vi "multipatch_states_V0.030_dualWCedits.vi"(0 "common cluster":T11, 1 "images":T8, 2 "allMainVIcontrols":refnum<vi>, 3 "which manipulator":T5(ring), 5 "individual controls in":T10, 7 "state in":T3=enum."Setting defaults...", 9 "cam size":i32[](array[numeric]), 11 "error in":errorcluster, 12 "time in":timestamp, 13 "mainVIpath":path) -> (15 "error out":errorcluster)   [LabVIEW 2015]
uses:
  controls/user_message_v6.ctl
  machine_vision/controls/approach_type.ctl
  controls/scope_motion.ctl
  multiBot/patcherBot/AxMultiClampMsg.dll
  whole_cell_protocol/Controls/Data.ctl
  pipette cleaning/pressure box/cleaning_soft/controls/arduino_pressure_setting.ctl
  controls/memtest_def.ctl
  <vilib>/vision/Image Controls.llb/IMAQ Image.ctl
  controls/images_controls.ctl
  controls/multipatch_common_controls_v4.ctl
  controls/multipatch_individual_controls_v5.ctl
  pipette cleaning/pressure box/cleaning_soft/controls/actuator_type.ctl
  pipette cleaning/pressure box/cleaning_soft/controls/actuator_cluster.ctl
  machine_vision/coordinate model vis/transform_properties_actuators.ctl
  machine_vision/controls/transform_cluster_actuator.ctl
  pipette cleaning/pressure box/cleaning_soft/controls/pressure_box_type.ctl
  pipette cleaning/pressure box/cleaning_soft/controls/pressure_box_control.ctl
  controls/NH_method.ctl
panel:
  out "cell number when cleaning fail 2":i32
  in  "protocol 2":enum16{"clean", "sham"}(ring)
  in  "Cleaning step (time [s], value [mBar]) actual 2":dbl[][](array[numeric])=[[3.0, -345.0], [1.0, -345.0], [1.0, 1000.0], [1.0, -345.0], [1.0, 1000.0], [1.0, -345.0], [1.0, 1000.0], [1.0, -345.0], [1.0, 1000.0], [5.0, 1000.0]]
  in  "Wash step (time [s], value [mBar]) actual 2":dbl[][](array[numeric])=[[2.0, -345.0], [10.0, 1000.0]]
  out "ValidationOutputCluster":T1(array[cluster])
  out "ValidationWaveform":waveform(dbl)[](array[waveform])
  out "ValidationPos2":T2(array[ring])
  out "ValidationPos1":T2(array[ring])
  out "ValidationResults":waveform(dbl)[][](array[waveform])
  in  "debug state":T3=enum."Detecting cell..."
  out "exit trigger":bool
  in  "Tab Control":T4(tab)
  out "max steps to take":i32
  in  "long wc protocol?":bool
  in  "GS memtest inputs":T6={"Samples to Read"=2000, "Rate (Hz)"=20000.0, "Amplitude (mV/pA)"=10.0, "Offset (mV/pA)"=0.0, "Frequency (Hz)"=10.0, "duty cycle (%)"=50.0, "phase"=0.0} {"phase" format="%.2p"; "duty cycle (%)" format="%0.2f"}
  in  "cell tracker movement options":T7={"step down by (steps)"=10.0, "descend threshold diam (px)"=30.0, "step XY by (steps)"=10.0} {"descend threshold diam (px)" format="%#_13g"; "step down by (steps)" format="%#_13g"}
  out "rel move vector (steps)":dbl[](array[numeric])
  in  "Wash step (time [s], value [mBar]) actual":dbl[][](array[numeric])=[[2.0, -345.0], [10.0, 1000.0]]
  in  "Cleaning step (time [s], value [mBar]) actual":dbl[][](array[numeric])=[[3.0, -345.0], [1.0, -345.0], [1.0, 1000.0], [1.0, -345.0], [1.0, 1000.0], [1.0, -345.0], [1.0, 1000.0], [1.0, -345.0], [1.0, 1000.0], [5.0, 1000.0]]
  in  "protocol":enum16{"clean", "sham"}(ring)
  out "cell number when cleaning fail":i32
  in  "give a zap?":i32[](array[numeric])=[0, 0, 1, 0, 1, 0, 0, 1, 0, 0, 1, 0, 1, 1]
  in  "Breakin num pulses":i32[](array[numeric])=[1, 1, 1, 1, 1, 1, 1, 1, 1, 1, 1, 1, 1, 1]
  in  "Breakin durations (ms)":i32[](array[numeric])=[0, 50, 50, 100, 100, 100, 200, 200, 200, 400, 500, 700, 1000, 1000]
  out "slow comp (pF)":dbl
  out "fast comp (pF)":dbl
  out "set pressure":dbl
  in  "AO physical channels":tag="Dev1/ao0:1"
  in  "AI Physical Channel":tag="Dev1/ai0:2, Dev1/ai10"
  out "state out":T3=enum."Setting defaults..."
  # "REENTRANT!!"
  # "VERSION CONTROL\n6/23/17\nmultiBot v0.007 is compatible with multipatch_states_v0.007\n- cell tracker working great\n- latest stable version for SINGLE-PATCH image tracking in slices\nmultiBot v0.006_reentrants is compatible with multipatch_states_wrapper_v0.001\nmultiBot v0.005 is compatible with multipatch_states_v0.005\nmultiBot v0.004 is compatible with multipatch_states_v0.004"
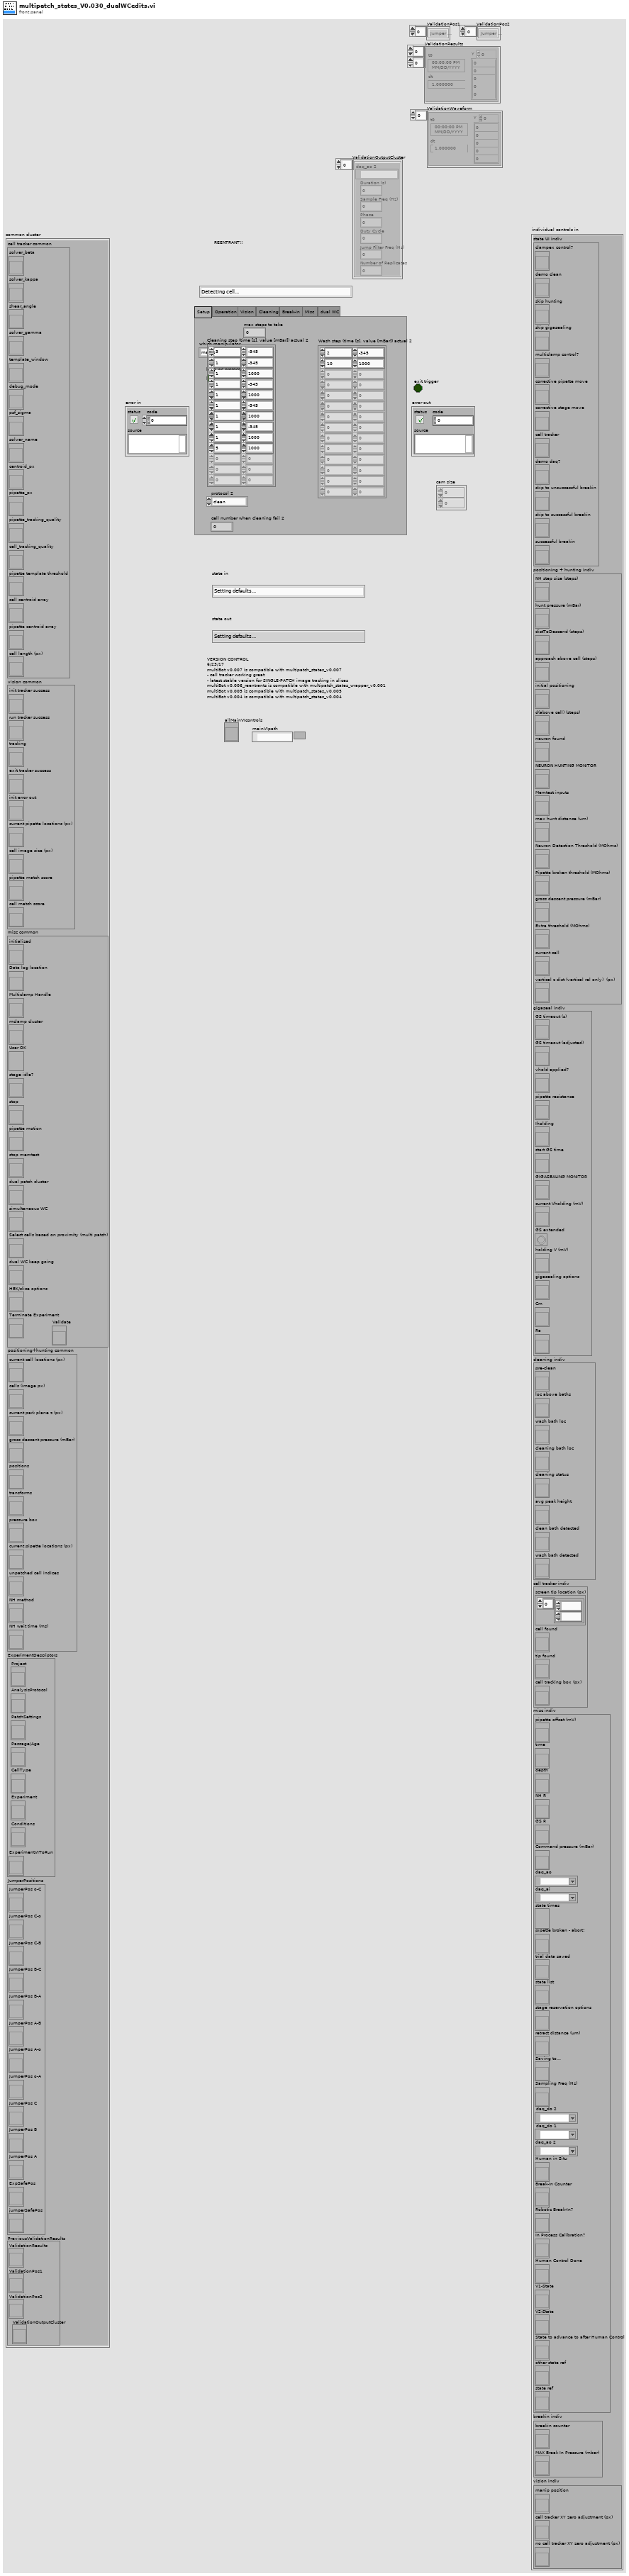
[diagram p1: front panel]
types:
  T1 = cluster{"daq_ao 2":tag, "Duration (s)":dbl, "Sample Freq (Hz)":dbl, "Phase":dbl, "Duty Cycle":dbl, "Jump Filter Freq (Hz)":dbl, "Number of Replicates":i16}[]
  T2 = enum16{"Jumper Safe Position", "Experiment Safe Position", "Jumper Position A", "Jumper Position B", "Jumper Position C", "Jumper Position o-A", "Jumper Position A-o", "Jumper Position A-B", "Jumper Position B-A", "Jumper Position B-C", "Jumper Position C-B", "Jumper Position C-o", "Jumper Position o-C"}[]
  T3 = typedef "user_message_v6.ctl" = enum16{"Initializing...", "Setting defaults...", "Click OK to start patcherBot!", "Starting new attempt...", "Pipette repositioning...", "Initializing cell tracker...", "Gross approach...", "Human Positioning...", "In Process Calibration", "Detecting cell...", "Cell detected...", "Gigaseal Established...", "Breaking in...", "Successful breakin!", "Unsuccessful breakin!", "Whole-cell recording", "Saving autopatching parameters...", "Quitting VI", "Waiting for idle stage...", "Cleaning...", "Retracting pipette...", "DEBUG STATE", "Waiting to break in...", "Waiting for WC", "reclean", "Done with Current Set of Cells"}
  T4 = enum32{"Setup", "Operation", "Vision", "Cleaning", "Break-in", "Misc", "dual WC"}
  T5 = enum16{"manipulator 1", "manipulator 2", "manipulator 3", "manipulator 4"}
  T6 = typedef "memtest_def.ctl" = cluster{"Samples to Read":i32, "Rate (Hz)":dbl, "Amplitude (mV/pA)":dbl, "Offset (mV/pA)":dbl, "Frequency (Hz)":dbl, "duty cycle (%)":dbl, "phase":dbl}
  T7 = cluster{"step down by (steps)":dbl, "descend threshold diam (px)":dbl, "step XY by (steps)":dbl}
  T8 = typedef "images_controls.ctl" = cluster{"slice image":T9, "pipette template":T9, "found pipette":T9, "pipette mask for cell tracker":T9, "cell images ref":refnum<vi>}
  T9 = typedef "IMAQ Image.ctl" = refnum<image>
  T10 = typedef "multipatch_individual_controls_v5.ctl" = cluster{"state UI indiv":cluster{"clampex control?":refnum<vi>, "demo clean":refnum<vi>, "skip hunting":refnum<vi>, "skip gigasealing":refnum<vi>, "multiclamp control?":refnum<vi>, "corrective pipette move":refnum<vi>, "corrective stage move":refnum<vi>, "cell tracker":refnum<vi>, "demo daq?":refnum<vi>, "skip to unsuccessful breakin":refnum<vi>, "skip to successful breakin":refnum<vi>, "successful breakin":refnum<vi>}, "positioning + hunting indiv":cluster{"NH step size (steps)":refnum<vi>, "hunt pressure (mBar)":refnum<vi>, "distToDescend (steps)":refnum<vi>, "approach above cell (steps)":refnum<vi>, "initial positioning":refnum<vi>, "d(above cell) (steps)":refnum<vi>, "neuron found":refnum<vi>, "NEURON HUNTING MONITOR":refnum<vi>, "Memtest inputs":refnum<vi>, "max hunt distance (um)":refnum<vi>, "Neuron Detection Threshold (MOhms)":refnum<vi>, "Pipette broken threshold (MOhms)":refnum<vi>, "gross descent pressure (mBar)":refnum<vi>, "Extra threshold (MOhms)":refnum<vi>, "current cell":refnum<vi>, "vertical z dist (vertical rel only)  (px)":refnum<vi>}, "gigaseal indiv":cluster{"GS timeout (s)":refnum<vi>, "GS timeout (adjusted)":refnum<vi>, "vhold applied?":refnum<vi>, "pipette resistance":refnum<vi>, "Iholding":refnum<vi>, "start GS time":refnum<vi>, "GIGASEALING MONITOR":refnum<vi>, "current Vholding (mV)":refnum<vi>, "GS extended":refnum<vi>, "holding V (mV)":refnum<vi>, "gigasealing options":refnum<vi>, "Cm":refnum<vi>, "Ra ":refnum<vi>}, "cleaning indiv":cluster{"pre-clean":refnum<vi>, "loc above baths":refnum<vi>, "wash bath loc":refnum<vi>, "cleaning bath loc":refnum<vi>, "cleaning status":refnum<vi>, "avg peak height":refnum<vi>, "clean bath detected":refnum<vi>, "wash bath detected":refnum<vi>}, "cell tracker indiv":cluster{"screen tip location (px)":refnum<vi>, "cell found":refnum<vi>, "tip found":refnum<vi>, "cell tracking box (px)":refnum<vi>}, "misc indiv":cluster{"pipette offset (mV)":refnum<vi>, "time":refnum<vi>, "depth":refnum<vi>, "NH R":refnum<vi>, "GS R":refnum<vi>, "Command pressure (mBar)":refnum<vi>, "daq_ao":tag, "daq_ai":tag, "state times":refnum<vi>, "pipette broken - abort!":refnum<vi>, "trial data saved":refnum<vi>, "state list":refnum<vi>, "stage reservation options":refnum<vi>, "retract distance (um)":refnum<vi>, "Saving to...":refnum<vi>, "Sampling Freq (Hz)":refnum<vi>, "daq_do 2":tag, "daq_do 1":tag, "daq_ao 2":tag, "Human in Situ":refnum<vi>, "Break-In Counter":refnum<vi>, "Robotic Break-In?":refnum<vi>, "In Process Calibration?":refnum<vi>, "Human Control Done":refnum<vi>, "V1-State":refnum<vi>, "V2-State":refnum<vi>, "State to advance to after Human Control":refnum<vi>, "other state ref":refnum<vi>, "state ref":refnum<vi>}, "breakin indiv":cluster{"breakin counter":refnum<vi>, "MAX Break In Pressure (mbar)":refnum<vi>}, "vision indiv":cluster{"manip position":refnum<vi>, "cell tracker XY zero adjustment (px)":refnum<vi>, "no cell tracker XY zero adjustment (px)":refnum<vi>}}
  T11 = typedef "multipatch_common_controls_v4.ctl" = cluster{"cell tracker common":cluster{"solver_beta":refnum<vi>, "solver_kappa":refnum<vi>, "shear_angle":refnum<vi>, "solver_gamma":refnum<vi>, "template_window":refnum<vi>, "debug_mode":refnum<vi>, "psf_sigma":refnum<vi>, "solver_name":refnum<vi>, "centroid_px":refnum<vi>, "pipette_px":refnum<vi>, "pipette_tracking_quality":refnum<vi>, "cell_tracking_quality":refnum<vi>, "pipette template threshold":refnum<vi>, "cell centroid array":refnum<vi>, "pipette centroid array":refnum<vi>, "cell length (px)":refnum<vi>}, "vision common":cluster{"init tracker success":refnum<vi>, "run tracker success":refnum<vi>, "tracking":refnum<vi>, "exit tracker success":refnum<vi>, "init error out":refnum<vi>, "current pipette locations (px)":refnum<vi>, "cell image size (px)":refnum<vi>, "pipette match score":refnum<vi>, "cell match score":refnum<vi>}, "misc common":cluster{"initialized":refnum<vi>, "Data log location":refnum<vi>, "Multiclamp Handle":refnum<vi>, "mclamp cluster":refnum<vi>, "User OK":refnum<vi>, "stage idle?":refnum<vi>, "stop":refnum<vi>, "pipette motion":refnum<vi>, "stop memtest":refnum<vi>, "dual patch cluster":refnum<vi>, "simultaneous WC":refnum<vi>, "Select cells based on proximity (multi patch)":refnum<vi>, "dual WC keep going":refnum<vi>, "HEK/slice options":refnum<vi>, "Terminate Experiment":refnum<vi>, "Validate":refnum<vi>}, "positioning+hunting common":cluster{"current cell locations (px)":refnum<vi>, "cells (image px)":refnum<vi>, "current park plane z (px)":refnum<vi>, "gross descent pressure (mBar)":refnum<vi>, "positions":refnum<vi>, "transforms":refnum<vi>, "pressure box":refnum<vi>, "current pipette locations (px)":refnum<vi>, "unpatched cell indices":refnum<vi>, "NH method":refnum<vi>, "NH wait time (ms)":refnum<vi>}, "ExperimentDescriptors":cluster{"Project":refnum<vi>, "AnalysisProtocol":refnum<vi>, "PatchSettings":refnum<vi>, "Passage/Age":refnum<vi>, "CellType":refnum<vi>, "Experiment":refnum<vi>, "Conditions":refnum<vi>, "ExperimentVIToRun":refnum<vi>}, "JumperPositions":cluster{"JumperPos o-C":refnum<vi>, "JumperPos C-o":refnum<vi>, "JumperPos C-B":refnum<vi>, "JumperPos B-C":refnum<vi>, "JumperPos B-A":refnum<vi>, "JumperPos A-B":refnum<vi>, "JumperPos A-o":refnum<vi>, "JumperPos o-A":refnum<vi>, "JumperPos C":refnum<vi>, "JumperPos B":refnum<vi>, "JumperPos A":refnum<vi>, "ExpSafePos":refnum<vi>, "jumperSafePos":refnum<vi>}, "PreviousValidationResults":cluster{"ValidationResults":refnum<vi>, "ValidationPos1":refnum<vi>, "ValidationPos2":refnum<vi>, "ValidationOutputCluster":refnum<vi>}}
  T12 = cluster{"Project":refnum<vi>, "AnalysisProtocol":refnum<vi>, "PatchSettings":refnum<vi>, "Passage/Age":refnum<vi>, "CellType":refnum<vi>, "Experiment":refnum<vi>, "Conditions":refnum<vi>, "ExperimentVIToRun":refnum<vi>}
  T13 = enum8{"Enabled", "Disabled", "Disabled and Grayed Out"}
  T14 = typedef "scope_motion.ctl" = enum16{"superSlow", "fast", "slow", "find slice speed", "slow_dualPatch"}
  T15 = typedef "approach_type.ctl" = enum16{"right to cell", "vertical abs", "approach", "vertical rel", "approach above"}
  T16 = typedef "Data.ctl" = cluster{"daq_ao 1":tag, "daq_ai 1":tag, "experiment day folder":path, "Multiclamp init error":i32, "Multiclamp Handle Out":u32, "sampling rate (Hz)":i32, "trial name":string}
  T17 = enum32{"Invalid", "Standard", "Closed", "Hidden", "Minimized", "Maximized"}
  T18 = enum16{"open", "replace", "create", "open or create", "replace or create", "replace or create with confirmation"}
  T19 = typedef "arduino_pressure_setting.ctl" = enum16{"High Positive Pressure", "Low Positive Pressure", "Atmospheric Pressure", "Low Vacuum", "High Vacuum", "Break In", "Puff"}
  T20 = cluster{"current stage pos (steps)":refnum<vi>, "current manip 1 pos (steps)":refnum<vi>, "current manip 2 pos (steps)":refnum<vi>, "current manip 3 pos (steps)":refnum<vi>, "current manip 4 pos (steps)":refnum<vi>}
  T21 = typedef "transform_cluster_actuator.ctl" = cluster{"s":refnum<vi>, "manip 1":refnum<vi>, "manip 2":refnum<vi>, "manip 3":refnum<vi>, "manip 4":refnum<vi>}
  T22 = typedef "pressure_box_control.ctl" = cluster{"Pressure box COM":refnum<visa-resource-name>, "pressure box type":T23, "High pos pressure (mBar)":dbl, "Low pos pressure (mBar)":dbl, "Vacuum pressure (mBar)":dbl, "calibration":enum16{"PA_vacPump", "PA_venturi", "Neuromatics", "ilyaRig", "mightenRig"}}
  T23 = typedef "pressure_box_type.ctl" = enum16{"Neuromatics", "ProportionAir", "Demo box", "N-ProportionAir"}
  T24 = typedef "transform_properties_actuators.ctl" = cluster{"theta (deg)":dbl, "X sc factor (px/step)":dbl, "Y sc factor (px/step)":dbl, "zero loc (x,y,z)":dbl[], "flip y?":bool, "flip x?":bool, "gamma (deg)":dbl, "flip z?":bool, "Z sc factor (px/step)":dbl, "actuator":T25, "safe space (steps)":i32[]}
  T25 = typedef "actuator_cluster.ctl" = cluster{"Actuator COM":refnum<visa-resource-name>, "Actuator type":T26}
  T26 = typedef "actuator_type.ctl" = enum16{"Scientifica", "Sutter", "Demo", "Off"}
  T27 = cluster{"clampex control?":refnum<vi>, "demo clean":refnum<vi>, "skip hunting":refnum<vi>, "skip gigasealing":refnum<vi>, "multiclamp control?":refnum<vi>, "corrective pipette move":refnum<vi>, "corrective stage move":refnum<vi>, "cell tracker":refnum<vi>, "demo daq?":refnum<vi>, "skip to unsuccessful breakin":refnum<vi>, "skip to successful breakin":refnum<vi>, "successful breakin":refnum<vi>}
  T28 = typedef "Image Type" = u32
  T29 = cluster{u32, string, i32, u32, u32, u32, "arg1":i32}
  T30 = cluster{"width x":dbl, "height y":dbl, "x offset":dbl, "y offset":dbl}
  T31 = cluster{"solver_beta":refnum<vi>, "solver_kappa":refnum<vi>, "shear_angle":refnum<vi>, "solver_gamma":refnum<vi>, "template_window":refnum<vi>, "debug_mode":refnum<vi>, "psf_sigma":refnum<vi>, "solver_name":refnum<vi>, "centroid_px":refnum<vi>, "pipette_px":refnum<vi>, "pipette_tracking_quality":refnum<vi>, "cell_tracking_quality":refnum<vi>, "pipette template threshold":refnum<vi>, "cell centroid array":refnum<vi>, "pipette centroid array":refnum<vi>, "cell length (px)":refnum<vi>}
  T32 = cluster{"init tracker success":refnum<vi>, "run tracker success":refnum<vi>, "tracking":refnum<vi>, "exit tracker success":refnum<vi>, "init error out":refnum<vi>, "current pipette locations (px)":refnum<vi>, "cell image size (px)":refnum<vi>, "pipette match score":refnum<vi>, "cell match score":refnum<vi>}
  T33 = enum16{"unreserve after gross approach", "unreserve after cell found"}
  T34 = typedef "NH_method.ctl" = enum16{"five-step", "three-stepANDfixedCutOff", "three-step"}
  T35 = cluster{"atm wait (indices)":i32, "num samples for slope":i32, "delta suction (mbar)":dbl, "if less than this slope, increase suction":dbl, "else if less than this slope, maintain suction":dbl, "else if less than this slope, decrease suction ":dbl, "max suction (mBar)":dbl}
  T36 = cluster{"GS timeout (s)":refnum<vi>, "GS timeout (adjusted)":refnum<vi>, "vhold applied?":refnum<vi>, "pipette resistance":refnum<vi>, "Iholding":refnum<vi>, "start GS time":refnum<vi>, "GIGASEALING MONITOR":refnum<vi>, "current Vholding (mV)":refnum<vi>, "GS extended":refnum<vi>, "holding V (mV)":refnum<vi>, "gigasealing options":refnum<vi>, "Cm":refnum<vi>, "Ra ":refnum<vi>}
  T37 = enum16{"manipulator 1", "manipulator 2", "manipulator 3", "manipulator 4"}[]
  T38 = typedef "dual_patch_controls.ctl" = cluster{"sampling rate (Hz)":dbl, "total duration (s)":dbl, "stim amplitude (pA)":dbl, "time between stims (s)":dbl, "delta t (s)":dbl, "pulse width (s)":dbl, "# repetitions":dbl, "number of pulses":i32, "before stim (s)":dbl}
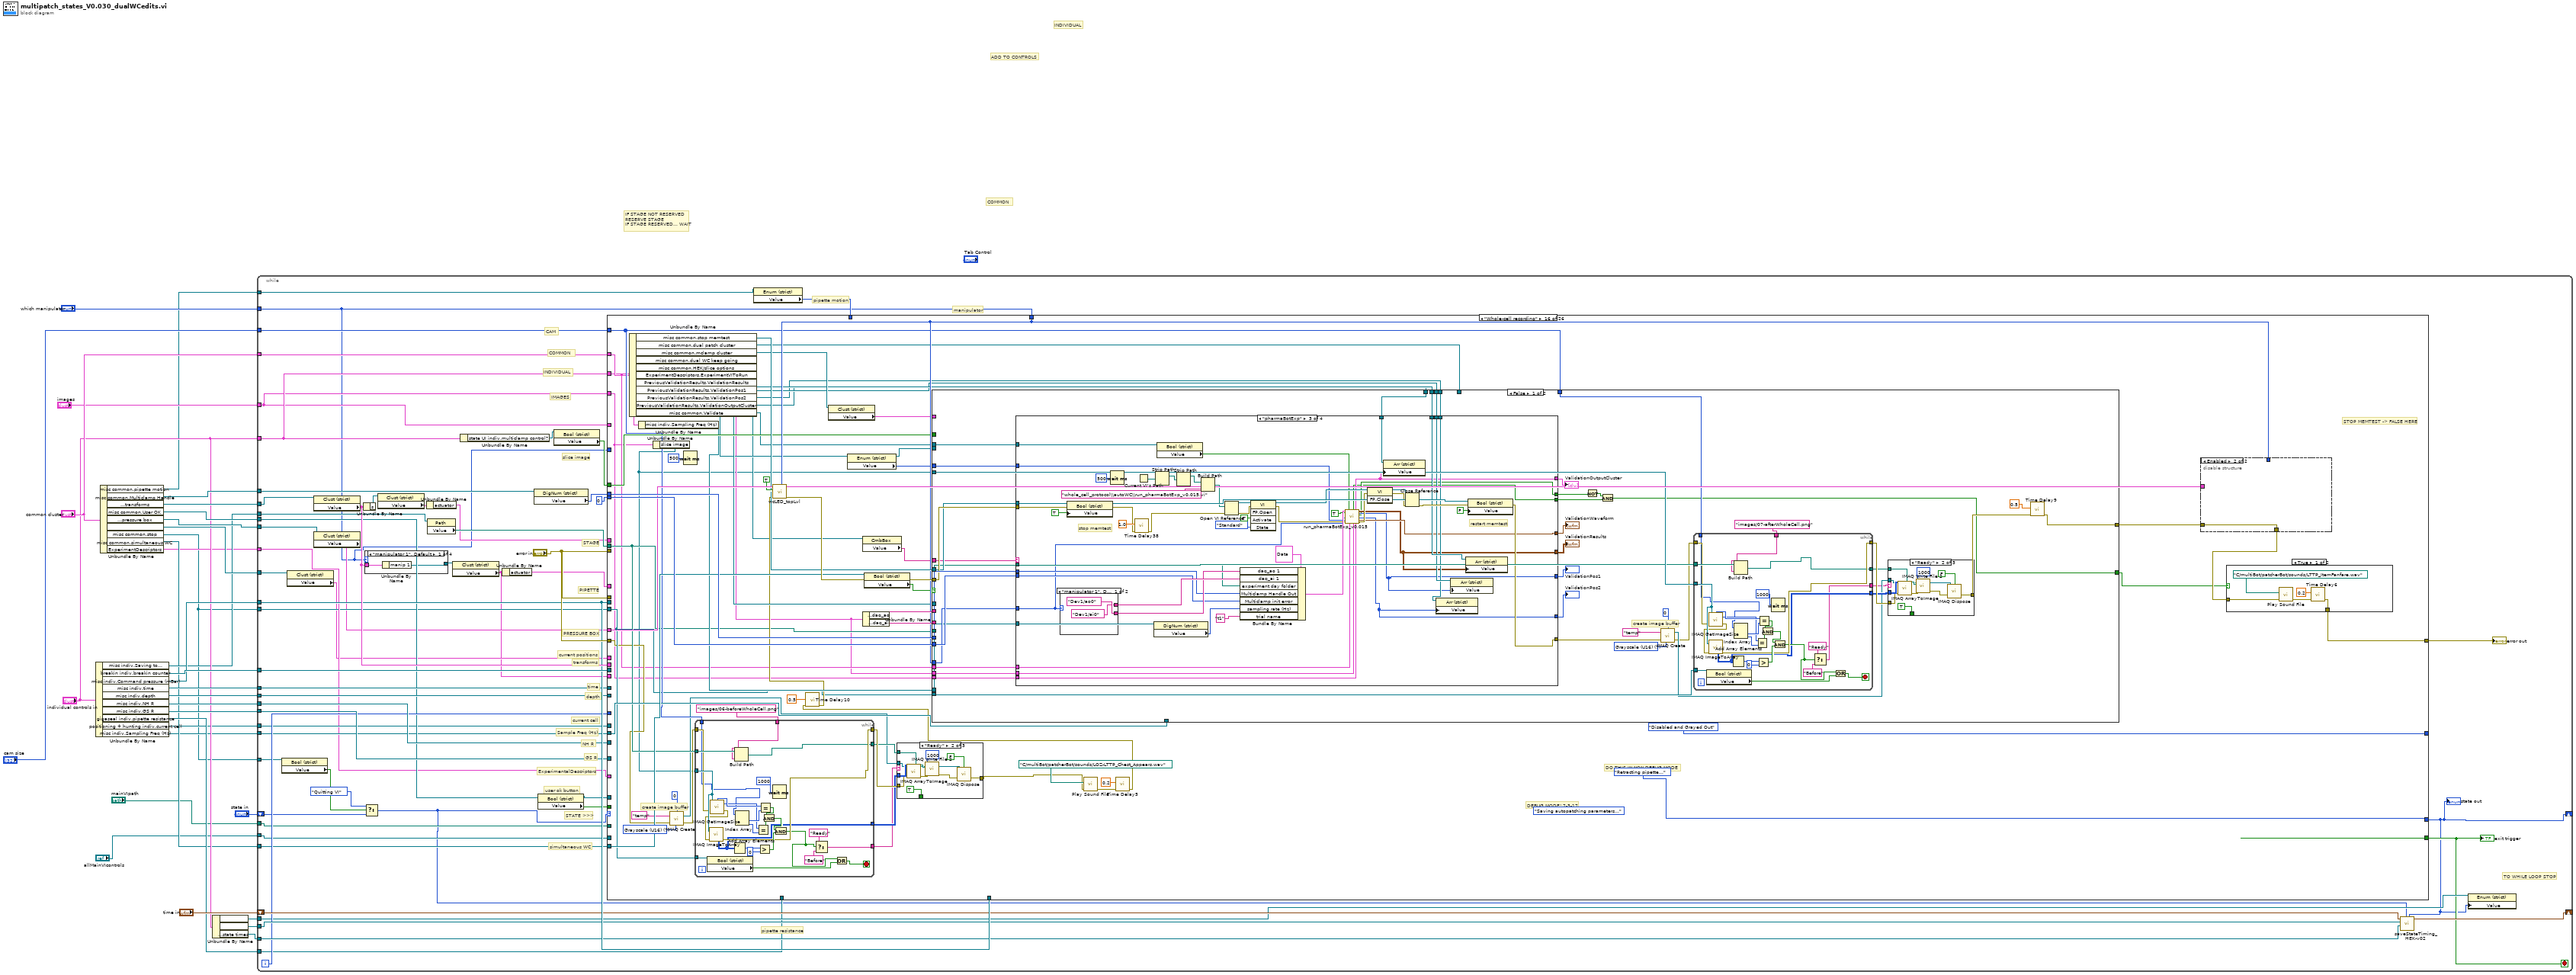
[diagram p0: block diagram]
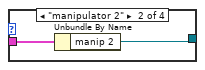
[diagram p2: hidden frame]
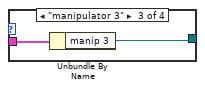
[diagram p3: hidden frame]
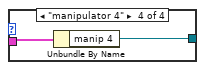
[diagram p4: hidden frame]
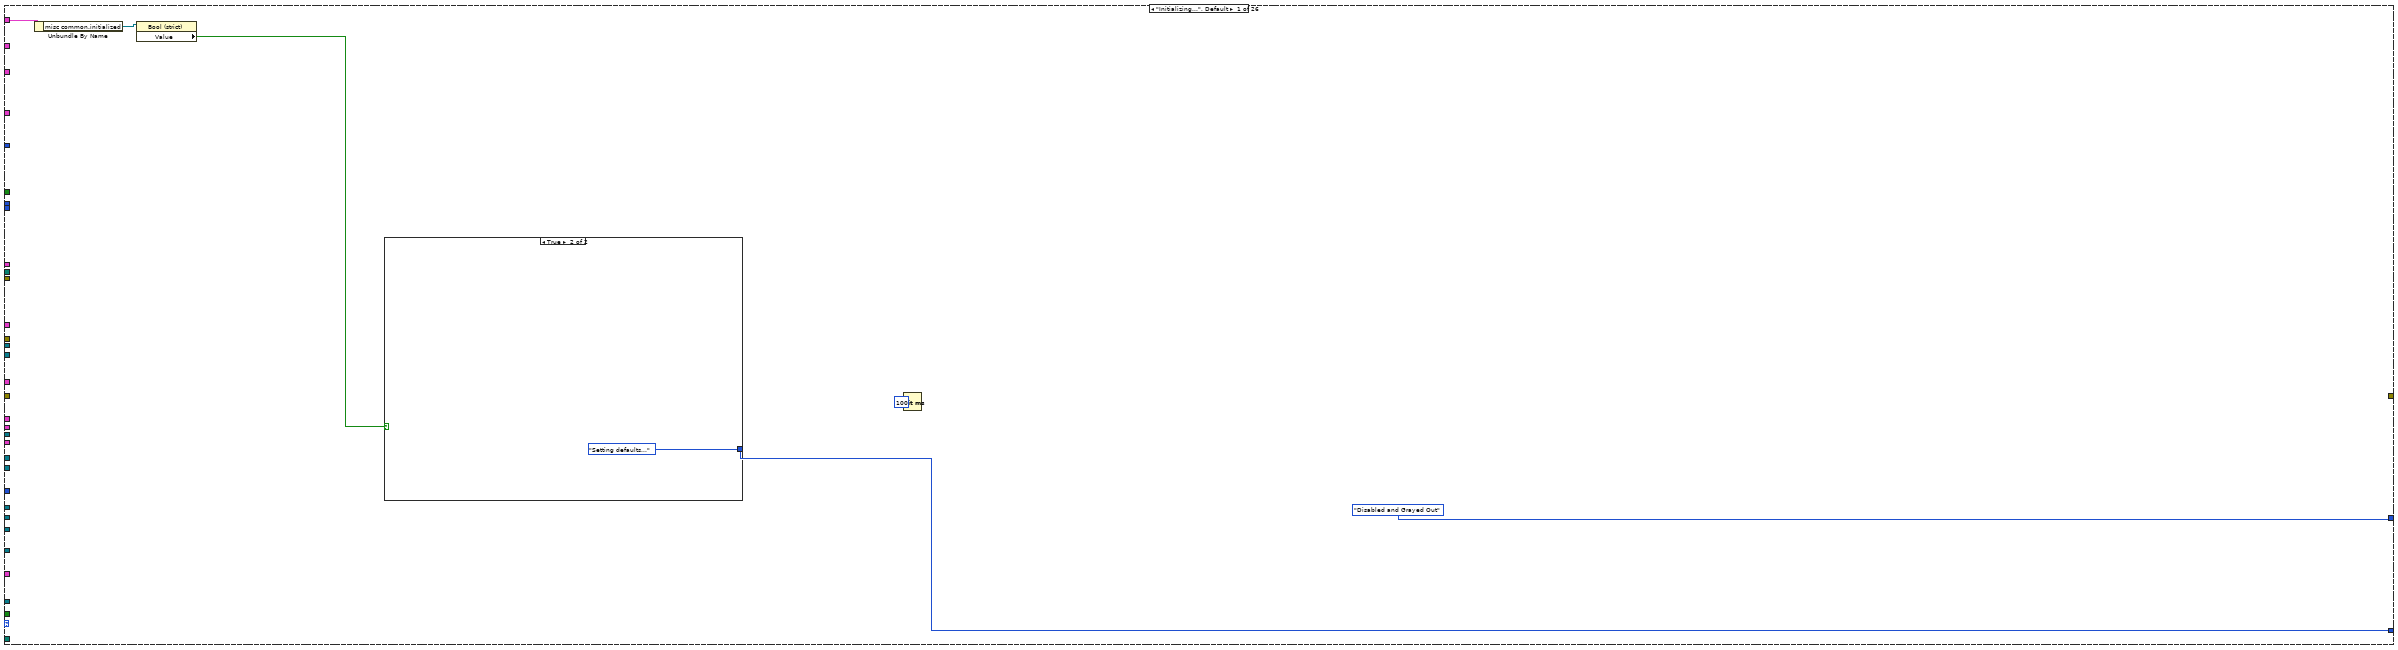
[diagram p5: hidden frame]
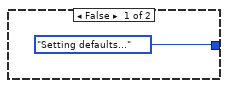
[diagram p6: hidden frame]
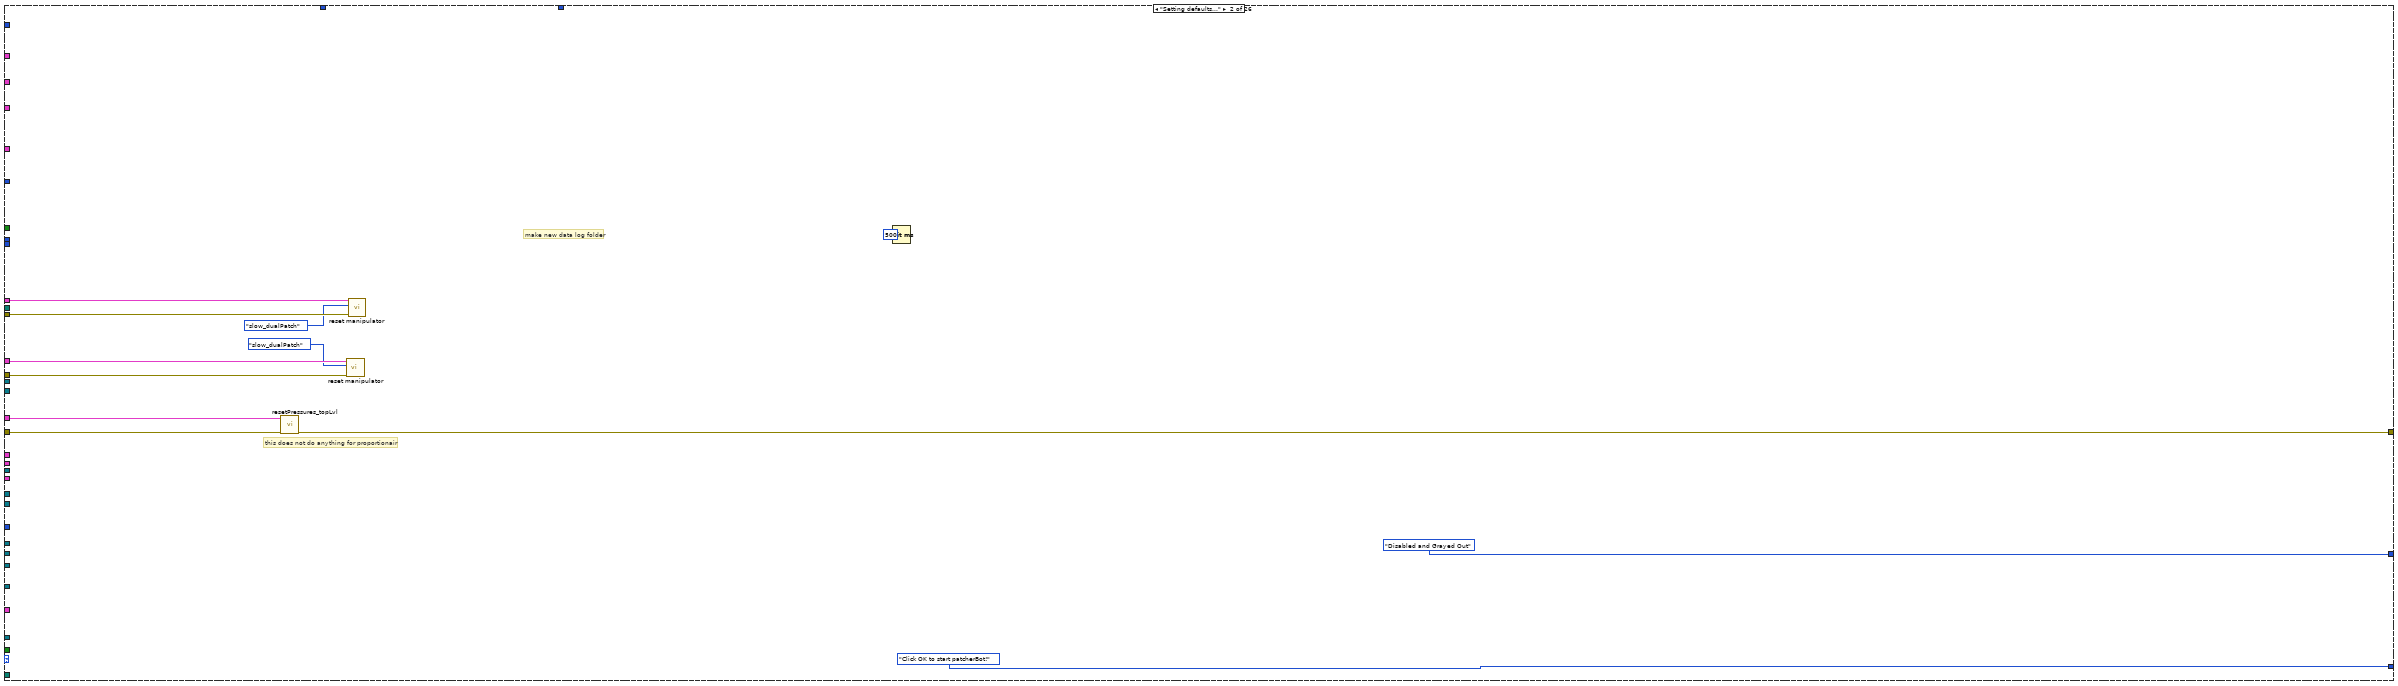
[diagram p7: hidden frame]
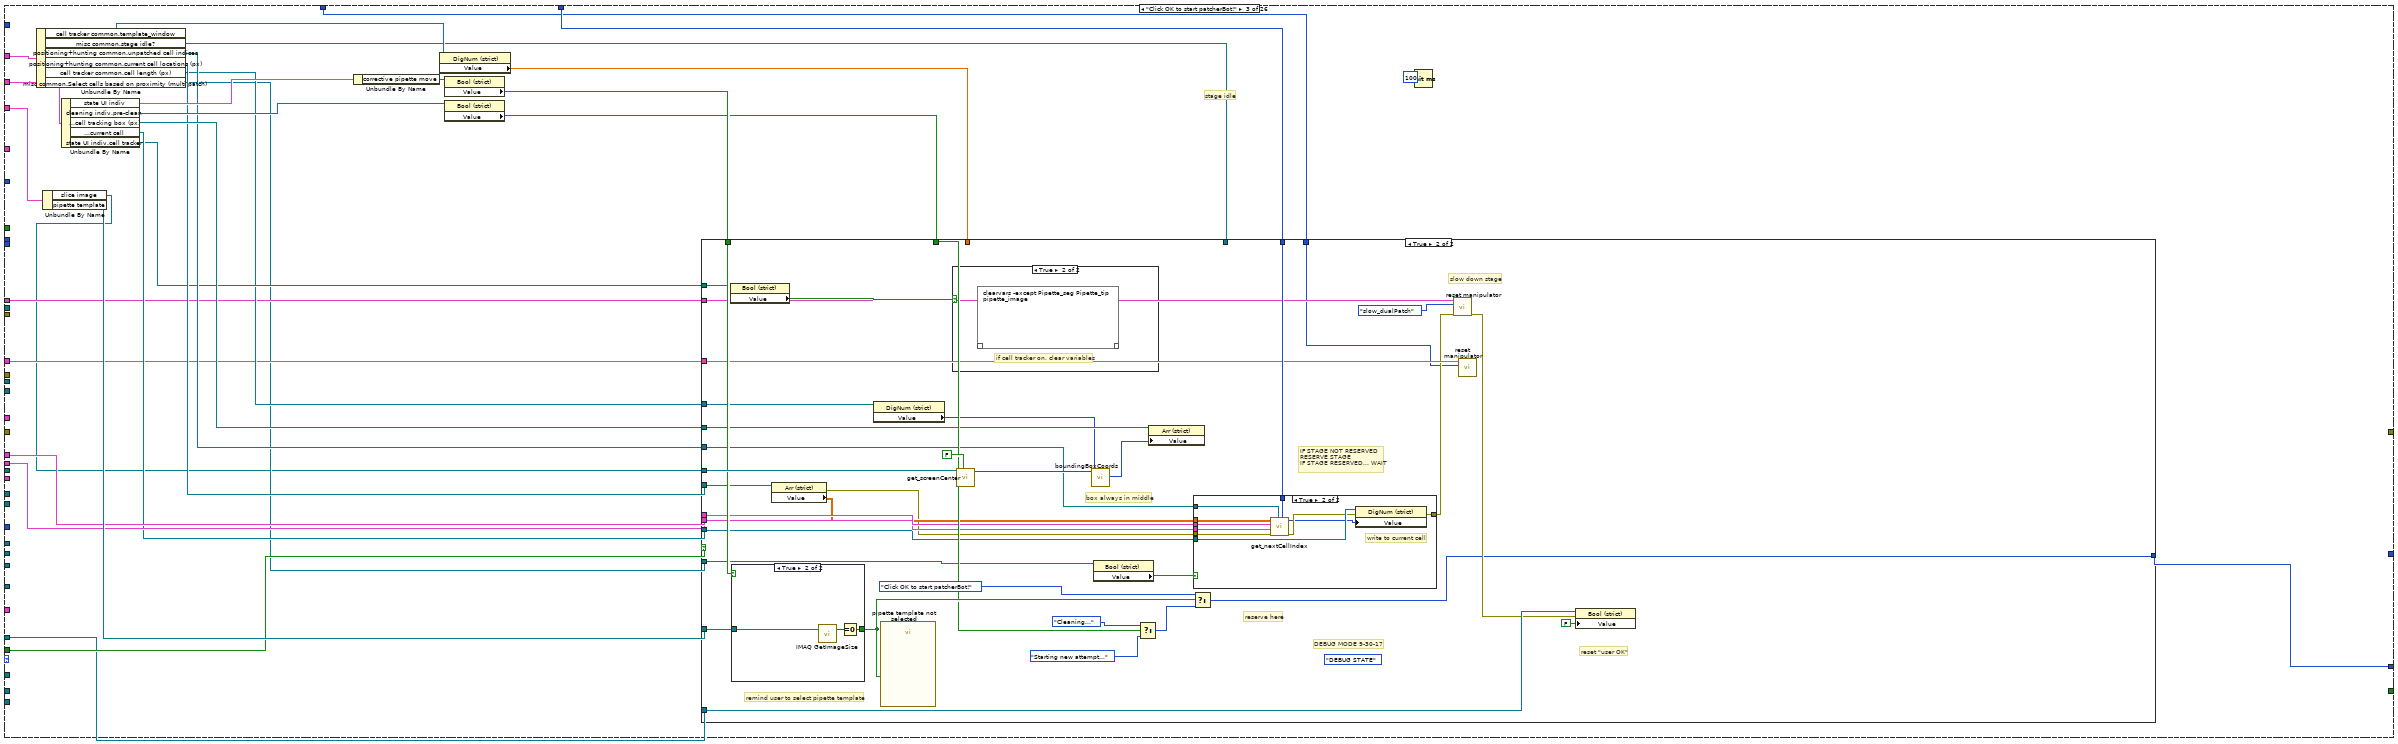
[diagram p8: hidden frame]
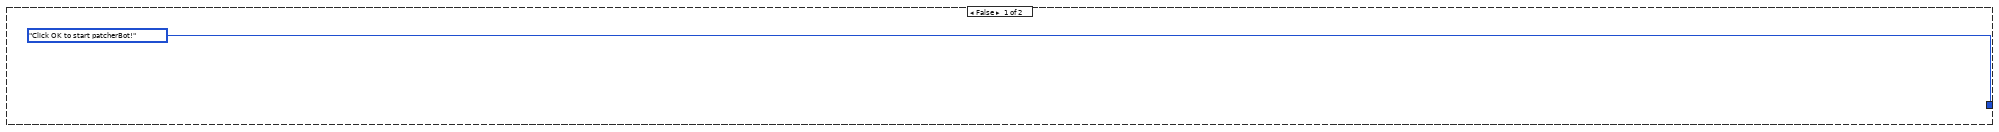
[diagram p9: hidden frame]
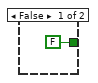
[diagram p12: hidden frame]
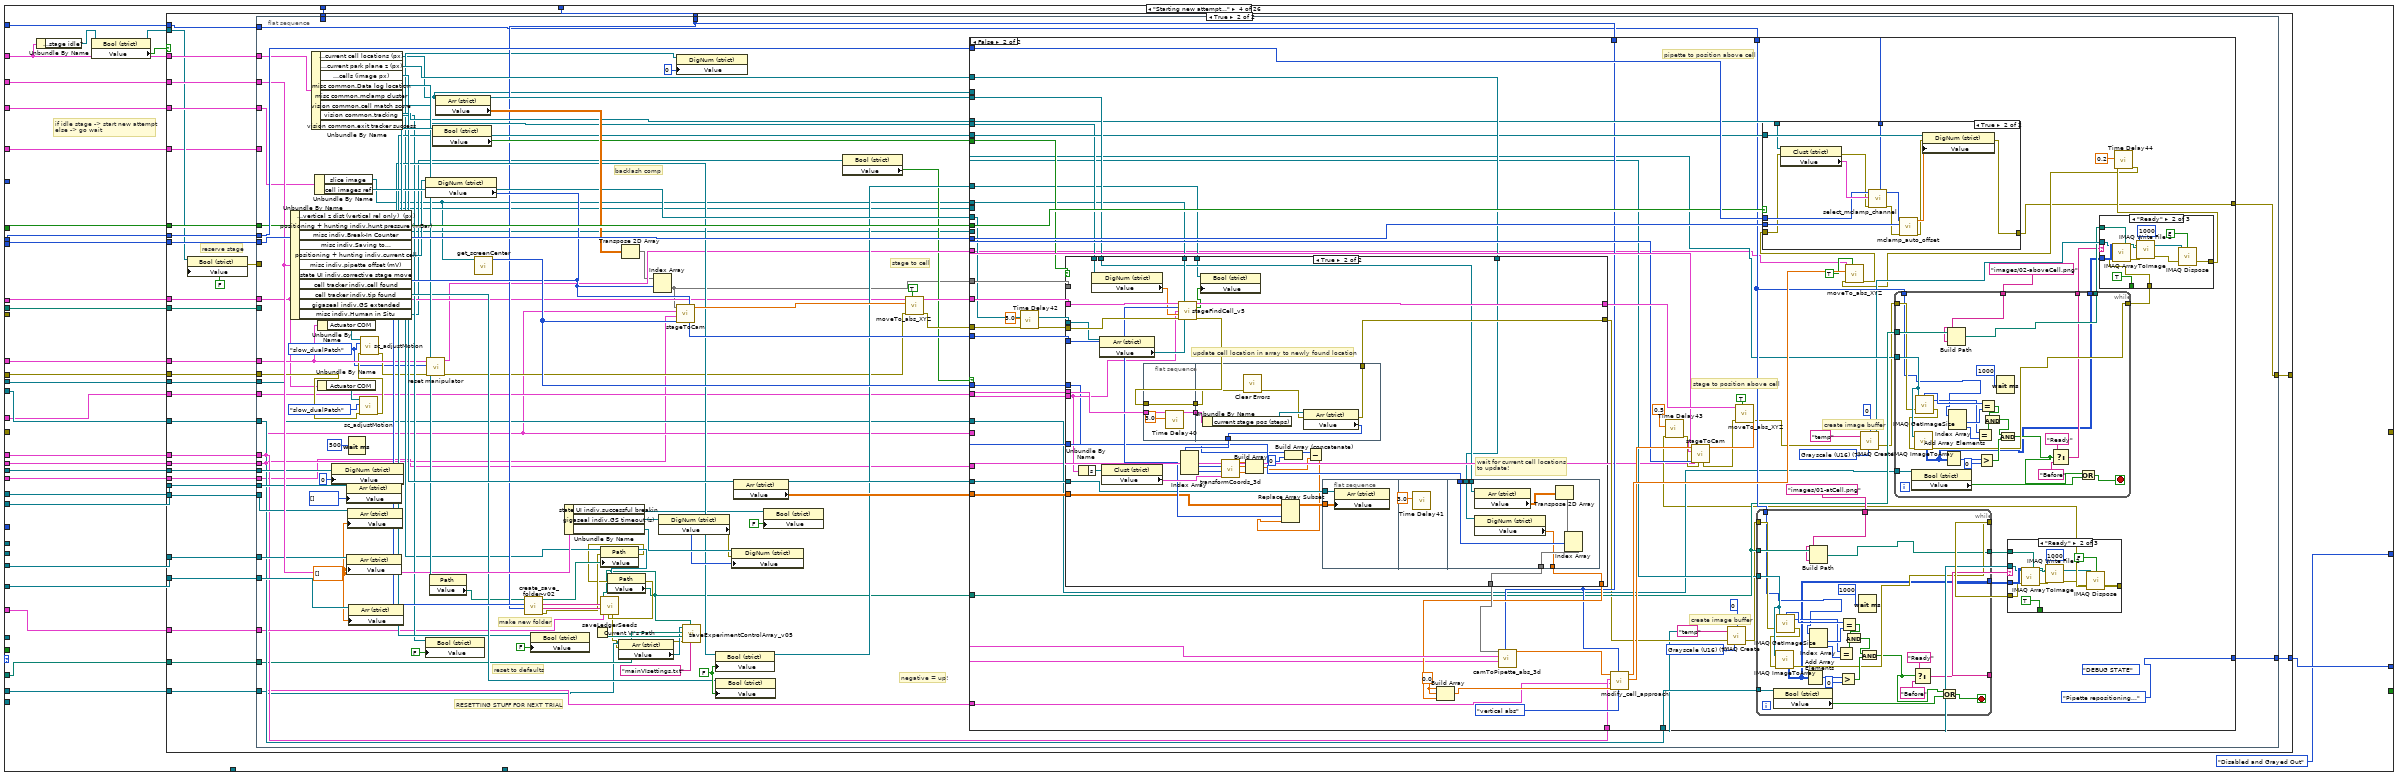
[diagram p13: hidden frame]
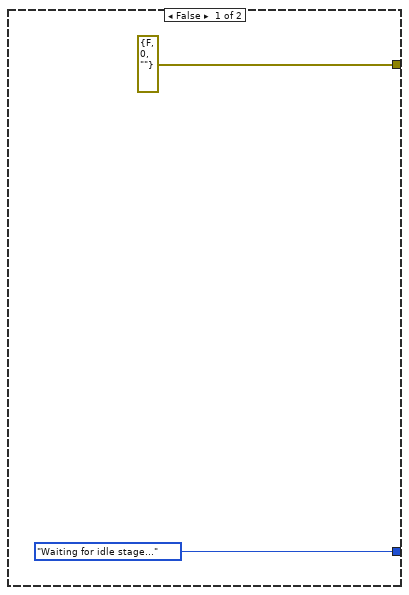
[diagram p14: hidden frame]
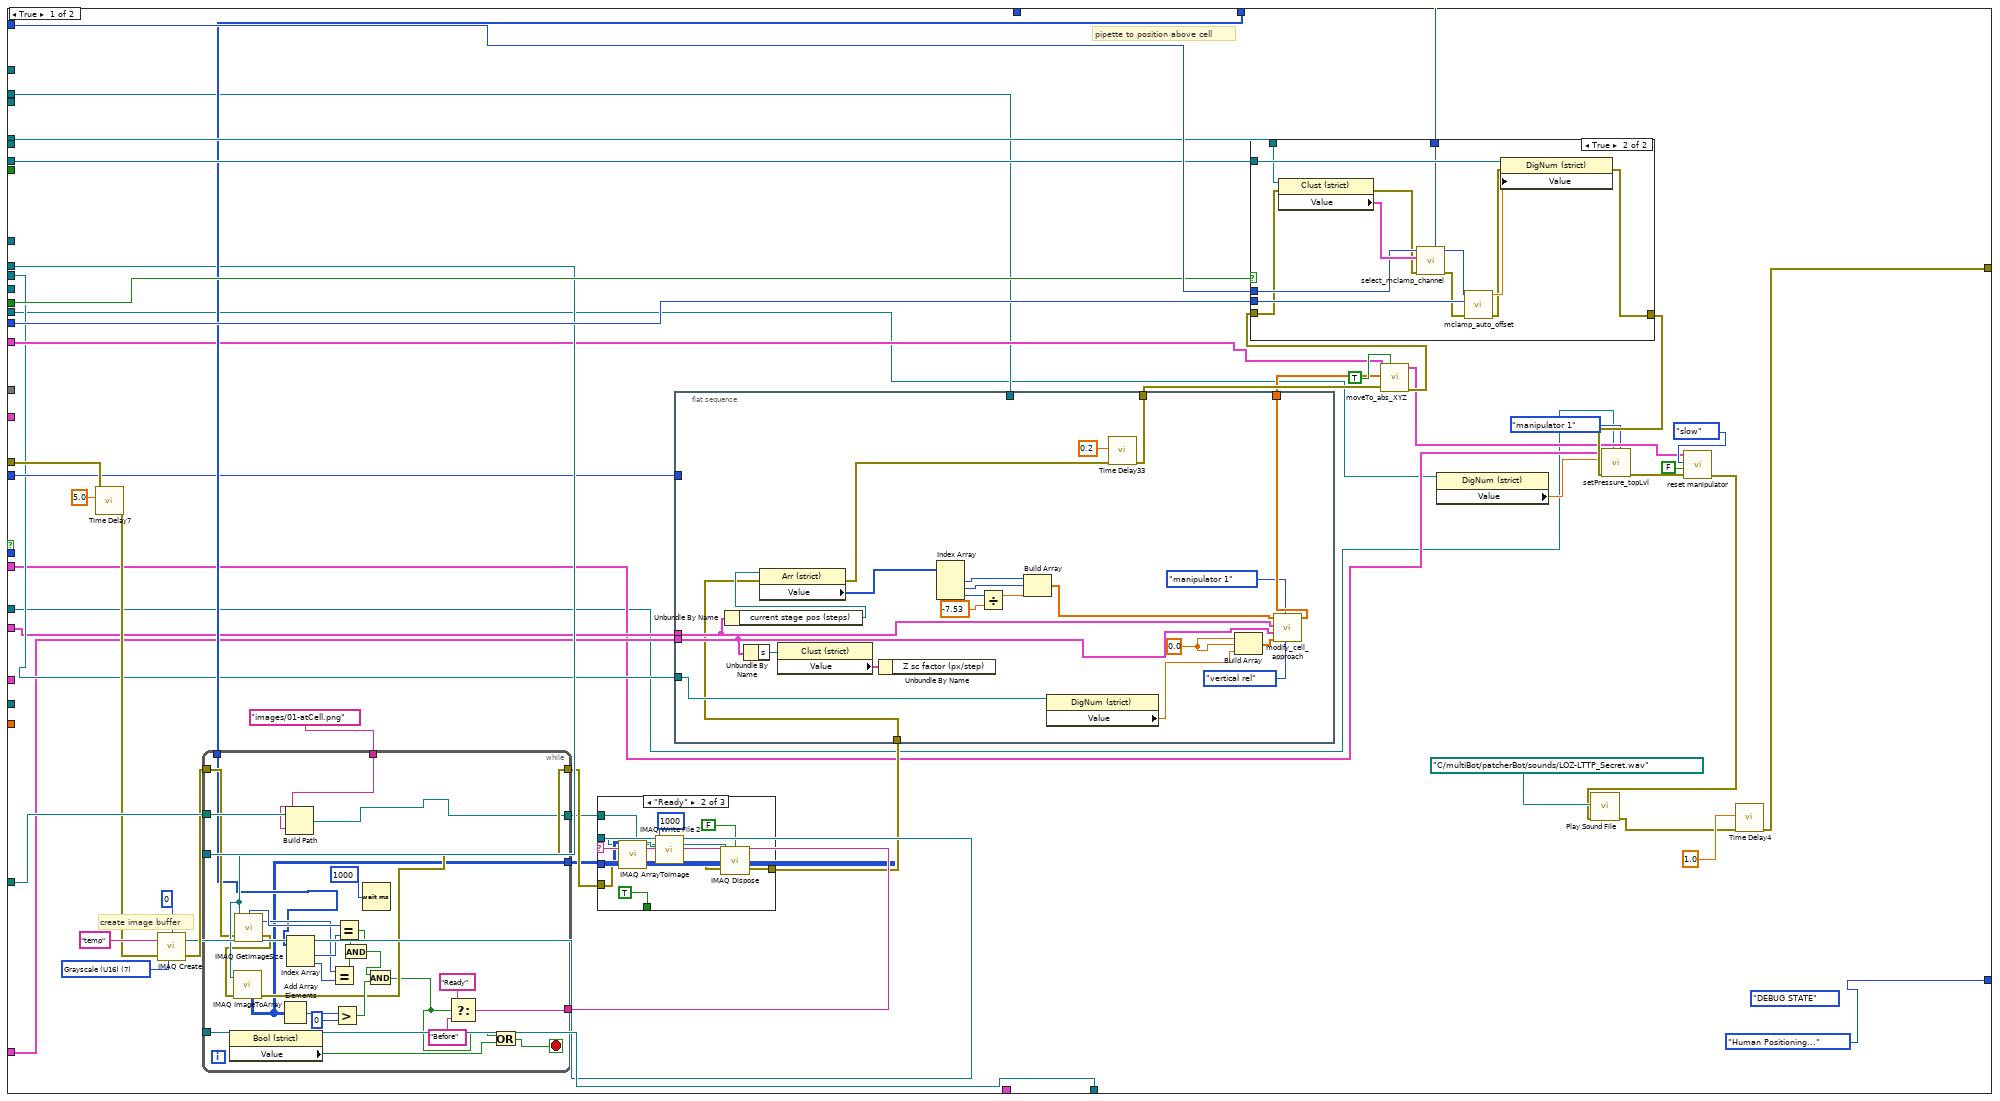
[diagram p15: hidden frame]
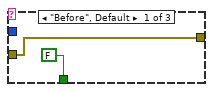
[diagram p16: hidden frame]
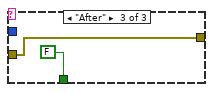
[diagram p17: hidden frame]
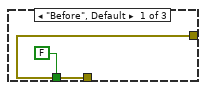
[diagram p19: hidden frame]
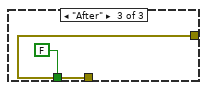
[diagram p20: hidden frame]
diagram:
  # "IF STAGE NOT RESERVED\nRESERVE STAGE\nIF STAGE RESERVED... WAIT"
  # "COMMON"
  # "INDIVIDUAL"
  # "ADD TO CONTROLS"
  n1 = Unbundle By Name("individual controls in") -> ("misc indiv.Saving to..."=w11:refnum<vi>, "breakin indiv.breakin counter"=w25:refnum<vi>, "misc indiv.Command pressure (mBar)"=w21:refnum<vi>, "misc indiv.time"=w19:refnum<vi>, "misc indiv.depth"=w18:refnum<vi>, "misc indiv.NH R"=w17:refnum<vi>, "misc indiv.GS R"=w16:refnum<vi>, "gigaseal indiv.pipette resistance"=w23:refnum<vi>, "positioning + hunting indiv.current cell"=w9:refnum<vi>, "misc indiv.Sampling Freq (Hz)"=w8:refnum<vi>)
  n2 = Unbundle By Name("common cluster") -> ("misc common.pipette motion"=w4:refnum<vi>, "misc common.Multiclamp Handle"=w26:refnum<vi>, "positioning+hunting common.transforms"=w30:refnum<vi>, "misc common.User OK"=w22:refnum<vi>, "positioning+hunting common.pressure box"=w28:refnum<vi>, "positioning+hunting common.positions"=w27:refnum<vi>, "misc common.stop"=w6:refnum<vi>, "misc common.simultaneous WC"=w10:refnum<vi>, "ExperimentDescriptors"=w7:T12)
  n3 = Unbundle By Name("individual controls in") -> ("misc indiv.state ref"=w12:refnum<vi>, "misc indiv.state list"=w14:refnum<vi>, "misc indiv.state times"=w13:refnum<vi>)
  n4 = while {
    tunnel: w30 -> [w88]
    tunnel: "which manipulator" -> [w32]
    tunnel: w28 -> [w84]
    tunnel: w27 -> [w80]
    tunnel: w26 -> [w79]
    tunnel: w25 -> [w75]
    tunnel: "common cluster" -> [w74]
    tunnel: "individual controls in" -> [w73]
    tunnel: w23 -> [w50]
    tunnel: w22 -> [w57]
    tunnel: w21 -> [w71]
    tunnel: "images" -> [w39]
    tunnel: w19 -> [w69]
    tunnel: w18 -> [w68]
    tunnel: w17 -> [w67]
    tunnel: w16 -> [w66]
    tunnel: w11 -> [w65]
    shift-right: [w62] -> _
    shift-left: "time in" -> [w63]
    tunnel: w14 -> [w61]
    tunnel: w13 -> [w60]
    tunnel: w12 -> [w58]
    tunnel: w6 -> [w54]
    tunnel: w4 -> [w52]
    tunnel: w10 -> [w49]
    tunnel: w9 -> [w48]
    tunnel: w8 -> [w47]
    tunnel: w7 -> [w46]
    tunnel: w6 -> [w45]
    tunnel: "cam size" -> [w44]
    tunnel: "mainVIpath" -> [w38]
    tunnel: "allMainVIcontrols" -> [w37]
    shift-right: [w33] -> _
    shift-left: "state in" -> [w36]
    i -> [w59]
    stop <- w43 stop-if-true
    # "CAM"
    # "ExperimentalDescriptors"
    # "Sample Freq (Hz)"
    # "current cell"
    # "simultaneous WC"
    # "pipette resistance"
    # "pipette motion"
    # "user ok button"
    # "TO WHILE LOOP STOP"
    # "IMAGES"
    # "INDIVIDUAL"
    # "COMMON"
    # "manipulator"
    # "slice image"
    # "transforms"
    # "current positions"
    # "STAGE"
    # "PRESSURE BOX"
    # "PIPETTE"
    # "STATE >>>"
    # "GS R"
    # "depth"
    # "time"
    # "NH R"
    n5 = property class="Bool (strict)"(reference=w54) -> ("Value"=w53:bool)  [unwired: 1 in, 2 out]
    n6 = property class="Clust (strict)"(reference=w80) -> ("Value"=w41:T20)  [unwired: 1 in, 2 out]
    n7 = property class="Clust (strict)"(reference=w88) -> ("Value"=w81:T21)  [unwired: 1 in, 2 out]
    n8 = property class="Clust (strict)"(reference=w84) -> ("Value"=w42:T22)  [unwired: 1 in, 2 out]
    n9 = Unbundle By Name(w81) -> ("s"=w72:refnum<vi>)
    n10 = case shown="\"manipulator 1\", Default" w32 {
      tunnel: w81 -> [w91 w93 w95 w97]
      tunnel: [w90 w92 w94 w96] -> w85
      frame "manipulator 1", Default {
        n11 = Unbundle By Name(w91) -> ("manip 1"=w90:refnum<vi>)
      }
      frame "manipulator 2" {
        n12 = Unbundle By Name(w93) -> ("manip 2"=w92:refnum<vi>)
      }
      frame "manipulator 3" {
        n13 = Unbundle By Name(w95) -> ("manip 3"=w94:refnum<vi>)
      }
      frame "manipulator 4" {
        n14 = Unbundle By Name(w97) -> ("manip 4"=w96:refnum<vi>)
      }
    }
    n15 = Select(t=user_message_v6."Quitting VI" ("state in"), s=w53, f=w36) -> (s? t:f=w34:T3)
    n16 = property class="Clust (strict)"(reference=w72) -> ("Value"=w87:T24)  [unwired: 1 in, 2 out]
    n17 = Unbundle By Name(w87) -> ("actuator"=w86:T25)
    n18 = property class="Path"(reference=w65) -> ("Value"=w89:path)  [unwired: 1 in, 2 out]
    n19 = property class="Clust (strict)"(reference=w85) -> ("Value"=w40:T24)  [unwired: 1 in, 2 out]
    n20 = Unbundle By Name(w73) -> ("state UI indiv.multiclamp control?"=w83:refnum<vi>)
    n21 = Unbundle By Name(w40) -> ("actuator"=w70:T25)
    n22 = property class="DigNum (strict)"(reference=w79) -> ("Value"=w78:u32)  [unwired: 1 in, 2 out]
    n23 = property class="Bool (strict)"(reference=w57) -> (reference out=w55:refnum<vi>, "Value"=w56:bool)  [unwired: 1 in, 1 out]
    n24 = property class="Bool (strict)"(reference=w83) -> ("Value"=w82:bool)  [unwired: 1 in, 2 out]
    n25 = property class="Enum (strict)"(reference=w52) -> ("Value"=w51:T14)  [unwired: 1 in, 2 out]
    n26 = case shown="\"Whole-cell recording\"" w34 {
      tunnel: w59 -> [_ _ _ _ _ _ _ w1247 _ w1347 w1660 _ _ _ _ _ _ _ _ _ _ _ _ w3350 _ _]
      tunnel: [w103 user_message_v6."Click OK to start patcherBot!" ("Message to user") w147 w232 user_message_v6."Initializing cell tracker..." ("Message to user") user_message_v6."Gross approach..." ("Message to user") w1112 w1256 w1290 w1308 w1653 w1770 w1938 w1990 user_message_v6."Retracting pipette..." ("Message to user") user_message_v6."Retracting pipette..." ("f") w2556 user_message_v6."Quitting VI" ("Message to user") w2660 w2770 w3010 user_message_v6."Saving autopatching parameters..." ("Message to user") w3318 w3335 w3364 _] -> w33
      tunnel: [T13."Disabled and Grayed Out" ("Disabled") T13."Disabled and Grayed Out" ("Disabled") _ T13."Disabled and Grayed Out" ("Disabled") T13."Disabled and Grayed Out" ("Disabled") _ _ _ _ T13."Disabled and Grayed Out" ("Disabled") w1659 T13."Disabled and Grayed Out" ("Disabled") T13."Disabled and Grayed Out" ("Disabled") T13."Disabled and Grayed Out" ("Disabled") T13."Disabled and Grayed Out" ("Disabled") T13."Disabled and Grayed Out" ("Disabled") T13."Disabled and Grayed Out" ("Disabled") T13."Disabled and Grayed Out" ("Disabled") _ _ _ T13."Disabled and Grayed Out" ("Disabled") _ _ _ _] -> _
      tunnel: w42 -> [_ w112 _ w206 w835 _ w1111 _ _ _ w1655 w1769 w1926 w1989 _ w2066 _ w2652 _ w2773 w3013 w3186 _ _ w3359 _]
      tunnel: "error in" -> [_ w111 _ _ _ _ _ _ _ _ _ w1733 w1891 _ _ w2035 _ w2651 _ _ _ w3185 _ _ _ _]
      tunnel: "error in" -> [_ w113 _ w227 w771 _ _ _ _ w1346 _ _ _ _ _ _ _ w2653 _ w2753 w2995 _ _ _ _ _]
      tunnel: [_ w110 _ _ w777 _ w1061 _ _ w1303 _ w1768 w1919 _ _ w2015 w2499 w2650 _ w2749 w2993 w3221 _ _ _ _] -> w64
      tunnel: w78 -> [_ _ _ w231 _ _ _ _ _ _ w1656 w1766 w1900 _ _ w2070 _ _ _ w2771 w3011 w3220 _ _ _ _]
      tunnel: 0 ("Error out") -> [_ _ _ w230 _ _ _ _ _ _ w1657 w1765 w1934 _ _ w2069 _ _ _ _ _ w3219 _ _ _ _]
      tunnel: w89 -> [_ _ _ w210 w753 _ w1072 _ _ w1307 _ w1743 _ _ _ w2041 w2484 _ _ _ _ w3168 _ _ _ _]
      tunnel: [_ _ _ _ _ _ _ _ _ _ _ _ _ _ _ _ w2508 TRUE _ _ _ _ _ _ _ _] -> w43
      tunnel: w82 -> [_ _ _ w229 _ _ _ _ _ _ w1658 w1767 w1935 _ _ w2055 _ _ _ _ _ w3210 _ _ _ _]
      tunnel: w86 -> [_ w109 w122 w226 w833 _ _ _ _ w1343 _ _ _ _ _ _ _ w2644 _ _ _ _ _ _ _ _]
      tunnel: "error in" -> [_ w108 _ _ _ _ w1068 _ _ w1344 _ _ _ _ _ _ _ w2643 _ _ _ _ _ _ _ _]
      tunnel: w71 -> [_ _ _ _ _ _ _ _ _ _ w1654 _ _ _ _ _ _ _ _ w2772 w3012 _ _ _ _ _]
      tunnel: w70 -> [_ w114 w121 w228 w769 _ w1113 _ _ w1342 _ _ _ _ _ _ _ w2649 _ w2750 w2904 w3194 _ _ _ _]
      tunnel: w71 -> [_ _ _ w205 w834 _ w1109 _ _ _ _ w1763 w1913 _ _ _ _ w2648 _ _ _ w3181 _ _ _ _]
      tunnel: w41 -> [_ _ w131 w225 w827 _ w1117 _ _ w1341 _ _ _ _ _ _ w2523 _ _ _ _ _ _ _ _ _]
      tunnel: w81 -> [_ _ w130 w224 w785 _ w1114 _ _ w1340 _ _ _ _ _ _ w2522 _ _ w2763 w2901 w3202 _ _ _ _]
      tunnel: w32 -> [_ _ w129 w217 w784 _ w1092 _ _ w1310 w1635 w1754 w1912 w1988 _ w2059 w2520 w2645 _ w2762 w3003 w3182 _ _ w3360 _]
      tunnel: w75 -> [_ _ _ w218 _ _ _ _ _ _ _ _ w1923 _ _ _ _ _ _ _ _ _ _ _ _ _]
      tunnel: w74 -> [w100 _ w139 w216 w818 w1021 w1104 w1251 _ w1321 w1634 w1753 w1927 _ _ w2027 w2540 _ w2662 w2766 w3006 w3205 _ _ _ _]
      tunnel: w73 -> [_ _ w145 w212 w781 w1031 w1103 w1255 w1289 w1319 w1652 w1761 w1921 w1992 _ w2026 w2531 _ _ w2745 w2902 w3211 _ w3358 w3367 _]
      tunnel: w39 -> [_ _ w141 w223 w815 w1030 w1060 _ _ w1302 _ w1730 _ _ _ w2013 w2483 _ _ _ _ w3155 _ _ _ _]
      tunnel: w69 -> [_ _ _ w222 _ _ _ w1250 _ w1314 w1648 _ _ _ _ _ w2548 _ _ _ _ _ _ w3348 _ _]
      tunnel: w68 -> [_ _ _ w221 _ _ _ _ _ w1336 _ _ _ _ _ _ w2546 _ _ _ _ _ _ _ _ _]
      tunnel: w67 -> [_ _ _ w220 _ _ _ _ _ w1338 _ _ _ _ _ _ w2544 _ _ _ _ _ _ _ _ _]
      tunnel: w66 -> [_ _ _ w219 _ _ _ w1249 _ w1332 w1646 _ _ _ _ _ w2543 _ _ _ _ _ _ w3343 _ _]
      tunnel: w56 -> [_ _ w126 _ _ _ _ _ _ _ _ _ _ _ _ _ _ _ _ _ _ _ w3320 _ _ _]
      tunnel: w55 -> [_ _ w125 _ _ _ _ _ _ _ _ _ _ _ _ _ _ _ _ _ _ _ w3319 _ _ _]
      tunnel: w51 -> [_ _ w120 w211 _ _ _ _ _ w1317 _ _ _ _ _ _ _ _ _ _ _ w3196 _ _ _ _]
      tunnel: w50 -> [_ _ _ _ _ _ _ _ _ w1316 w1630 _ _ _ _ _ _ _ _ _ _ w3198 _ w3345 _ _]
      tunnel: w49 -> [_ _ _ _ _ _ _ _ _ _ _ w1749 _ w1987 _ w2056 _ _ _ _ _ _ _ _ _ _]
      tunnel: w48 -> [_ _ _ _ _ _ _ _ _ _ _ _ _ _ _ _ _ _ _ w2755 w2898 _ _ _ _ _]
      tunnel: w47 -> [_ _ _ _ _ _ _ _ _ _ _ _ _ _ _ w2048 _ _ _ _ _ _ _ _ _ _]
      tunnel: w46 -> [_ _ _ w209 _ _ _ _ _ _ _ _ _ _ _ _ _ _ _ _ _ _ _ _ _ _]
      tunnel: w45 -> [_ _ _ w207 w752 _ w1070 _ _ w1304 _ w1742 _ _ _ w2040 w2496 _ _ _ _ w3167 _ _ _ _]
      tunnel: w44 -> [_ _ _ w208 w754 _ w1071 _ _ w1305 _ w1744 _ _ _ w2042 w2498 _ _ _ _ w3170 _ _ _ _]
      tunnel: w40 -> [_ _ _ w204 _ _ _ _ _ _ _ _ _ _ _ _ _ _ _ _ _ _ _ _ _ _]
      tunnel: w39 -> [_ _ _ w203 _ _ _ _ _ _ _ _ _ _ _ _ _ _ _ _ _ _ _ _ _ _]
      tunnel: w38 -> [_ _ _ w202 _ _ _ _ _ _ _ _ _ _ _ _ _ _ _ _ _ _ _ _ _ _]
      tunnel: w37 -> [_ _ _ w201 _ _ _ _ _ _ _ _ _ _ _ _ _ _ _ _ _ _ _ _ _ _]
      tunnel: w32 -> [_ _ _ _ _ _ _ _ _ _ _ _ _ _ _ _ _ _ _ _ w2903 _ _ _ _ _]
      frame "Initializing...", Default {
        n27 = Unbundle By Name(w100) -> ("misc common.initialized"=w99:refnum<vi>)
        n28 = property class="Bool (strict)"(reference=w99) -> ("Value"=w98:bool)  [unwired: 1 in, 2 out]
        n29 = case shown="True" w98 {
          tunnel: [user_message_v6."Setting defaults..." ("Message to user") user_message_v6."Setting defaults..." ("Message to user")] -> w103
          frame False {
          }
          frame True {
          }
        }
        n30 = Wait (ms)(milliseconds to wait=u32 100) -> ()  [unwired: 1 out]
      }
      frame "Setting defaults..." {
        # "this does not do anything for proportionair"
        # "make new data log folder"
        n31 = call "resetPressures_topLvl.vi"("error in"=w111, "Pressure box control in"=w112) -> ("error out"=w110:errorcluster)  [unwired: 8 in, 1 out]
        n32 = call "reset manipulator.vi"("error in"=w113, "motion"=scope_motion."slow_dualPatch", "manip in"=w114) -> ()  [unwired: 7 in, 2 out]
        n33 = call "reset manipulator.vi"("error in"=w108, "motion"=scope_motion."slow_dualPatch", "manip in"=w109) -> ()  [unwired: 7 in, 2 out]
        n34 = Wait (ms)(milliseconds to wait=u32 500) -> ()  [unwired: 1 out]
      }
      frame "Click OK to start patcherBot!" {
        # "stage idle"
        n35 = Unbundle By Name(w139) -> ("cell tracker common.template_window"=w138:refnum<vi>, "misc common.stage idle?"=w133:refnum<vi>, "positioning+hunting common.unpatched cell indices"=w132:refnum<vi>, "positioning+hunting common.current cell locations (px)"=w128:refnum<vi>, "cell tracker common.cell length (px)"=w123:refnum<vi>, "misc common.Select cells based on proximity (multi patch)"=w119:refnum<vi>)
        n36 = Unbundle By Name(w141) -> ("slice image"=w118:T9, "pipette template"=w140:T9)
        n37 = Unbundle By Name(w145) -> ("state UI indiv"=w144:T27, "cleaning indiv.pre-clean"=w136:refnum<vi>, "cell tracker indiv.cell tracking box (px)"=w134:refnum<vi>, "positioning + hunting indiv.current cell"=w127:refnum<vi>, "state UI indiv.cell tracker"=w124:refnum<vi>)
        n38 = Unbundle By Name(w144) -> ("corrective pipette move"=w143:refnum<vi>)
        n39 = property class="DigNum (strict)"(reference=w138) -> ("Value"=w137:dbl)  [unwired: 1 in, 2 out]
        n40 = property class="Bool (strict)"(reference=w143) -> ("Value"=w142:bool)  [unwired: 1 in, 2 out]
        n41 = property class="Bool (strict)"(reference=w136) -> ("Value"=w135:bool)  [unwired: 1 in, 2 out]
        n42 = case shown="True" w126 {
          tunnel: [user_message_v6."Click OK to start patcherBot!" ("Message to user") w151] -> w147
          tunnel: w118 -> [_ w179]
          tunnel: w142 -> [_ w176]
          tunnel: w140 -> [_ w175]
          tunnel: w137 -> [_ _]
          tunnel: w135 -> [_ w174]
          tunnel: w134 -> [_ w172]
          tunnel: w133 -> [_ _]
          tunnel: w132 -> [_ w171]
          tunnel: w131 -> [_ w170]
          tunnel: w130 -> [_ w169]
          tunnel: w129 -> [_ w168]
          tunnel: w128 -> [_ w167]
          tunnel: w127 -> [_ w165]
          tunnel: w125 -> [_ w163]
          tunnel: w124 -> [_ w161]
          tunnel: w123 -> [_ w159]
          tunnel: w122 -> [_ w156]
          tunnel: w121 -> [_ w157]
          tunnel: w120 -> [_ w150]
          tunnel: w119 -> [_ w153]
          frame False {
          }
          frame True {
            (unwired) user_message_v6."DEBUG STATE" ("Message to user")
            # "DEBUG MODE 9-30-17"
            # "reserve here"
            # "slow down stage"
            # "reset \"user OK\""
            # "IF STAGE NOT RESERVED\nRESERVE STAGE\nIF STAGE RESERVED... WAIT"
            # "box always in middle"
            # "remind user to select pipette template"
            n43 = property class="Bool (strict)"(reference=w161) -> ("Value"=w160:bool)  [unwired: 1 in, 2 out]
            n44 = case shown="True" w176 {
              tunnel: [FALSE w198] -> w184
              tunnel: w175 -> [_ w197]
              frame False {
              }
              frame True {
                n45 = call "IMAQ GetImageSize"("Image"=w197) -> ("Y Resolution"=w199:i32)  [unwired: 3 in, 2 out]
                n46 = Equal To 0?(x=w199) -> (x = 0?=w198:bool)
              }
            }
            n47 = property class="Arr (strict)"(reference=w167) -> (error out=w164:errorcluster, "Value"=w166:dbl[][])  [unwired: 1 in, 1 out]
            n48 = property class="DigNum (strict)"(reference=w159) -> ("Value"=w158:i32)  [unwired: 1 in, 2 out]
            n49 = call "pipette template not selected"("Enable"=w184) -> ()  [unwired: 9 in, 2 out]
            n50 = case shown="True" w160 {
              frame False {
              }
              frame True {
                # "if cell tracker on, clear variables"
                n51 = script code="clearvars -except Pipette_seg Pipette_tip pipette_image"() -> ()  [unwired: 1 in, 1 out]
              }
            }
            n52 = call "get_screenCenter.vi"("use demo values?"=FALSE, "image"=w179) -> ("screen center (px)"=w177:i32[])  [unwired: 9 in]
            n53 = call "boundingBoxCoords.vi"("side length (px)"=w158, "center (x,y)"=w177) -> ("bounding rectangle"=w173:i32[])  [unwired: 8 in, 1 out]
            n54 = property class="Bool (strict)"(reference=w153) -> ("Value"=w152:bool)  [unwired: 1 in, 2 out]
            n55 = Select(t=user_message_v6."Cleaning..." ("Message to user"), s=w174, f=user_message_v6."Starting new attempt..." ("Message to user")) -> (s? t:f=w180:T3)
            n56 = property class="Arr (strict)"(reference=w172, "Value"=w173) -> ()  [unwired: 1 in, 2 out]
            n57 = case shown="True" w152 {
              tunnel: w171 -> [_ w195]
              tunnel: w170 -> [_ w194]
              tunnel: w169 -> [_ w193]
              tunnel: w168 -> [_ w192]
              tunnel: w166 -> [_ w191]
              tunnel: w165 -> [_ w190]
              tunnel: [w185 w187] -> w155
              tunnel: w164 -> [w185 w186]
              frame False {
              }
              frame True {
                # "write to current cell"
                n58 = call "get_nextCellIndex.vi"("which manipulator"=w192, "unpatched cell indices ref"=w195, "error in"=w186, "transform cluster"=w193, "positions cluster"=w194, "current cell locations (px)"=w191) -> ("error out"=w189:errorcluster, "next manip cell"=w188:i32)  [unwired: 3 in, 1 out]
                n59 = property class="DigNum (strict)"(reference=w190, error in=w189, "Value"=w188) -> (error out=w187:errorcluster)  [unwired: 1 out]
              }
            }
            n60 = Select(t=user_message_v6."Click OK to start patcherBot!" ("Message to user"), s=w184, f=w180) -> (s? t:f=w151:T3)
            n61 = call "reset manipulator.vi"("error in"=w155, "motion"=scope_motion."slow_dualPatch", "manip in"=w156) -> ("error out"=w154:errorcluster)  [unwired: 7 in, 1 out]
            n62 = call "reset manipulator.vi"("motion"=w150, "manip in"=w157) -> ()  [unwired: 8 in, 2 out]
            n63 = property class="Bool (strict)"(reference=w163, error in=w154, "Value"=FALSE) -> ()  [unwired: 2 out]
          }
        }
        n64 = Wait (ms)(milliseconds to wait=u32 100) -> ()  [unwired: 1 out]
      }
      frame "Starting new attempt..." {
        # "if idle stage -> start new attempt\nelse -> go wait"
        n65 = Unbundle By Name(w216) -> ("misc common.stage idle?"=w215:refnum<vi>)
        n66 = property on="Property Node" class="Bool (strict)"(reference=w215) -> (reference out=w213:refnum<vi>, "Value"=w200:bool)  [unwired: 1 in, 1 out]
        n67 = case shown="True" w200 {
          tunnel: [user_message_v6."Waiting for idle stage..." ("Message to user") w267] -> w232
          tunnel: w231 -> [_ w266]
          tunnel: w230 -> [_ w265]
          tunnel: w229 -> [_ w264]
          tunnel: [errorcluster {"status"=FALSE, "code"=0, "source"=""} ("error out") w263] -> _
          tunnel: w228 -> [_ w262]
          tunnel: w227 -> [_ w261]
          tunnel: w226 -> [_ w260]
          tunnel: w225 -> [_ w259]
          tunnel: w224 -> [_ w258]
          tunnel: w223 -> [_ w257]
          tunnel: w212 -> [_ w256]
          tunnel: w222 -> [_ w255]
          tunnel: w221 -> [_ w254]
          tunnel: w220 -> [_ w253]
          tunnel: w219 -> [_ w252]
          tunnel: w218 -> [_ w251]
          tunnel: w217 -> [_ w250]
          tunnel: w216 -> [_ w247]
          tunnel: w213 -> [_ w246]
          tunnel: w211 -> [_ w245]
          tunnel: w210 -> [_ w244]
          tunnel: w209 -> [_ w243]
          tunnel: w208 -> [_ w242]
          tunnel: w207 -> [_ w241]
          tunnel: w206 -> [_ w240]
          tunnel: w205 -> [_ w239]
          tunnel: w204 -> [_ w238]
          tunnel: w203 -> [_ w237]
          tunnel: w202 -> [_ w236]
          tunnel: w201 -> [_ w235]
          frame False {
          }
          frame True {
            # "reserve stage"
            n68 = property on="Property Node" class="Bool (strict)"(reference=w246, "Value"=FALSE) -> (error out=w248:errorcluster)  [unwired: 1 in, 1 out]
            n69 = flat-sequence {
              tunnel: [w318] -> w267
              tunnel: w266 -> [w365]
              tunnel: w265 -> [w364]
              tunnel: w264 -> [w363]
              tunnel: [w292] -> w263
              tunnel: w262 -> [w304]
              tunnel: w261 -> [w300]
              tunnel: w260 -> [w298]
              tunnel: w259 -> [w281]
              tunnel: w258 -> [w280]
              tunnel: w247 -> [w357]
              tunnel: w257 -> [w296]
              tunnel: w256 -> [w345]
              tunnel: w255 -> [w339]
              tunnel: w254 -> [w338]
              tunnel: w253 -> [w337]
              tunnel: w252 -> [w336]
              tunnel: w251 -> [w330]
              tunnel: w250 -> [w323]
              tunnel: w248 -> [_]
              tunnel: w245 -> [_]
              tunnel: w244 -> [_]
              tunnel: w243 -> [w291]
              tunnel: w242 -> [w295]
              tunnel: w241 -> [w294]
              tunnel: w240 -> [w286]
              tunnel: w239 -> [w285]
              tunnel: w238 -> [w279]
              tunnel: w237 -> [_]
              tunnel: w236 -> [w273]
              tunnel: w235 -> [w272]
              frame #0 {
                w297 = scope_motion."slow_dualPatch" ("motion")
                w335 = dbl[] []
                w333 = FALSE ("tip found")
                # "RESETTING STUFF FOR NEXT TRIAL"
                # "reset to defaults"
                # "stage to cell"
                # "backlash comp"
                # "negative = up!"
                # "make new folder"
                n70 = Unbundle By Name(w345) -> ("positioning + hunting indiv.vertical z dist (vertical rel only)  (px)"=w278:refnum<vi>, "positioning + hunting indiv.hunt pressure (mBar)"=w284:refnum<vi>, "misc indiv.Break-In Counter"=w289:refnum<vi>, "misc indiv.Saving to..."=w320:refnum<vi>, "positioning + hunting indiv.current cell"=w324:refnum<vi>, "misc indiv.pipette offset (mV)"=w340:refnum<vi>, "state UI indiv.corrective stage move"=w355:refnum<vi>, "cell tracker indiv.cell found"=w334:refnum<vi>, "cell tracker indiv.tip found"=w332:refnum<vi>, "gigaseal indiv.GS extended"=w327:refnum<vi>, "misc indiv.Human in Situ"=w288:refnum<vi>)
                n71 = Unbundle By Name(w357) -> ("positioning+hunting common.current cell locations (px)"=w277:refnum<vi>, "positioning+hunting common.current park plane z (px)"=w352:refnum<vi>, "positioning+hunting common.cells (image px)"=w350:refnum<vi>, "misc common.Data log location"=w346:refnum<vi>, "misc common.mclamp cluster"=w328:refnum<vi>, "vision common.cell match score"=w325:refnum<vi>, "vision common.tracking"=w322:refnum<vi>)  [unwired: 1 out]
                n72 = Unbundle By Name(w296) -> ("slice image"=w276:T9, "cell images ref"=w351:refnum<vi>)
                n73 = Unbundle By Name(w298) -> ("Actuator COM"=w301:refnum<visa-resource-name>)
                n74 = Unbundle By Name(w304) -> ("Actuator COM"=w305:refnum<visa-resource-name>)
                n75 = property class="DigNum (strict)"(reference=w330, "Value"=0) -> ()  [unwired: 1 in, 2 out]
                n76 = property class="Arr (strict)"(reference=w339, "Value"=i32[] []) -> ()  [unwired: 1 in, 2 out]
                n77 = property class="Arr (strict)"(reference=w337, "Value"=w335) -> ()  [unwired: 1 in, 2 out]
                n78 = property class="Arr (strict)"(reference=w338, "Value"=w335) -> ()  [unwired: 1 in, 2 out]
                n79 = Wait (ms)(milliseconds to wait=u32 500) -> ()  [unwired: 1 out]
                n80 = property class="Arr (strict)"(reference=w336, "Value"=w335) -> ()  [unwired: 1 in, 2 out]
                n81 = call "sc_adjustMotion.vi"("error in (no error)"=w300, "motion"=scope_motion."slow_dualPatch", "VISA handle"=w301) -> ("error out"=w299:errorcluster)  [unwired: 7 in, 1 out]
                n82 = call "sc_adjustMotion.vi"("error in (no error)"=w299, "motion"=w297, "VISA handle"=w305) -> ("error out"=w303:errorcluster)  [unwired: 7 in, 1 out]
                n83 = property class="DigNum (strict)"(reference=w324) -> ("Value"=w347:i32)  [unwired: 1 in, 2 out]
                n84 = property class="Bool (strict)"(reference=w322, "Value"=FALSE) -> ()  [unwired: 1 in, 2 out]
                n85 = call "reset manipulator.vi"("error in"=w303, "motion"=w297, "manip in"=w304) -> ("error out"=w311:errorcluster, "manip out"=w293:T25)  [unwired: 7 in]
                n86 = property class="Path"(reference=w346) -> ("Value"=w313:path)  [unwired: 1 in, 2 out]
                n87 = property class="Bool (strict)"(reference=w355) -> ("Value"=w354:bool)  [unwired: 1 in, 2 out]
                n88 = property class="Arr (strict)"(reference=w277) -> (reference out=w353:refnum<vi>, "Value"=w356:dbl[][])  [unwired: 1 in, 1 out]
                n89 = call "get_screenCenter.vi"("image"=w276) -> ("screen center (px)"=w359:i32[])  [unwired: 10 in]
                n90 = call "create_save_folder-v02.vi"("which manipulator"=w323, "current cell"=w347, "log path"=w313) -> ("error out"=w309:errorcluster, "Recording"=w314:string, "Date"=w315:string, "dup path"=w312:path)  [unwired: 5 in]
                n91 = property class="Bool (strict)"(reference=w327, "Value"=FALSE) -> ()  [unwired: 1 in, 2 out]
                n92 = Unbundle By Name(w345) -> ("state UI indiv.successful breakin"=w316:refnum<vi>, "gigaseal indiv.GS timeout (s)"=w344:refnum<vi>, "gigaseal indiv.GS timeout (adjusted)"=w343:refnum<vi>)
                n93 = Current VI's Path() -> (path=w274:path)
                n94 = property class="Path"(reference=w320, error in=w309, "Value"=w312) -> (reference out=w308:refnum<vi>, error out=w307:errorcluster)
                n95 = property class="Path"(reference=w308, error in=w307) -> (error out=w306:errorcluster, "Value"=w275:path)  [unwired: 1 out]
                n96 = call "saveLedgerSeeds.vi"("error in (no error)"=w306, "ExperimentDescriptors 2"=w291, "Recording"=w314, "Date"=w315, "dataRoot"=w275) -> ("error out"=w270:errorcluster)  [unwired: 6 in]
                n97 = property class="Arr (strict)"(reference=w272, error in=w270) -> (error out=w269:errorcluster, "Value"=w271:refnum<vi>[])  [unwired: 1 out]
                n98 = Transpose 2D Array(2D array=w356) -> (transposed array=w282:dbl[][])
                n99 = Index Array(array=w282, index (row)=w347) -> (element=w283:dbl[])  [unwired: 1 in]
                n100 = property class="DigNum (strict)"(reference=w344) -> (error out=w341:errorcluster, "Value"=w342:i32)  [unwired: 1 in, 1 out]
                n101 = property class="DigNum (strict)"(reference=w289, "Value"=0) -> ()  [unwired: 1 in, 2 out]
                n102 = call "stageToCam.vi"("center location"=w359, "transform cluster + actuator"=w280, "current positions"=w281, "cam location (px)"=w283) -> ("stage location (steps)"=w361:dbl[])  [unwired: 6 in, 1 out]
                n103 = call "saveExperimentControlArray_v05.vi"("saveFileName"="mainVIsettings.txt", "filepath"=w275, "error in"=w269, "subVI"=w274, "mainVI"=w273, "control array in"=w271) -> ()  [unwired: 4 in, 2 out]
                n104 = property class="Bool (strict)"(reference=w334, "Value"=w333) -> (reference out=w319:refnum<vi>)  [unwired: 1 in, 1 out]
                n105 = property class="Bool (strict)"(reference=w332, "Value"=w333) -> ()  [unwired: 1 in, 2 out]
                n106 = property class="DigNum (strict)"(reference=w343, error in=w341, "Value"=w342) -> ()  [unwired: 2 out]
                n107 = property class="Arr (strict)"(reference=w350) -> (reference out=w348:refnum<vi>, "Value"=w349:dbl[][])  [unwired: 1 in, 1 out]
                n108 = property class="Bool (strict)"(reference=w316, "Value"=FALSE) -> ()  [unwired: 1 in, 2 out]
                n109 = property class="Bool (strict)"(reference=w288) -> ("Value"=w287:bool)  [unwired: 1 in, 2 out]
                n110 = call "moveTo_abs_XYZ.vi"("blocking?"=TRUE, "error in"=w311, "XYZ location (steps)"=w361, "Actuator cluster in"=w298) -> ("error out"=w358:errorcluster, "Actuator cluster out"=w360:T25)  [unwired: 6 in]
                n111 = case shown="False" w287 {
                  tunnel: w365 -> [w415 w566]
                  tunnel: w364 -> [w414 w565]
                  tunnel: w363 -> [w413 w564]
                  tunnel: w360 -> [_ w555]
                  tunnel: w281 -> [_ w551]
                  tunnel: w359 -> [_ w550]
                  tunnel: w358 -> [w410 w547]
                  tunnel: w283 -> [_ w544]
                  tunnel: w354 -> [_ w543]
                  tunnel: w353 -> [_ w542]
                  tunnel: w352 -> [_ w541]
                  tunnel: w351 -> [_ w540]
                  tunnel: w349 -> [_ w539]
                  tunnel: w348 -> [_ w538]
                  tunnel: w347 -> [w375 w537]
                  tunnel: w340 -> [w409 w536]
                  tunnel: w328 -> [w408 w535]
                  tunnel: w325 -> [_ w534]
                  tunnel: w323 -> [w407 w533]
                  tunnel: w319 -> [_ w532]
                  tunnel: [user_message_v6."Human Positioning..." ("Message to user") user_message_v6."Pipette repositioning..." ("Message to user")] -> w318
                  tunnel: w295 -> [w404 w524]
                  tunnel: w275 -> [w403 w523]
                  tunnel: w276 -> [w402 w522]
                  tunnel: w294 -> [w401 w521]
                  tunnel: w293 -> [w382 w509]
                  tunnel: [w387 w500] -> w292
                  tunnel: w280 -> [w372 w495]
                  tunnel: w286 -> [w368 _]
                  tunnel: w285 -> [w367 _]
                  tunnel: w284 -> [w366 _]
                  tunnel: w281 -> [w373 _]
                  tunnel: w279 -> [_ _]
                  tunnel: w278 -> [w374 _]
                  tunnel: w277 -> [w370 _]
                  frame True {
                    w398 = T28 7 items=["Grayscale (U8)", "Grayscale (I16)", "Grayscale (SGL)", "Complex (CSG)", "RGB (U32)", "HSL (U32)", "RGB (U64)", "Grayscale (U16)"] ("Image Type")
                    (unwired) user_message_v6."DEBUG STATE" ("Message to user")
                    # "create image buffer"
                    # "pipette to position above cell"
                    n112 = call "Time Delay7"("error in (no error)"=w410, "Delay Time (s)"=5.0) -> ("error out"=w376:errorcluster)  [unwired: 9 in]
                    n113 = call "IMAQ Create"("Border Size"=0, "Image Name"="temp", "Image Type"=w398, "error in (no error)"=w376) -> ("New Image"=w392:T9, "error out"=w397:errorcluster)  [unwired: 1 in]
                    n114 = while {
                      tunnel: w402 -> [w466]
                      tunnel: w403 -> [w480]
                      tunnel: w404 -> [w459]
                      tunnel: [w458] -> w396
                      tunnel: w397 -> [w465]
                      tunnel: "images/01-atCell.png" ("name or relative path") -> [w477]
                      tunnel: w401 -> [w475]
                      tunnel: [w456] -> w395
                      tunnel: [w455] -> w394
                      tunnel: [w454] -> w393
                      stop <- w476 stop-if-true
                      n115 = property class="Bool (strict)"(reference=w475) -> ("Value"=w474:bool)  [unwired: 1 in, 2 out]
                      n116 = call "IMAQ GetImageSize"("Image"=w466, "error in (no error)"=w465) -> ("Y Resolution"=w470:i32, "X Resolution"=w473:i32, "error out"=w464:errorcluster)  [unwired: 2 in]
                      n117 = call "IMAQ ImageToArray"("error in (no error)"=w464, "Image"=w466) -> ("Image Pixels (U16)"=w454:u16[][], "error out"=w458:errorcluster)  [unwired: 2 in, 3 out]
                      n118 = Add Array Elements(numeric array=w454) -> (sum=w463:u16)
                      n119 = Build Path(base path=w480, name or relative path=w477) -> (appended path=w455:path)
                      n120 = Index Array(array=w459) -> (element #1=w472:i32, element #2=w471:i32)  [unwired: 2 in]
                      n121 = Equal?(x=w470, y=w471) -> (x = y?=w468:bool)
                      n122 = Greater?(x=w463, y=u16 0) -> (0:w460:bool)
                      n123 = Equal?(x=w473, y=w472) -> (x = y?=w469:bool)
                      n124 = And(x=w469, y=w468) -> (x .and. y?=w461:bool)
                      n125 = Wait (ms)(milliseconds to wait=u32 1000) -> ()  [unwired: 1 out]
                      n126 = And(x=w461, y=w460) -> (x .and. y?=w457:bool)
                      n127 = Select(t="Ready", s=w457, f="Before") -> (s? t:f=w456:string)
                      n128 = Or(x=w457, y=w474) -> (x .or. y?=w476:bool)
                    }
                    n129 = case shown="\"Ready\"" w395 {
                      tunnel: w394 -> [_ w450 _]
                      tunnel: [FALSE TRUE FALSE] -> _
                      tunnel: w396 -> [w439 w444 w452]
                      tunnel: [w439 w442 w452] -> w369
                      tunnel: w393 -> [_ w447 _]
                      tunnel: w392 -> [_ w441 _]
                      frame "Before", Default {
                      }
                      frame "Ready" {
                        n130 = call "IMAQ ArrayToImage"("Image Pixels (U16)"=w447, "error in (no error)"=w444, "Image"=w441) -> ("error out"=w448:errorcluster, "Image Out"=w445:T9)  [unwired: 7 in]
                        n131 = call-poly "IMAQ Write File 2"("error in (no error)"=w448, "Image Quality"=u32 1000, "File Path"=w450, "Image"=w445) -> ("error out"=w443:errorcluster)  [unwired: 6 in, 1 out]
                        n132 = call "IMAQ Dispose"("All Images? (No)"=FALSE, "Image"=w445, "error in (no error)"=w443) -> ("error out"=w442:errorcluster)  [unwired: 3 in]
                      }
                      frame "After" {
                      }
                    }
                    n133 = flat-sequence {
                      tunnel: [w437] -> w391
                      tunnel: w375 -> [_]
                      tunnel: w374 -> [w436]
                      tunnel: w373 -> [w429]
                      tunnel: w372 -> [w425]
                      tunnel: [w432] -> w371
                      tunnel: w370 -> [_]
                      tunnel: w369 -> [w422]
                      frame #0 {
                        w433 = 0.0 ("element")
                        n134 = Unbundle By Name(w429) -> ("current stage pos (steps)"=w428:refnum<vi>)
                        n135 = Unbundle By Name(w425) -> ("s"=w424:refnum<vi>)
                        n136 = property class="Arr (strict)"(reference=w428, error in=w422) -> (error out=w426:errorcluster, "Value"=w427:i32[])  [unwired: 1 out]
                        n137 = property class="Clust (strict)"(reference=w424) -> ("Value"=w423:T24)  [unwired: 1 in, 2 out]
                        n138 = Unbundle By Name(w423) -> ()  [unwired: 1 out]
                        n139 = Index Array(array=w427) -> (element #1=w421:i32, element #2=w420:i32, element #3=w419:i32)  [unwired: 3 in]
                        n140 = Divide(x=w419, y=-7.53 ("x")) -> (x/y=w418:dbl)
                        n141 = Build Array(w421, w420, w418) -> (w416:dbl[])
                        n142 = property class="DigNum (strict)"(reference=w436) -> ("Value"=w435:dbl)  [unwired: 1 in, 2 out]
                        n143 = call "Time Delay33"("error in (no error)"=w426, "Delay Time (s)"=0.2) -> ("error out"=w437:errorcluster)  [unwired: 9 in]
                        n144 = Build Array(w433, w433, w435) -> (w434:dbl[])
                        n145 = call "modify_cell_approach.vi"("approach type"=approach_type."vertical rel", "which manipulator"=T5."manipulator 1", "abs or rel park location (z only) (px)"=w434, "transform cluster + actuator"=w425, "current positions"=w429, "cell location (steps, pipette coord system)"=w416) -> ("approach cell location (steps, pipette coord system)"=w432:dbl[])  [unwired: 3 in, 2 out]
                      }
                    }
                    n146 = call "moveTo_abs_XYZ.vi"("blocking?"=TRUE, "error in"=w391, "XYZ location (steps)"=w371, "Actuator cluster in"=w382) -> ("error out"=w411:errorcluster, "Actuator cluster out"=w380:T25)  [unwired: 6 in]
                    n147 = case shown="True" w413 {
                      tunnel: w414 -> [_ w494]
                      tunnel: w415 -> [_ w489]
                      tunnel: [w481 w482] -> w386
                      tunnel: w411 -> [w481 w485]
                      tunnel: w409 -> [_ w493]
                      tunnel: w408 -> [_ w491]
                      tunnel: w407 -> [_ w486]
                      frame False {
                      }
                      frame True {
                        n148 = property class="Clust (strict)"(reference=w491, error in=w485) -> (error out=w484:errorcluster, "Value"=w490:T29)  [unwired: 1 out]
                        n149 = call "select_mclamp_channel.vi"("which manipulator"=w486, "error in (no error)"=w484, "mclamp cluster"=w490, "Multiclamp Handle In"=w489) -> ("error out"=w487:errorcluster, "Multiclamp Handle out"=w488:u32)  [unwired: 5 in, 1 out]
                        n150 = call "mclamp_auto_offset.vi"("error in (no error)"=w487, "Error in"=w494, "Multiclamp Handle Out"=w488) -> ("error out"=w483:errorcluster, "pipette offset (mV)"=w492:dbl)  [unwired: 7 in]
                        n151 = property class="DigNum (strict)"(reference=w493, error in=w483, "Value"=w492) -> (error out=w482:errorcluster)  [unwired: 1 out]
                      }
                    }
                    n152 = property class="DigNum (strict)"(reference=w366) -> ("Value"=w378:dbl)  [unwired: 1 in, 2 out]
                    n153 = call "setPressure_topLvl.vi"("which manipulator"=T5."manipulator 1", "Slide Refnum"=w367, "error in"=w386, "set pressure (mBar)"=w378, "Pressure box control in"=w368) -> ("error out"=w385:errorcluster)  [unwired: 5 in, 1 out]
                    n154 = call "reset manipulator.vi"("error in"=w385, "approach? (T = on)"=FALSE, "motion"=scope_motion."slow", "manip in"=w380) -> ("error out"=w384:errorcluster)  [unwired: 6 in, 1 out]
                    n155 = call <vilib>:"Play Sound File.vi"("error in (no error)"=w384, "path"=path "C:/multiBot/patcherBot/sounds/LOZ-LTTP_Secret.wav") -> ("error out"=w388:errorcluster)  [unwired: 8 in, 1 out]
                    n156 = call "Time Delay4"("error in (no error)"=w388, "Delay Time (s)"=1.0) -> ("error out"=w387:errorcluster)  [unwired: 9 in]
                  }
                  frame False {
                    w506 = T28 7 items=["Grayscale (U8)", "Grayscale (I16)", "Grayscale (SGL)", "Complex (CSG)", "RGB (U32)", "HSL (U32)", "RGB (U64)", "Grayscale (U16)"] ("Image Type")
                    w518 = T28 7 items=["Grayscale (U8)", "Grayscale (I16)", "Grayscale (SGL)", "Complex (CSG)", "RGB (U32)", "HSL (U32)", "RGB (U64)", "Grayscale (U16)"] ("Image Type")
                    w557 = 0.0
                    (unwired) user_message_v6."DEBUG STATE" ("Message to user")
                    # "create image buffer"
                    # "create image buffer"
                    # "pipette to position above cell"
                    # "stage to position above cell"
                    n157 = call "Time Delay42"("error in (no error)"=w547, "Delay Time (s)"=5.0) -> ("error out"=w546:errorcluster)  [unwired: 9 in]
                    n158 = case shown="True" w543 {
                      tunnel: [w653 w702] -> w517
                      tunnel: w551 -> [w672 w705]
                      tunnel: w495 -> [w671 w683]
                      tunnel: w546 -> [w661 w716]
                      tunnel: w555 -> [w670 w715]
                      tunnel: [w669 w714] -> w554
                      tunnel: w537 -> [w664 w697]
                      tunnel: w522 -> [_ w713]
                      tunnel: w550 -> [w668 w678]
                      tunnel: [w663 w696] -> w549
                      tunnel: [w652 w695] -> w548
                      tunnel: w544 -> [_ _]
                      tunnel: w542 -> [w658 w692]
                      tunnel: w541 -> [w651 w690]
                      tunnel: w540 -> [_ w685]
                      tunnel: w539 -> [_ w694]
                      tunnel: w538 -> [_ w693]
                      tunnel: w537 -> [_ w691]
                      tunnel: w532 -> [_ w688]
                      tunnel: w534 -> [_ w687]
                      frame False {
                        # "backlash comp"
                        n159 = property class="Arr (strict)"(reference=w658, error in=w661) -> (reference out=w655:refnum<vi>, error out=w660:errorcluster, "Value"=w659:dbl[][])
                        n160 = Transpose 2D Array(2D array=w659) -> (transposed array=w667:dbl[][])
                        n161 = Index Array(array=w667, index (row)=w664) -> (element=w666:dbl[])  [unwired: 1 in]
                        n162 = Subtract(x=w666, y=dbl[] [0.0, 0.0, 0.0]) -> (x-y=w673:dbl[])
                        n163 = call "stageToCam.vi"("center location"=w668, "transform cluster + actuator"=w671, "current positions"=w672, "cam location (px)"=w673) -> ("stage location (steps)"=w674:dbl[])  [unwired: 6 in, 1 out]
                        n164 = call "moveTo_abs_XYZ.vi"("blocking?"=TRUE, "error in"=w660, "XYZ location (steps)"=w674, "Actuator cluster in"=w670) -> ("error out"=w662:errorcluster, "Actuator cluster out"=w669:T25)  [unwired: 6 in]
                        n165 = call "Time Delay39"("error in (no error)"=w662, "Delay Time (s)"=2.0) -> ("error out"=w657:errorcluster)  [unwired: 9 in]
                        n166 = property class="Arr (strict)"(reference=w655, error in=w657) -> (error out=w654:errorcluster, "Value"=w656:dbl[][])  [unwired: 1 out]
                        n167 = Transpose 2D Array(2D array=w656) -> (transposed array=w665:dbl[][])
                        n168 = Index Array(array=w665, index (row)=w664) -> (element=w663:dbl[])  [unwired: 1 in]
                        n169 = property class="DigNum (strict)"(reference=w651, error in=w654) -> (error out=w653:errorcluster, "Value"=w652:dbl)  [unwired: 1 out]
                      }
                      frame True {
                        # "wait for current cell locations\nto update!"
                        # "update cell location in array to newly found location"
                        n170 = Unbundle By Name(w683) -> ("s"=w704:refnum<vi>)
                        n171 = property class="DigNum (strict)"(reference=w687) -> ("Value"=w686:sgl)  [unwired: 1 in, 2 out]
                        n172 = property class="Arr (strict)"(reference=w685) -> ("Value"=w684:T9[])  [unwired: 1 in, 2 out]
                        n173 = property class="Clust (strict)"(reference=w704) -> ("Value"=w703:T24)  [unwired: 1 in, 2 out]
                        n174 = flat-sequence {
                          tunnel: w699 -> [w728]
                          tunnel: w705 -> [w729]
                          tunnel: [w729] -> w701
                          tunnel: [w728] -> w700
                          tunnel: [w734] -> w706
                          tunnel: [w732] -> w702
                          tunnel: w701 -> [w733]
                          tunnel: w700 -> [w731]
                          frame #0 {
                            n175 = call "Time Delay40"("Delay Time (s)"=3.0) -> ()  [unwired: 10 in, 1 out]
                          }
                          frame #1 {
                            n176 = Unbundle By Name(w733) -> ("current stage pos (steps)"=w735:refnum<vi>)
                            n177 = call <vilib>:"Clear Errors.vi"("error in (no error)"=w731) -> ("error out"=w730:errorcluster)  [unwired: 5 in, 1 out]
                            n178 = property class="Arr (strict)"(reference=w735, error in=w730) -> (error out=w732:errorcluster, "Value"=w734:i32[])  [unwired: 1 out]
                          }
                        }
                        n179 = call "stageFindCell_v5.vi"("stage in"=w715, "slice image"=w713, "cell index"=w697, "transform cluster + actuator"=w683, "cell match score"=w686, "error in"=w716, "cell images"=w684) -> ("stageout"=w714:T25, "cell found"=w689:bool, "error out"=w699:errorcluster)  [unwired: 3 in, 3 out]
                        n180 = Index Array(array=w706) -> (element #1=w712:i32, element #2=w711:i32, element #3=w708:i32)  [unwired: 3 in]
                        n181 = property class="Bool (strict)"(reference=w688, "Value"=w689) -> ()  [unwired: 1 in, 2 out]
                        n182 = call "transformCoords_3d.vi"("transform properties"=w703, "z"=w708, "y"=w711, "x"=w712) -> ("z out"=w707:dbl, "y out"=w709:dbl, "x out"=w710:dbl)  [unwired: 5 in]
                        n183 = Build Array(w710, w709, w707) -> (w680:dbl[])
                        n184 = Build Array (concatenate)(w678, 0) -> (w681:i32[])
                        n185 = Subtract(x=w681, y=w680) -> (x-y=w679:dbl[])
                        n186 = Replace Array Subset(array=w694, new element=w679, index (col)=w697) -> (w698:dbl[][])  [unwired: 1 in]
                        n187 = flat-sequence {
                          tunnel: w698 -> [w718]
                          tunnel: w693 -> [w717]
                          tunnel: [w725] -> w696
                          tunnel: [w720] -> w695
                          tunnel: w692 -> [w724]
                          tunnel: w691 -> [w722]
                          tunnel: w690 -> [w721]
                          frame #0 {
                            n188 = property class="Arr (strict)"(reference=w717, "Value"=w718) -> ()  [unwired: 1 in, 2 out]
                          }
                          frame #1 {
                            n189 = call "Time Delay41"("Delay Time (s)"=3.0) -> ()  [unwired: 10 in, 1 out]
                          }
                          frame #2 {
                            n190 = property class="DigNum (strict)"(reference=w721) -> ("Value"=w720:dbl)  [unwired: 1 in, 2 out]
                            n191 = property class="Arr (strict)"(reference=w724) -> ("Value"=w723:dbl[][])  [unwired: 1 in, 2 out]
                            n192 = Transpose 2D Array(2D array=w723) -> (transposed array=w726:dbl[][])
                            n193 = Index Array(array=w726, index (row)=w722) -> (element=w725:dbl[])  [unwired: 1 in]
                          }
                        }
                      }
                    }
                    n194 = Build Array(w557, w557, w548) -> (w556:dbl[])
                    n195 = call "camToPipette_abs_3d.vi"("which manipulator"=w533, "transform cluster + actuator"=w495, "current positions"=w551, "abs pixel location"=w549) -> ("pipette location (steps)"=w562:dbl[])  [unwired: 7 in]
                    n196 = call "modify_cell_approach.vi"("approach type"=approach_type."vertical abs", "which manipulator"=w533, "abs or rel park location (z only) (px)"=w556, "transform cluster + actuator"=w495, "current positions"=w551, "cell location (steps, pipette coord system)"=w562) -> ("approach cell location (px)"=w553:dbl[], "approach cell location (steps, pipette coord system)"=w561:dbl[])  [unwired: 3 in, 1 out]
                    n197 = call "IMAQ Create"("Border Size"=0, "Image Name"="temp", "Image Type"=w518, "error in (no error)"=w517) -> ("New Image"=w510:T9, "error out"=w516:errorcluster)  [unwired: 1 in]
                    n198 = while {
                      tunnel: w522 -> [w636]
                      tunnel: w523 -> [w650]
                      tunnel: w524 -> [w629]
                      tunnel: [w628] -> w515
                      tunnel: w516 -> [w635]
                      tunnel: "images/01-atCell.png" ("name or relative path") -> [w647]
                      tunnel: w521 -> [w645]
                      tunnel: [w626] -> w513
                      tunnel: [w625] -> w512
                      tunnel: [w624] -> w511
                      stop <- w646 stop-if-true
                      n199 = property class="Bool (strict)"(reference=w645) -> ("Value"=w644:bool)  [unwired: 1 in, 2 out]
                      n200 = call "IMAQ GetImageSize"("Image"=w636, "error in (no error)"=w635) -> ("Y Resolution"=w640:i32, "X Resolution"=w643:i32, "error out"=w634:errorcluster)  [unwired: 2 in]
                      n201 = call "IMAQ ImageToArray"("error in (no error)"=w634, "Image"=w636) -> ("Image Pixels (U16)"=w624:u16[][], "error out"=w628:errorcluster)  [unwired: 2 in, 3 out]
                      n202 = Add Array Elements(numeric array=w624) -> (sum=w633:u16)
                      n203 = Build Path(base path=w650, name or relative path=w647) -> (appended path=w625:path)
                      n204 = Index Array(array=w629) -> (element #1=w642:i32, element #2=w641:i32)  [unwired: 2 in]
                      n205 = Equal?(x=w640, y=w641) -> (x = y?=w638:bool)
                      n206 = Greater?(x=w633, y=u16 0) -> (0:w630:bool)
                      n207 = Equal?(x=w643, y=w642) -> (x = y?=w639:bool)
                      n208 = And(x=w639, y=w638) -> (x .and. y?=w631:bool)
                      n209 = Wait (ms)(milliseconds to wait=u32 1000) -> ()  [unwired: 1 out]
                      n210 = And(x=w631, y=w630) -> (x .and. y?=w627:bool)
                      n211 = Select(t="Ready", s=w627, f="Before") -> (s? t:f=w626:string)
                      n212 = Or(x=w627, y=w644) -> (x .or. y?=w646:bool)
                    }
                    n213 = case shown="\"Ready\"" w513 {
                      tunnel: w512 -> [_ w593 _]
                      tunnel: [FALSE TRUE FALSE] -> _
                      tunnel: w515 -> [w582 w587 w595]
                      tunnel: [w582 w585 w595] -> w514
                      tunnel: w511 -> [_ w590 _]
                      tunnel: w510 -> [_ w584 _]
                      frame "Before", Default {
                      }
                      frame "Ready" {
                        n214 = call "IMAQ ArrayToImage"("Image Pixels (U16)"=w590, "error in (no error)"=w587, "Image"=w584) -> ("error out"=w591:errorcluster, "Image Out"=w588:T9)  [unwired: 7 in]
                        n215 = call-poly "IMAQ Write File 2"("error in (no error)"=w591, "Image Quality"=u32 1000, "File Path"=w593, "Image"=w588) -> ("error out"=w586:errorcluster)  [unwired: 6 in, 1 out]
                        n216 = call "IMAQ Dispose"("All Images? (No)"=FALSE, "Image"=w588, "error in (no error)"=w586) -> ("error out"=w585:errorcluster)  [unwired: 3 in]
                      }
                      frame "After" {
                      }
                    }
                    n217 = call "Time Delay43"("error in (no error)"=w514, "Delay Time (s)"=0.5) -> ("error out"=w528:errorcluster)  [unwired: 9 in]
                    n218 = call "stageToCam.vi"("error in (no error)"=w528, "center location"=w550, "transform cluster + actuator"=w495, "current positions"=w551, "cam location (px)"=w553) -> ("stage location (steps)"=w552:dbl[], "error out"=w527:errorcluster)  [unwired: 5 in]
                    n219 = call "moveTo_abs_XYZ.vi"("blocking?"=TRUE, "error in"=w527, "XYZ location (steps)"=w552, "Actuator cluster in"=w554) -> ("error out"=w497:errorcluster)  [unwired: 6 in, 1 out]
                    n220 = call "IMAQ Create"("Border Size"=0, "Image Name"="temp", "Image Type"=w506, "error in (no error)"=w497) -> ("New Image"=w505:T9, "error out"=w496:errorcluster)  [unwired: 1 in]
                    n221 = while {
                      tunnel: w522 -> [w610]
                      tunnel: w523 -> [w623]
                      tunnel: w524 -> [w603]
                      tunnel: [w602] -> w499
                      tunnel: w496 -> [w609]
                      tunnel: "images/02-aboveCell.png" ("name or relative path") -> [w621]
                      tunnel: w521 -> [w619]
                      tunnel: [w601] -> w504
                      tunnel: [w600] -> w503
                      tunnel: [w597] -> w498
                      stop <- w620 stop-if-true
                      n222 = property class="Bool (strict)"(reference=w619) -> ("Value"=w618:bool)  [unwired: 1 in, 2 out]
                      n223 = call "IMAQ GetImageSize"("Image"=w610, "error in (no error)"=w609) -> ("Y Resolution"=w614:i32, "X Resolution"=w617:i32, "error out"=w608:errorcluster)  [unwired: 2 in]
                      n224 = call "IMAQ ImageToArray"("error in (no error)"=w608, "Image"=w610) -> ("Image Pixels (U16)"=w597:u16[][], "error out"=w602:errorcluster)  [unwired: 2 in, 3 out]
                      n225 = Add Array Elements(numeric array=w597) -> (sum=w607:u16)
                      n226 = Build Path(base path=w623, name or relative path=w621) -> (appended path=w601:path)
                      n227 = Index Array(array=w603) -> (element #1=w616:i32, element #2=w615:i32)  [unwired: 2 in]
                      n228 = Equal?(x=w614, y=w615) -> (x = y?=w612:bool)
                      n229 = Greater?(x=w607, y=u16 0) -> (0:w604:bool)
                      n230 = Equal?(x=w617, y=w616) -> (x = y?=w613:bool)
                      n231 = And(x=w613, y=w612) -> (x .and. y?=w605:bool)
                      n232 = Wait (ms)(milliseconds to wait=u32 1000) -> ()  [unwired: 1 out]
                      n233 = And(x=w605, y=w604) -> (x .and. y?=w599:bool)
                      n234 = Select(t="Ready", s=w599, f="Before") -> (s? t:f=w600:string)
                      n235 = Or(x=w599, y=w618) -> (x .or. y?=w620:bool)
                    }
                    n236 = case shown="\"Ready\"" w503 {
                      tunnel: w504 -> [_ w578 _]
                      tunnel: [FALSE TRUE FALSE] -> _
                      tunnel: w499 -> [w567 w571 w580]
                      tunnel: [w567 w569 w580] -> w502
                      tunnel: w498 -> [_ w575 _]
                      tunnel: w505 -> [_ w574 _]
                      frame "Before", Default {
                      }
                      frame "Ready" {
                        n237 = call "IMAQ ArrayToImage"("Image Pixels (U16)"=w575, "error in (no error)"=w571, "Image"=w574) -> ("error out"=w576:errorcluster, "Image Out"=w572:T9)  [unwired: 7 in]
                        n238 = call-poly "IMAQ Write File 2"("error in (no error)"=w576, "Image Quality"=u32 1000, "File Path"=w578, "Image"=w572) -> ("error out"=w570:errorcluster)  [unwired: 6 in, 1 out]
                        n239 = call "IMAQ Dispose"("All Images? (No)"=FALSE, "Image"=w572, "error in (no error)"=w570) -> ("error out"=w569:errorcluster)  [unwired: 3 in]
                      }
                      frame "After" {
                      }
                    }
                    n240 = call "Time Delay44"("error in (no error)"=w502, "Delay Time (s)"=0.2) -> ("error out"=w501:errorcluster)  [unwired: 9 in]
                    n241 = call "moveTo_abs_XYZ.vi"("blocking?"=TRUE, "error in"=w501, "XYZ location (steps)"=w561, "Actuator cluster in"=w509) -> ("error out"=w559:errorcluster)  [unwired: 6 in, 1 out]
                    n242 = case shown="True" w564 {
                      tunnel: w565 -> [_ w749]
                      tunnel: w566 -> [_ w744]
                      tunnel: [w736 w737] -> w500
                      tunnel: w559 -> [w736 w740]
                      tunnel: w536 -> [_ w748]
                      tunnel: w535 -> [_ w746]
                      tunnel: w533 -> [_ w741]
                      frame False {
                      }
                      frame True {
                        n243 = property class="Clust (strict)"(reference=w746, error in=w740) -> (error out=w739:errorcluster, "Value"=w745:T29)  [unwired: 1 out]
                        n244 = call "select_mclamp_channel.vi"("which manipulator"=w741, "error in (no error)"=w739, "mclamp cluster"=w745, "Multiclamp Handle In"=w744) -> ("error out"=w742:errorcluster, "Multiclamp Handle out"=w743:u32)  [unwired: 5 in, 1 out]
                        n245 = call "mclamp_auto_offset.vi"("error in (no error)"=w742, "Error in"=w749, "Multiclamp Handle Out"=w743) -> ("error out"=w738:errorcluster, "pipette offset (mV)"=w747:dbl)  [unwired: 7 in]
                        n246 = property class="DigNum (strict)"(reference=w748, error in=w738, "Value"=w747) -> (error out=w737:errorcluster)  [unwired: 1 out]
                      }
                    }
                  }
                }
              }
            }
          }
        }
      }
      frame "Pipette repositioning..." {
        w763 = T28 7 items=["Grayscale (U8)", "Grayscale (I16)", "Grayscale (SGL)", "Complex (CSG)", "RGB (U32)", "HSL (U32)", "RGB (U64)", "Grayscale (U16)"] ("Image Type")
        w823 = 0.0
        # "create image buffer"
        # "if vertical rel -> use vertical z dist\notherwise -> use park plane"
        # "add secondary autofocus here?"
        # "adjust manip coord system"
        # "CALCULATE PIPETTE POSITION (PX)\nAFTER MOVEMENT"
        # "CALCULATE PIPETTE POSITION (PX)\nBEFORE MOVEMENT"
        # "pipette to RE-ADJUSTED approach position"
        # "stage to cell"
        # "position pipette at center of screen"
        n247 = Unbundle By Name(w781) -> ("positioning + hunting indiv.vertical z dist (vertical rel only)  (px)"=w797:refnum<vi>, "positioning + hunting indiv.current cell"=w798:refnum<vi>, "state UI indiv.corrective pipette move"=w817:refnum<vi>, "positioning + hunting indiv.initial positioning"=w809:refnum<vi>, "positioning + hunting indiv.distToDescend (steps)"=w808:refnum<vi>, "positioning + hunting indiv.approach above cell (steps)"=w807:refnum<vi>, "cell tracker indiv.tip found"=w790:refnum<vi>, "cell tracker indiv.screen tip location (px)"=w805:refnum<vi>, "vision indiv.manip position"=w803:refnum<vi>, "positioning + hunting indiv.gross descent pressure (mBar)"=w799:refnum<vi>, "state UI indiv.cell tracker"=w787:refnum<vi>)
        n248 = Unbundle By Name(w815) -> ("pipette template"=w776:T9, "found pipette"=w814:T9, "slice image"=w750:T9)
        n249 = Unbundle By Name(w769) -> ("Actuator COM"=w772:refnum<visa-resource-name>)
        n250 = Unbundle By Name(w818) -> ("positioning+hunting common.current cell locations (px)"=w813:refnum<vi>, "positioning+hunting common.current park plane z (px)"=w810:refnum<vi>, "positioning+hunting common.current pipette locations (px)"=w804:refnum<vi>, "vision common.pipette match score"=w801:refnum<vi>)
        n251 = Wait (ms)(milliseconds to wait=u32 500) -> ()  [unwired: 1 out]
        n252 = call "sc_adjustMotion.vi"("error in (no error)"=w771, "motion"=scope_motion."slow_dualPatch", "VISA handle"=w772) -> ("error out"=w770:errorcluster)  [unwired: 7 in, 1 out]
        n253 = call "get_screenCenter.vi"("image"=w750) -> ("screen center (px)"=w826:i32[])  [unwired: 10 in]
        n254 = property class="Bool (strict)"(reference=w817) -> ("Value"=w816:bool)  [unwired: 1 in, 2 out]
        n255 = property on="Property Node" class="Arr (strict)"(reference=w804, error in=w770) -> (reference out=w802:refnum<vi>, error out=w832:errorcluster, "Value"=w831:dbl[][])
        n256 = Index Array(array=w831, index (row)=w784) -> (element=w824:dbl[])  [unwired: 1 in]
        n257 = case shown="True" w816 {
          tunnel: w826 -> [_ w955]
          tunnel: w769 -> [w939 w953]
          tunnel: w832 -> [w940 w952]
          tunnel: [w940 w951] -> w775
          tunnel: [w939 w950] -> _
          tunnel: w785 -> [_ w949]
          tunnel: w784 -> [_ w948]
          tunnel: w750 -> [_ w947]
          tunnel: w776 -> [_ w946]
          tunnel: w814 -> [_ w945]
          tunnel: w805 -> [_ w944]
          tunnel: w803 -> [_ w943]
          tunnel: w801 -> [_ w942]
          tunnel: [FALSE ("tip found?") w941] -> w791
          frame False {
          }
          frame True {
            n258 = for {
              N: 1 -> [_]
              tunnel: w955 -> [w960]
              tunnel: [w979] -> w950
              tunnel: [w980] -> w951
              tunnel: w953 -> [w975]
              tunnel: w952 -> [w974]
              tunnel: w949 -> [w959]
              tunnel: w948 -> [w962]
              tunnel: w947 -> [w973]
              tunnel: w946 -> [w972]
              tunnel: w945 -> [w961]
              tunnel: w944 -> [w957]
              tunnel: w943 -> [w971]
              tunnel: w942 -> [w969]
              tunnel: [w963] -> w941
              i -> [w964]
              n259 = property class="DigNum (strict)"(reference=w969) -> ("Value"=w967:sgl)  [unwired: 1 in, 2 out]
              n260 = property class="Clust (strict)"(reference=w971) -> ("Value"=w970:T30)  [unwired: 1 in, 2 out]
              n261 = call "Time Delay8"("error in (no error)"=w974, "Delay Time (s)"=1.0) -> ("error out"=w977:errorcluster)  [unwired: 9 in]
              n262 = Multiply(x=w964, y=100) -> (x*y=w966:i32)
              n263 = Add(x=w966, y=w967) -> (x+y=w965:sgl)
              n264 = call "find_pipetteTip_v5.vi"("manip position"=w970, "slice view"=w973, "error in"=w977, "pipette match score"=w965, "pipette template"=w972, "pipette in"=w975) -> ("error out"=w981:errorcluster, "tip found?"=w963:bool, "screen tip location (px)"=w956:i32[], "pipette out"=w976:T25, "found"=w958:T9)  [unwired: 1 out]
              n265 = case shown="True" w963 {
                tunnel: w981 -> [w983 w998]
                tunnel: [w983 w997] -> w980
                tunnel: [w982 w996] -> w979
                tunnel: w976 -> [w982 w995]
                tunnel: w962 -> [_ w992]
                tunnel: w961 -> [_ w990]
                tunnel: w956 -> [_ w989]
                tunnel: w960 -> [_ w988]
                tunnel: w959 -> [_ w987]
                tunnel: w958 -> [_ w986]
                tunnel: w957 -> [_ w985]
                tunnel: w956 -> [_ w984]
                frame False {
                }
                frame True {
                  n266 = property class="Arr (strict)"(reference=w985, "Value"=w984) -> ()  [unwired: 1 in, 2 out]
                  n267 = Subtract(x=w988, y=w989) -> (x-y=w993:i32[])
                  n268 = call "camToPipette_rel_3d.vi"("which manipulator"=w992, "transform cluster + actuator"=w987, "rel cam (px)"=w993) -> ("rel pipette (steps)"=w991:dbl[])  [unwired: 8 in]
                  n269 = To Long Integer(number=w991) -> (32bit integer=w999:i32[])
                  n270 = call "moveTo_rel_XY.vi"("blocking?"=TRUE, "error in"=w998, "XYZ location (steps)"=w999, "Actuator cluster in"=w995) -> ("error out"=w997:errorcluster, "Actuator cluster out"=w996:T25)  [unwired: 6 in]
                  n271 = call "IMAQ Copy"("Image Dst"=w990, "Image Src"=w986) -> ()  [unwired: 4 in, 2 out]
                }
              }
            }
          }
        }
        n272 = property class="DigNum (strict)"(reference=w807) -> ("Value"=w806:i32)  [unwired: 1 in, 2 out]
        n273 = property class="Bool (strict)"(reference=w790, "Value"=w791) -> ()  [unwired: 1 in, 2 out]
        n274 = property class="Enum (strict)"(reference=w809) -> ("Value"=w751:T15)  [unwired: 1 in, 2 out]
        n275 = property class="DigNum (strict)"(reference=w799) -> ("Value"=w800:dbl)  [unwired: 1 in, 2 out]
        n276 = call <vilib>:"Clear Errors.vi"("error in (no error)"=w775, "specific error code to clear (0: all)"=0) -> ("error out"=w768:errorcluster)  [unwired: 4 in, 1 out]
        n277 = call "setPressure_topLvl.vi"("which manipulator"=w784, "Slide Refnum"=w834, "error in"=w768, "set pressure (mBar)"=w800, "Pressure box control in"=w835) -> ("error out"=w755:errorcluster)  [unwired: 5 in, 1 out]
        n278 = call "IMAQ Create"("Border Size"=0, "Image Name"="temp", "Image Type"=w763, "error in (no error)"=w755) -> ("New Image"=w757:T9, "error out"=w758:errorcluster)  [unwired: 1 in]
        n279 = while {
          tunnel: w750 -> [w865]
          tunnel: w753 -> [w879]
          tunnel: w754 -> [w858]
          tunnel: [w857] -> w762
          tunnel: w758 -> [w864]
          tunnel: "images/03-beforeDecent.png" ("name or relative path") -> [w876]
          tunnel: w752 -> [w874]
          tunnel: [w856] -> w761
          tunnel: [w855] -> w760
          tunnel: [w853] -> w759
          stop <- w875 stop-if-true
          n280 = property class="Bool (strict)"(reference=w874) -> ("Value"=w873:bool)  [unwired: 1 in, 2 out]
          n281 = call "IMAQ GetImageSize"("Image"=w865, "error in (no error)"=w864) -> ("Y Resolution"=w869:i32, "X Resolution"=w872:i32, "error out"=w863:errorcluster)  [unwired: 2 in]
          n282 = call "IMAQ ImageToArray"("error in (no error)"=w863, "Image"=w865) -> ("Image Pixels (U16)"=w853:u16[][], "error out"=w857:errorcluster)  [unwired: 2 in, 3 out]
          n283 = Add Array Elements(numeric array=w853) -> (sum=w862:u16)
          n284 = Build Path(base path=w879, name or relative path=w876) -> (appended path=w856:path)
          n285 = Index Array(array=w858) -> (element #1=w871:i32, element #2=w870:i32)  [unwired: 2 in]
          n286 = Equal?(x=w869, y=w870) -> (x = y?=w867:bool)
          n287 = Greater?(x=w862, y=u16 0) -> (0:w859:bool)
          n288 = Equal?(x=w872, y=w871) -> (x = y?=w868:bool)
          n289 = And(x=w868, y=w867) -> (x .and. y?=w860:bool)
          n290 = Wait (ms)(milliseconds to wait=u32 1000) -> ()  [unwired: 1 out]
          n291 = And(x=w860, y=w859) -> (x .and. y?=w854:bool)
          n292 = Select(t="Ready", s=w854, f="Before") -> (s? t:f=w855:string)
          n293 = Or(x=w854, y=w873) -> (x .or. y?=w875:bool)
        }
        n294 = property class="Digital (strict)"(reference=w810) -> ("Value"=w793:dbl)  [unwired: 1 in, 2 out]
        n295 = property class="Digital (strict)"(reference=w797) -> ("Value"=w794:dbl)  [unwired: 1 in, 2 out]
        n296 = property class="DigNum (strict)"(reference=w798) -> ("Value"=w811:i32)  [unwired: 1 in, 2 out]
        n297 = property class="Arr (strict)"(reference=w813) -> ("Value"=w812:dbl[][])  [unwired: 1 in, 2 out]
        n298 = case shown="\"Ready\"" w760 {
          tunnel: w761 -> [_ w849 _]
          tunnel: [FALSE TRUE FALSE] -> _
          tunnel: w762 -> [w838 w842 w851]
          tunnel: [w838 w840 w851] -> w756
          tunnel: w759 -> [_ w846 _]
          tunnel: w757 -> [_ w845 _]
          frame "Before", Default {
          }
          frame "Ready" {
            n299 = call "IMAQ ArrayToImage"("Image Pixels (U16)"=w846, "error in (no error)"=w842, "Image"=w845) -> ("error out"=w847:errorcluster, "Image Out"=w843:T9)  [unwired: 7 in]
            n300 = call-poly "IMAQ Write File 2"("error in (no error)"=w847, "Image Quality"=u32 1000, "File Path"=w849, "Image"=w843) -> ("error out"=w841:errorcluster)  [unwired: 6 in, 1 out]
            n301 = call "IMAQ Dispose"("All Images? (No)"=FALSE, "Image"=w843, "error in (no error)"=w841) -> ("error out"=w840:errorcluster)  [unwired: 3 in]
          }
          frame "After" {
          }
        }
        n302 = property on="Property Node" class="Arr (strict)"(reference=w802, error in=w756) -> (error out=w828:errorcluster, "Value"=w830:dbl[][])  [unwired: 1 out]
        n303 = Equal?(x=w751, y=approach_type."vertical rel" ("Value")) -> (x = y?=w795:bool)
        n304 = Select(t=w794, s=w795, f=w793) -> (s? t:f=w792:dbl)
        n305 = Index Array(array=w830, index (row)=w784) -> (element=w825:dbl[])  [unwired: 1 in]
        n306 = Subtract(x=w825, y=w824) -> (x-y=w829:dbl[])
        n307 = Transpose 2D Array(2D array=w812) -> (transposed array=w821:dbl[][])
        n308 = Build Array(w823, w823, w792) -> (w822:dbl[])
        n309 = Index Array(array=w821, index (row)=w811) -> (element=w820:dbl[])  [unwired: 1 in]
        n310 = call "adjust_manip_coordSystem.vi"("which manipulator"=w784, "error in"=w828, "transform cluster + actuator"=w785, "pipette position difference (px)"=w829) -> ("error out"=w819:errorcluster)  [unwired: 7 in]
        n311 = flat-sequence {
          tunnel: w833 -> [w918]
          tunnel: w769 -> [w931]
          tunnel: w751 -> [w930]
          tunnel: w827 -> [w914]
          tunnel: w819 -> [w908]
          tunnel: w826 -> [w919]
          tunnel: [w923] -> _
          tunnel: [w927] -> _
          tunnel: w785 -> [w915]
          tunnel: w822 -> [w926]
          tunnel: w784 -> [w925]
          tunnel: w820 -> [w920]
          tunnel: w806 -> [w924]
          tunnel: w808 -> [w917]
          tunnel: [w915] -> w789
          tunnel: [w915] -> w783
          tunnel: [w914] -> w782
          tunnel: [w910] -> w778
          frame #0 {
            # "stage to cell position"
            # "pipette to top of slice position"
            n312 = call "camToPipette_abs_3d.vi"("which manipulator"=w925, "transform cluster + actuator"=w915, "current positions"=w914, "abs pixel location"=w920) -> ("pipette location (steps)"=w929:dbl[])  [unwired: 7 in]
            n313 = call "modify_cell_approach.vi"("approach above cell (steps)"=w924, "approach type"=w930, "which manipulator"=w925, "abs or rel park location (z only) (px)"=w926, "transform cluster + actuator"=w915, "current positions"=w914, "cell location (steps, pipette coord system)"=w929) -> ("distToDescend (steps)"=w913:i32, "approach cell location (steps, pipette coord system)"=w916:dbl[])  [unwired: 2 in, 1 out]
            n314 = disable-structure shown="Enabled" {
              disable-tunnel: w913 -> [w935 w937]
              disable-tunnel: [w932 w937] -> w912
              frame Disabled {
                n315 = Divide(x=w935, y=75.3) -> (x/y=w934:dbl)
                n316 = Round To Nearest(number=w934) -> (nearest integer value=w933:dbl)
                n317 = To Long Integer(number=w933) -> (32bit integer=w932:i32)
              }
              frame Enabled {
              }
            }
            n318 = call "Time Delay28"("error in (no error)"=w908, "Delay Time (s)"=1.0) -> ("error out"=w907:errorcluster)  [unwired: 9 in]
            n319 = call "stageToCam.vi"("center location"=w919, "transform cluster + actuator"=w915, "current positions"=w914, "cam location (px)"=w920) -> ("stage location (steps)"=w921:dbl[])  [unwired: 6 in, 1 out]
            n320 = property class="DigNum (strict)"(reference=w917, "Value"=w912) -> ()  [unwired: 1 in, 2 out]
            n321 = call "moveTo_abs_XYZ.vi"("blocking?"=TRUE, "error in"=w907, "XYZ location (steps)"=w921, "Actuator cluster in"=w918) -> ("error out"=w911:errorcluster, "Actuator cluster out"=w923:T25)  [unwired: 6 in]
            n322 = call "moveTo_abs_XYZ.vi"("blocking?"=TRUE, "error in"=w911, "XYZ location (steps)"=w916, "Actuator cluster in"=w931) -> ("error out"=w910:errorcluster, "Actuator cluster out"=w927:T25)  [unwired: 6 in]
          }
        }
        n323 = Unbundle By Name(w781) -> ("vision indiv.cell tracker XY zero adjustment (px)"=w779:refnum<vi>, "vision indiv.no cell tracker XY zero adjustment (px)"=w780:refnum<vi>)
        n324 = case shown="\"manipulator 1\", Default" w784 {
          tunnel: w789 -> [w900 w902 w904 w906]
          tunnel: [w899 w901 w903 w905] -> w788
          frame "manipulator 1", Default {
            n325 = Unbundle By Name(w900) -> ("manip 1"=w899:refnum<vi>)
          }
          frame "manipulator 2" {
            n326 = Unbundle By Name(w902) -> ("manip 2"=w901:refnum<vi>)
          }
          frame "manipulator 3" {
            n327 = Unbundle By Name(w904) -> ("manip 3"=w903:refnum<vi>)
          }
          frame "manipulator 4" {
            n328 = Unbundle By Name(w906) -> ("manip 4"=w905:refnum<vi>)
          }
        }
        n329 = property class="Bool (strict)"(reference=w787) -> ("Value"=w786:bool)  [unwired: 1 in, 2 out]
        n330 = case shown="False" w786 {
          tunnel: w788 -> [_ w898]
          tunnel: w784 -> [w888 _]
          tunnel: w783 -> [w885 _]
          tunnel: w782 -> [w886 _]
          tunnel: w780 -> [w884 _]
          tunnel: w779 -> [_ w892]
          tunnel: w778 -> [w882 w890]
          tunnel: [w881 w890] -> w777
          frame False {
            # "fudge factor for when not using cell tracker"
            n331 = property class="Arr (strict)"(reference=w884) -> ("Value"=w883:dbl[])  [unwired: 1 in, 2 out]
            n332 = Wait (ms)(milliseconds to wait=u32 500) -> ()  [unwired: 1 out]
            n333 = call "camToPipette_rel_3d.vi"("which manipulator"=w888, "transform cluster + actuator"=w885, "rel cam (px)"=w883) -> ("rel pipette (steps)"=w889:dbl[])  [unwired: 8 in]
            n334 = call "move manipulator rel.vi"("blocking?"=TRUE, "which manipulator"=w888, "error in (no error)"=w882, "transform cluster + actuator"=w885, "positions"=w886, "location (steps)"=w889) -> ("error out"=w881:errorcluster)  [unwired: 5 in]
          }
          frame True {
            # "fudge factor for cell tracker"
            n335 = property class="Clust (strict)"(reference=w898) -> (reference out=w893:refnum<vi>, "Value"=w897:T24)  [unwired: 1 in, 1 out]
            n336 = property class="Arr (strict)"(reference=w892) -> ("Value"=w891:dbl[])  [unwired: 1 in, 2 out]
            n337 = Unbundle By Name(w897) -> ("zero loc (x,y,z)"=w895:dbl[])
            n338 = Add(x=w895, y=w891) -> (x+y=w896:dbl[])
            n339 = Bundle By Name(cluster=w897, "zero loc (x,y,z)"=w896) -> (w894:T24)
            n340 = property class="Clust (strict)"(reference=w893, "Value"=w894) -> ()  [unwired: 1 in, 2 out]
          }
        }
      }
      frame "Initializing cell tracker..." {
        n341 = Unbundle By Name(w1021) -> ("cell tracker common"=w1020:T31)
        n342 = Unbundle By Name(w1021) -> ("vision common"=w1026:T32)
        n343 = Unbundle By Name(w1030) -> ("slice image"=w1000:T9, "pipette mask for cell tracker"=w1029:T9)
        n344 = Unbundle By Name(w1031) -> ("state UI indiv.cell tracker"=w1028:refnum<vi>, "cell tracker indiv.cell tracking box (px)"=w1004:refnum<vi>)
        n345 = Unbundle By Name(w1020) -> ("solver_beta"=w1019:refnum<vi>, "solver_kappa"=w1018:refnum<vi>, "shear_angle"=w1017:refnum<vi>, "solver_gamma"=w1016:refnum<vi>, "template_window"=w1015:refnum<vi>, "debug_mode"=w1014:refnum<vi>, "psf_sigma"=w1013:refnum<vi>, "solver_name"=w1012:refnum<vi>, "pipette template threshold"=w1003:refnum<vi>)
        n346 = Unbundle By Name(w1026) -> ("init tracker success"=w1025:refnum<vi>, "exit tracker success"=w1024:refnum<vi>, "tracking"=w1023:refnum<vi>, "init error out"=w1022:refnum<vi>)  [unwired: 1 out]
        n347 = property class="Bool (strict)"(reference=w1028) -> ("Value"=w1027:bool)  [unwired: 1 in, 2 out]
        n348 = property class="DigNum (strict)"(reference=w1013) -> ("Value"=w1010:dbl)  [unwired: 1 in, 2 out]
        n349 = property class="DigNum (strict)"(reference=w1003) -> ("Value"=w1002:dbl)  [unwired: 1 in, 2 out]
        n350 = property class="DigNum (strict)"(reference=w1015) -> ("Value"=w1011:dbl)  [unwired: 1 in, 2 out]
        n351 = property class="DigNum (strict)"(reference=w1016) -> ("Value"=w1008:dbl)  [unwired: 1 in, 2 out]
        n352 = property class="DigNum (strict)"(reference=w1017) -> ("Value"=w1001:dbl)  [unwired: 1 in, 2 out]
        n353 = property class="DigNum (strict)"(reference=w1018) -> ("Value"=w1007:dbl)  [unwired: 1 in, 2 out]
        n354 = property class="Bool (strict)"(reference=w1014) -> ("Value"=w1006:bool)  [unwired: 1 in, 2 out]
        n355 = property class="DigNum (strict)"(reference=w1019) -> ("Value"=w1009:dbl)  [unwired: 1 in, 2 out]
        n356 = property class="Str"(reference=w1012) -> ("Value"=w1005:string)  [unwired: 1 in, 2 out]
        n357 = case shown="True" w1027 {
          tunnel: w1029 -> [_ _]
          tunnel: w1000 -> [_ w1051]
          tunnel: w1024 -> [_ w1050]
          tunnel: w1025 -> [_ w1047]
          tunnel: w1023 -> [_ w1046]
          tunnel: w1022 -> [_ w1045]
          tunnel: w1011 -> [_ w1043]
          tunnel: w1001 -> [_ w1042]
          tunnel: w1010 -> [_ w1041]
          tunnel: w1009 -> [_ w1040]
          tunnel: w1008 -> [_ w1039]
          tunnel: w1007 -> [_ w1038]
          tunnel: w1006 -> [_ w1037]
          tunnel: w1005 -> [_ w1036]
          tunnel: w1004 -> [_ w1034]
          tunnel: w1002 -> [_ w1033]
          frame False {
          }
          frame True {
            n358 = property class="Bool (strict)"(reference=w1050, "Value"=FALSE) -> ()  [unwired: 1 in, 2 out]
            n359 = call "IMAQ ImageToArray"("Image"=w1051) -> ("Image Pixels (U8)"=w1056:u8[][])  [unwired: 3 in, 4 out]
            n360 = Build Array(w1043, w1042, w1041, w1040, w1039, w1038, w1033) -> (w1055:dbl[])
            n361 = property class="Arr (strict)"(reference=w1034) -> ("Value"=w1035:i32[])  [unwired: 1 in, 2 out]
            n362 = Add(x=w1055, y=0.0) -> (x+y=w1053:dbl[])
            n363 = Boolean To (0,1)(Boolean=w1037) -> (0, 1=w1052:i16)
            n364 = script code="% initialize tracking code\n\ntemplate_window = solver_params(1);\nshear_angle = solver_params(2);\npsf_sigma = solver_params(3);\nsolver_beta = solver_params(4);\nsolver_gamma = solver_params(5);\nsolver_kappa = solver_params(6);\npipette_template_threshold = solver_params(7);\n\ninit_cellTracker_flag = 0;\ninit_cellTracker;"("template_loc"=w1035, "LV_image"=w1056, "solver_params"=w1053, "solver_name"=w1036, "DEBUG_MODE"=w1052) -> ("??"=w1044:errorcluster, "init_cellTracker_flag"=w1058:dbl)  [unwired: 1 in]
            n365 = Not Equal To 0?(x=w1058) -> (x != 0?=w1048:bool)
            n366 = property on="Property Node" class="Bool (strict)"(reference=w1046, error in=w1044, "Value"=TRUE ("tracking")) -> ()  [unwired: 2 out]
            n367 = property class="Clust (strict)"(reference=w1045, "Value"=w1044) -> ()  [unwired: 1 in, 2 out]
            n368 = property class="Bool (strict)"(reference=w1047, "Value"=w1048) -> ()  [unwired: 1 in, 2 out]
          }
        }
      }
      frame "Gross approach..." {
        # "human positioning"
        # "picture before pipette descent"
        # "move pipette to above cell"
        # "set neuron hunt step"
        # "scaling factor conversions"
        # "set pipette speed to slow\napproach on"
        # "move stage to cell"
        n369 = Unbundle By Name(w1104) -> ("positioning+hunting common.current cell locations (px)"=w1101:refnum<vi>, "misc common.stage idle?"=w1088:refnum<vi>)
        n370 = Unbundle By Name(w1103) -> ("positioning + hunting indiv.current cell"=w1085:refnum<vi>, "positioning + hunting indiv.initial positioning"=w1102:refnum<vi>, "positioning + hunting indiv.distToDescend (steps)"=w1098:refnum<vi>, "positioning + hunting indiv.NH step size (steps)"=w1096:refnum<vi>, "positioning + hunting indiv.d(above cell) (steps)"=w1094:refnum<vi>, "misc indiv.stage reservation options"=w1091:refnum<vi>, "positioning + hunting indiv.hunt pressure (mBar)"=w1087:refnum<vi>, "misc indiv.Human in Situ"=w1067:refnum<vi>)
        n371 = Wait (ms)(milliseconds to wait=u32 500) -> ()  [unwired: 1 out]
        n372 = Unbundle By Name(w1060) -> ("slice image"=w1059:T9)
        n373 = disable-structure shown="Enabled" {
          disable-tunnel: w1072 -> [w1134 _]
          disable-tunnel: w1071 -> [w1133 _]
          disable-tunnel: w1059 -> [w1132 _]
          disable-tunnel: w1070 -> [w1131 _]
          disable-tunnel: [w1126 w1178] -> w1069
          disable-tunnel: w1068 -> [w1122 w1178]
          frame Disabled {
            w1128 = T28 7 items=["Grayscale (U8)", "Grayscale (I16)", "Grayscale (SGL)", "Complex (CSG)", "RGB (U32)", "HSL (U32)", "RGB (U64)", "Grayscale (U16)"] ("Image Type")
            # "create image buffer"
            n374 = call "IMAQ Create"("Border Size"=0, "Image Name"="temp", "Image Type"=w1128, "error in (no error)"=w1122) -> ("New Image"=w1120:T9, "error out"=w1121:errorcluster)  [unwired: 1 in]
            n375 = while {
              tunnel: w1132 -> [w1163]
              tunnel: w1134 -> [w1177]
              tunnel: w1133 -> [w1156]
              tunnel: [w1155] -> w1127
              tunnel: w1121 -> [w1162]
              tunnel: "images/03-beforeDecent.png" ("name or relative path") -> [w1174]
              tunnel: w1131 -> [w1172]
              tunnel: [w1154] -> w1125
              tunnel: [w1153] -> w1124
              tunnel: [w1151] -> w1123
              stop <- w1173 stop-if-true
              n376 = property class="Bool (strict)"(reference=w1172) -> ("Value"=w1171:bool)  [unwired: 1 in, 2 out]
              n377 = call "IMAQ GetImageSize"("Image"=w1163, "error in (no error)"=w1162) -> ("Y Resolution"=w1167:i32, "X Resolution"=w1170:i32, "error out"=w1161:errorcluster)  [unwired: 2 in]
              n378 = call "IMAQ ImageToArray"("error in (no error)"=w1161, "Image"=w1163) -> ("Image Pixels (U16)"=w1151:u16[][], "error out"=w1155:errorcluster)  [unwired: 2 in, 3 out]
              n379 = Add Array Elements(numeric array=w1151) -> (sum=w1160:u16)
              n380 = Build Path(base path=w1177, name or relative path=w1174) -> (appended path=w1154:path)
              n381 = Index Array(array=w1156) -> (element #1=w1169:i32, element #2=w1168:i32)  [unwired: 2 in]
              n382 = Equal?(x=w1167, y=w1168) -> (x = y?=w1165:bool)
              n383 = Greater?(x=w1160, y=u16 0) -> (0:w1157:bool)
              n384 = Equal?(x=w1170, y=w1169) -> (x = y?=w1166:bool)
              n385 = And(x=w1166, y=w1165) -> (x .and. y?=w1158:bool)
              n386 = Wait (ms)(milliseconds to wait=u32 1000) -> ()  [unwired: 1 out]
              n387 = And(x=w1158, y=w1157) -> (x .and. y?=w1152:bool)
              n388 = Select(t="Ready", s=w1152, f="Before") -> (s? t:f=w1153:string)
              n389 = Or(x=w1152, y=w1171) -> (x .or. y?=w1173:bool)
            }
            n390 = case shown="\"Ready\"" w1124 {
              tunnel: w1125 -> [_ w1147 _]
              tunnel: [FALSE TRUE FALSE] -> _
              tunnel: w1127 -> [w1136 w1140 w1149]
              tunnel: [w1136 w1138 w1149] -> w1126
              tunnel: w1123 -> [_ w1144 _]
              tunnel: w1120 -> [_ w1143 _]
              frame "Before", Default {
              }
              frame "Ready" {
                n391 = call "IMAQ ArrayToImage"("Image Pixels (U16)"=w1144, "error in (no error)"=w1140, "Image"=w1143) -> ("error out"=w1145:errorcluster, "Image Out"=w1141:T9)  [unwired: 7 in]
                n392 = call-poly "IMAQ Write File 2"("error in (no error)"=w1145, "Image Quality"=u32 1000, "File Path"=w1147, "Image"=w1141) -> ("error out"=w1139:errorcluster)  [unwired: 6 in, 1 out]
                n393 = call "IMAQ Dispose"("All Images? (No)"=FALSE, "Image"=w1141, "error in (no error)"=w1139) -> ("error out"=w1138:errorcluster)  [unwired: 3 in]
              }
              frame "After" {
              }
            }
          }
          frame Enabled {
          }
        }
        n394 = call "Time Delay31"("error in (no error)"=w1069, "Delay Time (s)"=1.0) -> ("error out"=w1074:errorcluster)  [unwired: 9 in]
        n395 = property class="DigNum (strict)"(reference=w1087) -> ("Value"=w1086:dbl)  [unwired: 1 in, 2 out]
        n396 = property class="DigNum (strict)"(reference=w1098) -> ("Value"=w1097:i32)  [unwired: 1 in, 2 out]
        n397 = property class="DigNum (strict)"(reference=w1085) -> ("Value"=w1099:i32)  [unwired: 1 in, 2 out]
        n398 = property class="Enum (strict)"(reference=w1102) -> ("Value"=w1078:T15)  [unwired: 1 in, 2 out]
        n399 = property class="Arr (strict)"(reference=w1101) -> ("Value"=w1100:dbl[][])  [unwired: 1 in, 2 out]
        n400 = property class="DigNum (strict)"(reference=w1094) -> ("Value"=w1093:i32)  [unwired: 1 in, 2 out]
        n401 = Transpose 2D Array(2D array=w1100) -> (transposed array=w1106:dbl[][])
        n402 = Index Array(array=w1106, index (row)=w1099) -> (element=w1105:dbl[])  [unwired: 1 in]
        n403 = case shown="\"vertical abs\", Default" w1078 {
          tunnel: w1093 -> [w1193 w1203 w1215 _ w1235]
          tunnel: w1117 -> [w1190 _ w1217 _ _]
          tunnel: w1114 -> [w1195 _ w1216 _ _]
          tunnel: w1105 -> [_ _ _ _ _]
          tunnel: w1074 -> [_ w1207 w1211 w1232 w1236]
          tunnel: [w1191 w1206 w1218 w1232 w1238] -> w1116
          tunnel: [w1189 w1205 w1212 w1231 w1239] -> w1083
          tunnel: w1092 -> [w1192 _ w1214 _ _]
          tunnel: w1097 -> [w1194 w1199 w1213 _ w1234]
          tunnel: w1113 -> [w1189 w1201 w1212 w1231 w1237]
          frame "vertical abs", Default {
            w1198 = 0
            # "move to relative distance above cell"
            n404 = Subtract(x=w1194, y=w1193) -> (x-y=w1188:i32)
            n405 = Build Array(w1198, w1198, w1188) -> (w1197:i32[])
            n406 = call "move manipulator rel.vi"("blocking?"=TRUE, "which manipulator"=w1192, "transform cluster + actuator"=w1195, "positions"=w1190, "location (steps)"=w1197) -> ("error out"=w1191:errorcluster)  [unwired: 6 in]
          }
          frame "approach" {
            # "pipette to x um away from cell"
            n407 = Subtract(x=w1199, y=w1203) -> (x-y=w1202:i32)
            n408 = call "set step.vi"("error in"=w1207, "step distance (steps)"=w1202, "actuator in"=w1201) -> ("error out"=w1209:errorcluster, "actuator out"=w1208:T25)  [unwired: 7 in]
            n409 = call "take step.vi"("approach?"=TRUE, "motion"=scope_motion."slow" ("gross approach speed"), "blocking?"=TRUE, "error in"=w1209, "actuator in"=w1208) -> ("error out"=w1206:errorcluster, "actuator out"=w1205:T25)  [unwired: 5 in]
          }
          frame "vertical rel" {
            # "should not need to go anywhere.  \npipette should be ready to start hunting already"
            n410 = disable-structure shown="Disabled" {
              disable-tunnel: [w1225 w1230] -> w1218
              disable-tunnel: w1217 -> [w1224 _]
              disable-tunnel: w1216 -> [w1223 _]
              disable-tunnel: w1215 -> [w1222 _]
              disable-tunnel: w1214 -> [w1221 _]
              disable-tunnel: w1213 -> [w1220 _]
              disable-tunnel: w1211 -> [w1219 w1230]
              frame Disabled {
                w1228 = 0
                n411 = Subtract(x=w1220, y=w1222) -> (x-y=w1229:i32)
                n412 = Build Array(w1228, w1228, w1229) -> (w1227:i32[])
                n413 = call "move manipulator rel.vi"("blocking?"=TRUE, "which manipulator"=w1221, "error in (no error)"=w1219, "transform cluster + actuator"=w1223, "positions"=w1224, "location (steps)"=w1227) -> ("error out"=w1225:errorcluster)  [unwired: 5 in]
              }
              frame Enabled {
              }
            }
          }
          frame "right to cell" {
          }
          frame "approach above" {
            n414 = Subtract(x=w1234, y=w1235) -> (x-y=w1233:i32)
            n415 = call "set step.vi"("error in"=w1236, "step distance (steps)"=w1233, "actuator in"=w1237) -> ("error out"=w1243:errorcluster, "actuator out"=w1242:T25)  [unwired: 7 in]
            n416 = call "take step.vi"("approach?"=TRUE, "motion"=scope_motion."slow" ("gross approach speed"), "blocking?"=TRUE, "error in"=w1243, "actuator in"=w1242) -> ("error out"=w1238:errorcluster, "actuator out"=w1239:T25)  [unwired: 5 in]
          }
        }
        n417 = property class="DigNum (strict)"(reference=w1096) -> ("Value"=w1095:i32)  [unwired: 1 in, 2 out]
        n418 = call "Time Delay11"("error in (no error)"=w1116, "Delay Time (s)"=1.0) -> ("error out"=w1110:errorcluster)  [unwired: 9 in]
        n419 = call "setPressure_topLvl.vi"("which manipulator"=w1092, "Slide Refnum"=w1109, "error in"=w1110, "set pressure (mBar)"=w1086, "Pressure box control in"=w1111) -> ("error out"=w1107:errorcluster)  [unwired: 5 in, 1 out]
        n420 = Equal?(x=w1078, y=approach_type."approach" ("initial positioning type")) -> (x = y?=w1077:bool)
        n421 = call "Time Delay12"("error in (no error)"=w1107, "Delay Time (s)"=1.0) -> ("error out"=w1081:errorcluster)  [unwired: 9 in]
        n422 = call "reset manipulator.vi"("error in"=w1081, "approach? (T = on)"=w1077, "motion"=scope_motion."slow", "manip in"=w1083) -> ("error out"=w1080:errorcluster, "manip out"=w1082:T25)  [unwired: 6 in]
        n423 = disable-structure shown="Disabled" {
          disable-tunnel: w1059 -> [w1184 _]
          disable-tunnel: [w1183 w1185] -> w1084
          disable-tunnel: w1072 -> [w1181 _]
          disable-tunnel: w1080 -> [w1179 w1185]
          frame Disabled {
            # "picture after pipette descent"
            n424 = Build Path(base path=w1181, name or relative path="after.tiff") -> (appended path=w1180:path)
            n425 = call-poly "IMAQ Write File 2"("error in (no error)"=w1179, "File Path"=w1180, "Image"=w1184) -> ("error out"=w1183:errorcluster)  [unwired: 7 in, 1 out]
          }
          frame Enabled {
          }
        }
        n426 = call "set step.vi"("error in"=w1084, "step distance (steps)"=w1095, "actuator in"=w1082) -> ("error out"=w1090:errorcluster)  [unwired: 7 in, 1 out]
        n427 = property class="Enum (strict)"(reference=w1091, error in=w1090) -> (error out=w1065:errorcluster, "Value"=w1089:T33)  [unwired: 1 out]
        n428 = case shown="\"unreserve after gross approach\", Default" w1089 {
          tunnel: w1088 -> [w1187 _]
          frame "unreserve after gross approach", Default {
            n429 = property class="Bool (strict)"(reference=w1187, "Value"=TRUE) -> ()  [unwired: 1 in, 2 out]
          }
          frame "unreserve after cell found" {
          }
        }
        n430 = property class="Bool (strict)"(reference=w1067) -> ("Value"=w1066:bool)  [unwired: 1 in, 2 out]
        n431 = case shown="False" w1066 {
          tunnel: [user_message_v6."Detecting cell..." ("Message to user") user_message_v6."Human Positioning..." ("Message to user")] -> w1112
          frame False {
          }
          frame True {
          }
        }
        n432 = call <vilib>:"Play Sound File.vi"("error in (no error)"=w1065, "path"=path "C:/multiBot/patcherBot/sounds/LOZ-LTTP_Secret.wav") -> ("error out"=w1062:errorcluster)  [unwired: 8 in, 1 out]
        n433 = call "Time Delay36"("error in (no error)"=w1062, "Delay Time (s)"=1.0) -> ("error out"=w1061:errorcluster)  [unwired: 9 in]
      }
      frame "Human Positioning..." {
        n434 = Unbundle By Name(w1255) -> ("misc indiv.stage reservation options"=w1246:refnum<vi>, "gigaseal indiv.start GS time"=w1248:refnum<vi>, "misc indiv.Human Control Done"=w1254:refnum<vi>, "misc indiv.State to advance to after Human Control"=w1253:refnum<vi>)
        n435 = Unbundle By Name(w1251) -> ("misc common.stage idle?"=w1245:refnum<vi>)  [unwired: 1 out]
        n436 = flat-sequence {
          tunnel: [w1258] -> w1252
          tunnel: w1254 -> [w1257]
          tunnel: [w1267] -> w1256
          tunnel: w1252 -> [_]
          tunnel: w1253 -> [w1274]
          tunnel: w1245 -> [w1272]
          tunnel: w1250 -> [w1269]
          tunnel: w1249 -> [w1268]
          tunnel: w1248 -> [w1266]
          tunnel: w1247 -> [w1265]
          tunnel: w1246 -> [w1264]
          frame #0 {
            n437 = while {
              tunnel: w1257 -> [w1261]
              tunnel: [w1259] -> w1258
              stop <- w1260 stop-if-true
              n438 = property class="Bool (strict)"(reference=w1261) -> (error out=w1259:errorcluster, "Value"=w1260:bool)  [unwired: 1 in, 1 out]
              n439 = Wait (ms)(milliseconds to wait=u32 200) -> ()  [unwired: 1 out]
            }
          }
          frame #1 {
            n440 = property class="Enum (strict)"(reference=w1274) -> ("Value"=w1267:T3)  [unwired: 1 in, 2 out]
            n441 = property class="Bool (strict)"(reference=w1272, "Value"=TRUE) -> (reference out=w1263:refnum<vi>)  [unwired: 1 in, 1 out]
            n442 = property class="Arr (strict)"(reference=w1268, "Value"=dbl[] [] ("Scalar")) -> ()  [unwired: 1 in, 2 out]
            n443 = property class="Arr (strict)"(reference=w1269, "Value"=i32[] []) -> ()  [unwired: 1 in, 2 out]
            n444 = case shown="\"Cell detected...\"" w1267 {
              tunnel: w1265 -> [_ w1280]
              tunnel: [w1275 user_message_v6."Cell detected..." ("f")] -> _
              tunnel: w1266 -> [_ w1281]
              tunnel: w1264 -> [_ w1279]
              tunnel: w1263 -> [_ w1278]
              tunnel: w1267 -> [w1275 _]
              frame "Initializing...", Default {
              }
              frame "Cell detected..." {
                (unwired) user_message_v6."DEBUG STATE" ("f")
                # "DEBUG MODE!"
                # "neuron found"
                n445 = property on="Property Node" class="Enum (strict)"(reference=w1279) -> ("Value"=w1277:T33)  [unwired: 1 in, 2 out]
                n446 = case shown="\"unreserve after cell found\"" w1277 {
                  tunnel: w1278 -> [_ w1283]
                  frame "unreserve after gross approach", Default {
                  }
                  frame "unreserve after cell found" {
                    n447 = property on="Property Node" class="Bool (strict)"(reference=w1283, "Value"=TRUE) -> ()  [unwired: 1 in, 2 out]
                  }
                }
                n448 = property on="Property Node" class="DigNum (strict)"(reference=w1281, "Val(Sgnl)"=w1280) -> ()  [unwired: 1 in, 2 out]
              }
            }
          }
        }
      }
      frame "In Process Calibration" {
        n449 = Unbundle By Name(w1289) -> ("misc indiv.State to advance to after Human Control"=w1288:refnum<vi>, "misc indiv.In Process Calibration?"=w1286:refnum<vi>)  [unwired: 1 out]
        n450 = call <vilib>:"Play Sound File.vi"("path"=path "C:/multiBot/patcherBot/sounds/LOZ-LA_Secret1.wav") -> ("error out"=w1285:errorcluster)  [unwired: 9 in, 1 out]
        n451 = flat-sequence {
          tunnel: [w1293] -> w1287
          tunnel: w1286 -> [w1292]
          tunnel: w1285 -> [w1291]
          tunnel: [user_message_v6."Starting new attempt..." ("Value")] -> w1290
          tunnel: w1287 -> [_]
          tunnel: w1288 -> [_]
          frame #0 {
            n452 = while {
              tunnel: w1292 -> [w1297]
              tunnel: [w1296] -> w1293
              tunnel: w1291 -> [w1294]
              stop <- w1295 continue-if-true
              n453 = property class="Bool (strict)"(reference=w1297, error in=w1294) -> (error out=w1296:errorcluster, "Value"=w1295:bool)  [unwired: 1 out]
              n454 = Wait (ms)(milliseconds to wait=u32 200) -> ()  [unwired: 1 out]
            }
          }
          frame #1 {
          }
        }
      }
      frame "Detecting cell..." {
        n455 = Unbundle By Name(w1321) -> ("cell tracker common.pipette_tracking_quality"=w1327:refnum<vi>, "cell tracker common.cell_tracking_quality"=w1326:refnum<vi>, "misc common.stage idle?"=w1320:refnum<vi>, "positioning+hunting common.NH method"=w1318:refnum<vi>, "positioning+hunting common.NH wait time (ms)"=w1312:refnum<vi>)
        n456 = property class="Arr (strict)"(reference=w1338) -> (reference out=w1300:refnum<vi>, "Value"=w1337:dbl[])  [unwired: 1 in, 1 out]
        n457 = property class="Arr (strict)"(reference=w1332, "Value"=dbl[] []) -> ()  [unwired: 1 in, 2 out]
        n458 = property class="Arr (strict)"(reference=w1336) -> (reference out=w1325:refnum<vi>, "Value"=w1339:dbl[])  [unwired: 1 in, 1 out]
        n459 = Unbundle By Name(w1319) -> ("state UI indiv.skip hunting"=w1335:refnum<vi>, "positioning + hunting indiv.NH step size (steps)"=w1333:refnum<vi>, "positioning + hunting indiv.NEURON HUNTING MONITOR"=w1330:refnum<vi>, "misc indiv.pipette broken - abort!"=w1329:refnum<vi>, "gigaseal indiv.start GS time"=w1328:refnum<vi>, "misc indiv.stage reservation options"=w1322:refnum<vi>)  [unwired: 1 out]
        n460 = Unbundle By Name(w1302) -> ("slice image"=w1301:T9)
        n461 = property class="Arr (strict)"(reference=w1314, "Value"=i32[] []) -> ()  [unwired: 1 in, 2 out]
        n462 = Wait (ms)(milliseconds to wait=u32 500) -> ()  [unwired: 1 out]
        n463 = property class="Bool (strict)"(reference=w1335) -> ("Value"=w1334:bool)  [unwired: 1 in, 2 out]
        n464 = property class="DigNum (strict)"(reference=w1316) -> ("Value"=w1315:dbl)  [unwired: 1 in, 2 out]
        n465 = case shown="False" w1334 {
          tunnel: w1315 -> [w1439 _]
          tunnel: w1337 -> [w1438 w1622]
          tunnel: w1339 -> [w1437 w1623]
          tunnel: [w1436 w1623] -> w1324
          tunnel: [w1435 w1622] -> w1323
          tunnel: w1342 -> [w1424 w1618]
          tunnel: w1347 -> [w1434 _]
          tunnel: w1346 -> [w1433 w1617]
          tunnel: [w1432 w1618] -> _
          tunnel: [w1431 w1617] -> w1306
          tunnel: [w1430 user_message_v6."Cell detected..." ("f")] -> w1308
          tunnel: w1344 -> [w1429 w1619]
          tunnel: w1343 -> [w1428 w1620]
          tunnel: [w1427 w1620] -> _
          tunnel: [w1426 w1619] -> _
          tunnel: w1310 -> [w1423 _]
          tunnel: w1341 -> [w1422 _]
          tunnel: w1340 -> [w1421 _]
          tunnel: w1333 -> [w1420 _]
          tunnel: w1319 -> [w1419 _]
          tunnel: w1321 -> [w1418 _]
          tunnel: w1330 -> [w1417 _]
          tunnel: w1329 -> [w1416 _]
          tunnel: w1328 -> [w1415 _]
          tunnel: w1327 -> [w1414 _]
          tunnel: w1326 -> [w1413 _]
          tunnel: w1322 -> [w1412 w1615]
          tunnel: w1320 -> [w1411 w1614]
          tunnel: w1319 -> [w1410 _]
          tunnel: w1318 -> [w1409 _]
          tunnel: w1317 -> [w1408 _]
          tunnel: w1310 -> [w1407 _]
          frame False {
            n466 = flat-sequence {
              tunnel: w1439 -> [w1487]
              tunnel: w1438 -> [w1486]
              tunnel: w1437 -> [w1474]
              tunnel: [w1485] -> w1446
              tunnel: [w1484] -> w1445
              tunnel: w1434 -> [w1483]
              tunnel: [w1482] -> w1444
              tunnel: w1433 -> [w1482]
              tunnel: [w1480] -> w1443
              tunnel: [w1481] -> w1442
              tunnel: w1429 -> [w1473]
              tunnel: w1428 -> [w1472]
              tunnel: [w1473] -> w1441
              tunnel: [w1472] -> w1440
              tunnel: [w1470] -> w1425
              tunnel: w1424 -> [w1470]
              tunnel: w1420 -> [w1466]
              tunnel: w1417 -> [w1464]
              tunnel: w1416 -> [w1462]
              tunnel: w1415 -> [w1447]
              tunnel: w1412 -> [w1460]
              tunnel: w1411 -> [w1459]
              tunnel: w1410 -> [w1458]
              tunnel: w1409 -> [w1449]
              tunnel: [w1517] -> w1435
              tunnel: [w1530] -> w1436
              tunnel: w1446 -> [w1530]
              tunnel: w1445 -> [w1517]
              tunnel: w1444 -> [w1528]
              tunnel: [w1527] -> w1432
              tunnel: [w1526] -> w1431
              tunnel: w1443 -> [w1516]
              tunnel: w1442 -> [w1529]
              tunnel: [w1529] -> w1430
              tunnel: w1441 -> [w1525]
              tunnel: w1440 -> [w1524]
              tunnel: [w1523] -> w1427
              tunnel: [w1522] -> w1426
              tunnel: w1425 -> [w1521]
              tunnel: w1423 -> [w1520]
              tunnel: w1422 -> [w1519]
              tunnel: w1421 -> [w1518]
              tunnel: w1419 -> [w1515]
              tunnel: w1418 -> [w1513]
              tunnel: w1414 -> [w1512]
              tunnel: w1413 -> [w1511]
              tunnel: w1408 -> [w1510]
              tunnel: w1407 -> [w1509]
              frame #0 {
                # "CONSTANT: UM/STEP"
                # "NEURON FOUND"
                # "current # steps taken"
                # "calc max steps you can take"
                n467 = Unbundle By Name(w1458) -> ("positioning + hunting indiv.Neuron Detection Threshold (MOhms)"=w1456:refnum<vi>, "positioning + hunting indiv.Pipette broken threshold (MOhms)"=w1453:refnum<vi>, "positioning + hunting indiv.Extra threshold (MOhms)"=w1454:refnum<vi>, "positioning + hunting indiv.max hunt distance (um)"=w1451:refnum<vi>)
                n468 = property class="DigNum (strict)"(reference=w1466) -> ("Value"=w1465:i32)  [unwired: 1 in, 2 out]
                n469 = property class="DigNum (strict)"(reference=w1451) -> ("Value"=w1450:dbl)  [unwired: 1 in, 2 out]
                n470 = Multiply(x=w1465, y=0.1) -> (x*y=w1467:dbl)
                n471 = Array Size(array=w1474) -> (size(s)=w1476:i32)
                n472 = Build Array (concatenate)(w1486, w1487) -> (w1484:dbl[])
                n473 = Divide(x=w1450, y=w1467) -> (x/y=w1479:dbl)
                n474 = Round Toward -Infinity(1:w1479) -> (0:w1478:dbl)
                n475 = property class="DigNum (strict)"(reference=w1454) -> ("Value"=w1455:dbl)  [unwired: 1 in, 2 out]
                n476 = property class="DigNum (strict)"(reference=w1456) -> ("Value"=w1457:dbl)  [unwired: 1 in, 2 out]
                n477 = property class="DigNum (strict)"(reference=w1453) -> ("Value"=w1452:dbl)  [unwired: 1 in, 2 out]
                n478 = property class="Enum (strict)"(reference=w1449) -> ("Value"=w1448:T34)  [unwired: 1 in, 2 out]
                n479 = To Long Integer(number=w1478) -> (32bit integer=w1477:i32)
                "max steps to take" <- w1477
                n480 = formula code="float depth;\ndepth=stepNum*NHstepsize_um;"("stepNum"=w1476, "NHstepsize_um"=w1467) -> ("depth"=w1475:dbl)
                n481 = Build Array (concatenate)(w1474, w1475) -> (w1485:dbl[])
                n482 = Bundle(w1485, w1484) -> (w1463:cluster{dbl[], dbl[]})  [unwired: 1 out]
                n483 = Greater Or Equal?(x=w1476, y=w1477) -> (x >= y?=w1471:bool)
                n484 = call "neuronFound.vi"("Pipette broken threshold (MOhms)"=w1452, "NH method"=w1448, "Extra threshold (MOhms)"=w1455, "Detection Threshold (MOhms)"=w1457, "R array"=w1484) -> ("pipette broken - abort!"=w1469:bool, "neuron found"=w1461:bool)  [unwired: 5 in]
                n485 = case shown="False" w1471 {
                  tunnel: w1483 -> [w1493 _]
                  tunnel: [w1492 user_message_v6."Unsuccessful breakin!" ("f")] -> w1481
                  tunnel: w1461 -> [w1491 _]
                  tunnel: w1447 -> [w1490 _]
                  tunnel: w1460 -> [w1489 w1505]
                  tunnel: w1459 -> [w1488 w1504]
                  frame False {
                    n486 = case shown="True" w1491 {
                      tunnel: w1493 -> [_ w1499]
                      tunnel: [user_message_v6."Detecting cell..." ("f") user_message_v6."Cell detected..." ("f")] -> w1492
                      tunnel: w1490 -> [_ w1500]
                      tunnel: w1489 -> [_ w1498]
                      tunnel: w1488 -> [_ w1497]
                      frame False {
                        # "No neuron ->\nkeep autopatching"
                      }
                      frame True {
                        (unwired) user_message_v6."DEBUG STATE" ("f")
                        # "DEBUG MODE!"
                        # "neuron found"
                        n487 = property on="Property Node" class="Enum (strict)"(reference=w1498) -> ("Value"=w1496:T33)  [unwired: 1 in, 2 out]
                        n488 = case shown="\"unreserve after cell found\"" w1496 {
                          tunnel: w1497 -> [_ w1502]
                          frame "unreserve after gross approach", Default {
                          }
                          frame "unreserve after cell found" {
                            n489 = property on="Property Node" class="Bool (strict)"(reference=w1502, "Value"=TRUE) -> ()  [unwired: 1 in, 2 out]
                          }
                        }
                        n490 = property on="Property Node" class="DigNum (strict)"(reference=w1500, "Val(Sgnl)"=w1499) -> ()  [unwired: 1 in, 2 out]
                      }
                    }
                  }
                  frame True {
                    (unwired) user_message_v6."DEBUG STATE" ("f")
                    # "Reached end -> unsuccessful"
                    n491 = property on="Property Node" class="Enum (strict)"(reference=w1505) -> ("Value"=w1506:T33)  [unwired: 1 in, 2 out]
                    n492 = case shown="\"unreserve after cell found\"" w1506 {
                      tunnel: w1504 -> [_ w1508]
                      frame "unreserve after gross approach", Default {
                      }
                      frame "unreserve after cell found" {
                        n493 = property on="Property Node" class="Bool (strict)"(reference=w1508, "Value"=TRUE) -> ()  [unwired: 1 in, 2 out]
                      }
                    }
                  }
                }
                n494 = property class="XYGraph (strict)"(reference=w1464, "Value"=w1463) -> ()  [unwired: 1 in, 2 out]
                n495 = Or(x=w1471, y=w1461) -> (x .or. y?=w1480:bool)
                n496 = property on="Property Node" class="Bool (strict)"(reference=w1462, "Val(Sgnl)"=w1469) -> ()  [unwired: 1 in, 2 out]
              }
              frame #1 {
                # "Step by x um each step\nin approach mode"
                n497 = Unbundle By Name(w1515) -> ("state UI indiv.cell tracker"=w1514:refnum<vi>)
                n498 = case shown="True" w1516 {
                  tunnel: w1528 -> [w1550 w1576]
                  tunnel: [w1549 w1578] -> w1527
                  tunnel: [w1548 w1581] -> w1526
                  tunnel: w1525 -> [w1542 w1583]
                  tunnel: w1524 -> [w1543 w1584]
                  tunnel: [w1543 w1584] -> w1523
                  tunnel: [w1542 w1583] -> w1522
                  tunnel: w1521 -> [w1547 w1571]
                  tunnel: w1520 -> [w1544 w1580]
                  tunnel: w1519 -> [w1545 w1582]
                  tunnel: w1518 -> [w1546 w1579]
                  tunnel: w1514 -> [w1541 w1575]
                  tunnel: w1513 -> [w1536 w1573]
                  tunnel: w1512 -> [w1540 _]
                  tunnel: w1511 -> [w1539 _]
                  tunnel: w1510 -> [_ _]
                  tunnel: w1509 -> [w1533 _]
                  frame False {
                    # "pipette tracking quality"
                    # "cell tracking quality"
                    # "IF cell tracking\nTHEN\nhybrid move"
                    # "Neuron not found"
                    n499 = property class="Bool (strict)"(reference=w1541) -> ("Value"=w1531:bool)  [unwired: 1 in, 2 out]
                    n500 = property on="Property Node" class="DigNum (strict)"(reference=w1540) -> ("Value"=w1538:dbl)  [unwired: 1 in, 2 out]
                    n501 = property on="Property Node" class="DigNum (strict)"(reference=w1539) -> ("Value"=w1537:dbl)  [unwired: 1 in, 2 out]
                    n502 = Unbundle By Name(w1536) -> ("cell tracker common.centroid_px"=w1535:refnum<vi>, "vision common.current pipette locations (px)"=w1532:refnum<vi>)  [unwired: 1 out]
                    n503 = Not Equal To 0?(x=w1538) -> ()  [unwired: 1 out]
                    n504 = Not Equal To 0?(x=w1537) -> (x != 0?=w1534:bool)
                    n505 = And(x=w1531, y=w1534) -> ()  [unwired: 1 out]
                    n506 = case shown="False" w1531 {
                      tunnel: w1547 -> [w1555 w1563]
                      tunnel: w1550 -> [w1554 w1562]
                      tunnel: [w1553 w1563] -> w1549
                      tunnel: [w1552 w1562] -> w1548
                      tunnel: w1546 -> [_ w1566]
                      tunnel: w1545 -> [_ w1565]
                      tunnel: w1544 -> [_ w1564]
                      tunnel: w1535 -> [_ w1561]
                      tunnel: w1533 -> [_ w1558]
                      tunnel: w1532 -> [_ w1557]
                      frame False {
                        # "step down"
                        n507 = call "take step fast.vi"("blocking?"=TRUE, "error in"=w1554, "actuator in"=w1555) -> ("error out"=w1552:errorcluster, "actuator out"=w1553:T25)  [unwired: 7 in]
                      }
                      frame True {
                        # "this moves laterally AND vertically down\ndepending on conditions"
                        n508 = property on="Property Node" class="Arr (strict)"(reference=w1557) -> ("Value"=w1559:dbl[][])  [unwired: 1 in, 2 out]
                        n509 = property on="Property Node" class="Arr (strict)"(reference=w1561) -> ("Value"=w1560:dbl[])  [unwired: 1 in, 2 out]
                        n510 = Index Array(array=w1559, index (row)=w1558) -> (element=w1556:dbl[])  [unwired: 1 in]
                        n511 = call "calc_NH_vector.vi"("current pipette location (px)"=w1556, "which manipulator"=w1564, "cell tracker movement options"="cell tracker movement options", "transform cluster + actuator"=w1566, "cell centroid (px)"=w1560) -> ("rel move vector (steps)"=w1568:dbl[])  [unwired: 6 in]
                        "rel move vector (steps)" <- w1568
                        n512 = call "move manipulator rel.vi"("blocking?"=TRUE, "which manipulator"=w1564, "transform cluster + actuator"=w1566, "positions"=w1565, "location (steps)"=w1568) -> ()  [unwired: 6 in, 1 out]
                      }
                    }
                  }
                  frame True {
                    # "neuron found or reached end"
                    n513 = property on="Property Node" class="Bool (strict)"(reference=w1575) -> ("Value"=w1574:bool)  [unwired: 1 in, 2 out]
                    n514 = call "reset manipulator.vi"("error in"=w1576, "approach? (T = on)"=FALSE, "motion"=scope_motion."slow", "manip in"=w1571) -> ("manip out"=w1572:T25)  [unwired: 6 in, 1 out]
                    n515 = case shown="False" w1574 {
                      tunnel: w1582 -> [_ _]
                      tunnel: w1576 -> [w1592 w1610]
                      tunnel: [w1597 w1610] -> w1581
                      tunnel: w1580 -> [_ _]
                      tunnel: w1579 -> [_ _]
                      tunnel: w1572 -> [w1591 w1611]
                      tunnel: [w1596 w1611] -> w1578
                      tunnel: w1573 -> [_ w1606]
                      frame False {
                        w1594 = 0.0 ("element")
                        n516 = Build Array(w1594, w1594, 10.0 ("element")) -> (w1593:dbl[])
                        n517 = To Long Integer(number=w1593) -> (32bit integer=w1590:i32[])
                        n518 = call "moveTo_rel_XYZ.vi"("blocking?"=TRUE, "error in"=w1592, "XYZ location (steps)"=w1590, "Actuator cluster in"=w1591) -> ("error out"=w1586:errorcluster, "Actuator cluster out"=w1588:T25)  [unwired: 6 in]
                        n519 = call "Time Delay35"("error in (no error)"=w1586, "Delay Time (s)"=0.2) -> ("error out"=w1585:errorcluster)  [unwired: 9 in]
                        n520 = call "reset manipulator.vi"("error in"=w1585, "approach? (T = on)"=FALSE, "motion"=scope_motion."slow", "manip in"=w1588) -> ("error out"=w1597:errorcluster, "manip out"=w1596:T25)  [unwired: 6 in]
                      }
                      frame True {
                        w1605 = FALSE ("tracking")
                        # "stop Neuron Hunt"
                        n521 = Unbundle By Name(w1606) -> ("vision common.init tracker success"=w1609:refnum<vi>, "vision common.run tracker success"=w1608:refnum<vi>, "vision common.tracking"=w1607:refnum<vi>, "vision common.exit tracker success"=w1602:refnum<vi>)
                        n522 = property class="Bool (strict)"(reference=w1609, "Value"=w1605) -> (error out=w1604:errorcluster)  [unwired: 1 in, 1 out]
                        n523 = property class="Bool (strict)"(reference=w1608, "Value"=w1605) -> ()  [unwired: 1 in, 2 out]
                        n524 = property class="Bool (strict)"(reference=w1607, "Value"=w1605) -> ()  [unwired: 1 in, 2 out]
                        n525 = call "Time Delay13"("error in (no error)"=w1604, "Delay Time (s)"=1.0) -> ("error out"=w1612:errorcluster)  [unwired: 9 in]
                        n526 = script code="% run exit script\nclearvars -except pipette_segmentation Pipette Pipette_tip Pipette_seg pipette_image\nexit_cellTracker_flag = 0;\nexit_cellTracker;"("??"=w1612) -> ("??"=w1601:errorcluster, "exit_cellTracker_flag"=w1613:dbl)
                        n527 = Not Equal To 0?(x=w1613) -> (x != 0?=w1600:bool)
                        n528 = property class="Bool (strict)"(reference=w1602, error in=w1601, "Value"=w1600) -> ()  [unwired: 2 out]
                      }
                    }
                  }
                }
              }
            }
          }
          frame True {
            n529 = property on="Property Node" class="Enum (strict)"(reference=w1615) -> ("Value"=w1616:T33)  [unwired: 1 in, 2 out]
            n530 = case shown="\"unreserve after cell found\"" w1616 {
              tunnel: w1614 -> [_ w1625]
              frame "unreserve after gross approach", Default {
              }
              frame "unreserve after cell found" {
                n531 = property on="Property Node" class="Bool (strict)"(reference=w1625, "Value"=TRUE) -> ()  [unwired: 1 in, 2 out]
              }
            }
          }
        }
        n532 = property class="Arr (strict)"(reference=w1300, "Value"=w1323) -> ()  [unwired: 1 in, 2 out]
        n533 = property class="Arr (strict)"(reference=w1325, "Value"=w1324) -> ()  [unwired: 1 in, 2 out]
        n534 = property class="DigNum (strict)"(reference=w1312) -> ("Value"=w1311:u32)  [unwired: 1 in, 2 out]
        n535 = case shown="\"Cell detected...\"" w1308 {
          tunnel: w1307 -> [_ w1361]
          tunnel: w1301 -> [_ w1363]
          tunnel: w1306 -> [w1348 w1356]
          tunnel: w1305 -> [_ w1362]
          tunnel: w1304 -> [_ w1360]
          tunnel: [w1348 w1349] -> w1303
          frame "Initializing...", Default {
          }
          frame "Cell detected..." {
            w1357 = T28 7 items=["Grayscale (U8)", "Grayscale (I16)", "Grayscale (SGL)", "Complex (CSG)", "RGB (U32)", "HSL (U32)", "RGB (U64)", "Grayscale (U16)"] ("Image Type")
            # "create image buffer"
            n536 = call "IMAQ Create"("Border Size"=0, "Image Name"="temp", "Image Type"=w1357, "error in (no error)"=w1356) -> ("New Image"=w1354:T9, "error out"=w1355:errorcluster)  [unwired: 1 in]
            n537 = while {
              tunnel: w1363 -> [w1392]
              tunnel: w1361 -> [w1406]
              tunnel: w1362 -> [w1386]
              tunnel: [w1382] -> w1350
              tunnel: w1355 -> [w1385]
              tunnel: "images/04-beforeSeal.png" ("name or relative path") -> [w1403]
              tunnel: w1360 -> [w1401]
              tunnel: [w1383] -> w1353
              tunnel: [w1381] -> w1352
              tunnel: [w1380] -> w1351
              stop <- w1402 stop-if-true
              n538 = property class="Bool (strict)"(reference=w1401) -> ("Value"=w1400:bool)  [unwired: 1 in, 2 out]
              n539 = call "IMAQ GetImageSize"("Image"=w1392, "error in (no error)"=w1385) -> ("Y Resolution"=w1396:i32, "X Resolution"=w1399:i32, "error out"=w1391:errorcluster)  [unwired: 2 in]
              n540 = call "IMAQ ImageToArray"("error in (no error)"=w1391, "Image"=w1392) -> ("Image Pixels (U16)"=w1380:u16[][], "error out"=w1382:errorcluster)  [unwired: 2 in, 3 out]
              n541 = Add Array Elements(numeric array=w1380) -> (sum=w1390:u16)
              n542 = Build Path(base path=w1406, name or relative path=w1403) -> (appended path=w1381:path)
              n543 = Index Array(array=w1386) -> (element #1=w1398:i32, element #2=w1397:i32)  [unwired: 2 in]
              n544 = Equal?(x=w1396, y=w1397) -> (x = y?=w1394:bool)
              n545 = Greater?(x=w1390, y=u16 0) -> (0:w1387:bool)
              n546 = Equal?(x=w1399, y=w1398) -> (x = y?=w1395:bool)
              n547 = And(x=w1395, y=w1394) -> (x .and. y?=w1388:bool)
              n548 = Wait (ms)(milliseconds to wait=u32 1000) -> ()  [unwired: 1 out]
              n549 = And(x=w1388, y=w1387) -> (x .and. y?=w1384:bool)
              n550 = Select(t="Ready", s=w1384, f="Before") -> (s? t:f=w1383:string)
              n551 = Or(x=w1384, y=w1400) -> (x .or. y?=w1402:bool)
            }
            n552 = case shown="\"Ready\"" w1353 {
              tunnel: w1352 -> [_ w1376 _]
              tunnel: [FALSE TRUE FALSE] -> _
              tunnel: w1350 -> [w1365 w1370 w1378]
              tunnel: [w1365 w1368 w1378] -> w1349
              tunnel: w1354 -> [_ w1373 _]
              tunnel: w1351 -> [_ w1367 _]
              frame "Before", Default {
              }
              frame "Ready" {
                n553 = call "IMAQ ArrayToImage"("Image Pixels (U16)"=w1367, "error in (no error)"=w1370, "Image"=w1373) -> ("error out"=w1374:errorcluster, "Image Out"=w1371:T9)  [unwired: 7 in]
                n554 = call-poly "IMAQ Write File 2"("error in (no error)"=w1374, "Image Quality"=u32 1000, "File Path"=w1376, "Image"=w1371) -> ("error out"=w1369:errorcluster)  [unwired: 6 in, 1 out]
                n555 = call "IMAQ Dispose"("All Images? (No)"=FALSE, "Image"=w1371, "error in (no error)"=w1369) -> ("error out"=w1368:errorcluster)  [unwired: 3 in]
              }
              frame "After" {
              }
            }
          }
        }
        n556 = Wait (ms)(milliseconds to wait=w1311) -> ()  [unwired: 1 out]
      }
      frame "Cell detected..." {
        # "The timing here requires the two wait functions\nto total 1 second and also uses the iteration count to \ndetermine the start time..."
        n557 = Wait (ms)(milliseconds to wait=u32 500) -> ()  [unwired: 1 out]
        n558 = property class="Arr (strict)"(reference=w1648) -> (reference out=w1643:refnum<vi>, "Value"=w1647:i32[])  [unwired: 1 in, 1 out]
        n559 = property class="Arr (strict)"(reference=w1646) -> (reference out=w1644:refnum<vi>, "Value"=w1645:dbl[])  [unwired: 1 in, 1 out]
        n560 = Unbundle By Name(w1634) -> ("misc common.mclamp cluster"=w1633:refnum<vi>)
        n561 = Unbundle By Name(w1652) -> ("gigaseal indiv.vhold applied?"=w1651:refnum<vi>, "state UI indiv.skip gigasealing"=w1642:refnum<vi>, "gigaseal indiv.GS timeout (adjusted)"=w1640:refnum<vi>, "gigaseal indiv.holding V (mV)"=w1639:refnum<vi>, "gigaseal indiv.GIGASEALING MONITOR"=w1638:refnum<vi>, "gigaseal indiv.start GS time"=w1637:refnum<vi>, "gigaseal indiv.GS extended"=w1636:refnum<vi>, "gigaseal indiv.current Vholding (mV)"=w1632:refnum<vi>, "gigaseal indiv.gigasealing options"=w1631:refnum<vi>, "gigaseal indiv.Cm"=w1628:refnum<vi>, "gigaseal indiv.Ra"=w1627:refnum<vi>)  [unwired: 1 out]
        n562 = property class="Bool (strict)"(reference=w1642) -> ("Value"=w1641:bool)  [unwired: 1 in, 2 out]
        n563 = property class="Bool (strict)"(reference=w1651) -> (reference out=w1649:refnum<vi>, "Value"=w1650:bool)  [unwired: 1 in, 1 out]
        n564 = property class="DigNum (strict)"(reference=w1630) -> ("Value"=w1629:dbl)  [unwired: 1 in, 2 out]
        n565 = case shown="False" w1641 {
          tunnel: w1647 -> [w1709 _]
          tunnel: w1660 -> [w1708 _]
          tunnel: [T13."Disabled and Grayed Out" ("Disabled") T13."Disabled and Grayed Out" ("Disabled")] -> w1659
          tunnel: w1645 -> [w1704 _]
          tunnel: w1658 -> [w1670 _]
          tunnel: w1657 -> [w1703 _]
          tunnel: w1656 -> [w1702 _]
          tunnel: w1655 -> [w1701 _]
          tunnel: w1654 -> [w1700 _]
          tunnel: [w1698 user_message_v6."Gigaseal Established..." ("state out")] -> w1653
          tunnel: w1629 -> [w1661 _]
          tunnel: w1650 -> [w1671 _]
          tunnel: w1649 -> [w1692 _]
          tunnel: w1644 -> [w1689 _]
          tunnel: w1643 -> [w1688 _]
          tunnel: w1640 -> [w1676 _]
          tunnel: w1639 -> [w1686 _]
          tunnel: w1638 -> [w1683 _]
          tunnel: w1637 -> [w1681 _]
          tunnel: w1636 -> [w1678 _]
          tunnel: w1635 -> [w1674 _]
          tunnel: w1633 -> [w1675 _]
          tunnel: w1632 -> [w1673 _]
          tunnel: w1631 -> [w1667 _]
          tunnel: w1628 -> [w1665 _]
          tunnel: w1627 -> [w1664 _]
          frame False {
            # "apply holding voltage once - if we just crossed the resistance threshold"
            # "REPLACE"
            # "if R > 400 MOHMS, add 60 s to the GS timeout"
            # "In gigasealing subVI, make it so pressure goes to atmospheric and V = -70 mV\nas soon as resistance tapers out at 1 GOhm\n\nSTATES: \nGigaohm established in < XXX seconds --> \"Gigaseal established\"\nXXX seconds elapsed with no Gigaohm --> \"Retract and quit\"\nt < XXX seconds --> \"Found neuron. Sealing...\""
            n566 = property class="DigNum (strict)"(reference=w1681) -> ("Value"=w1680:i32)  [unwired: 1 in, 2 out]
            n567 = property class="Bool (strict)"(reference=w1678) -> (reference out=w1677:refnum<vi>, "Value"=w1679:bool)  [unwired: 1 in, 1 out]
            n568 = property class="Clust (strict)"(reference=w1667) -> ("Value"=w1666:T35)  [unwired: 1 in, 2 out]
            n569 = property class="DigNum (strict)"(reference=w1665) -> ("Value"=w1663:dbl)  [unwired: 1 in, 2 out]
            n570 = property class="DigNum (strict)"(reference=w1664) -> ("Value"=w1662:dbl)  [unwired: 1 in, 2 out]
            n571 = property class="DigNum (strict)"(reference=w1676) -> ("Value"=w1687:i32)  [unwired: 1 in, 2 out]
            n572 = Greater?(x=w1661, y=400.0 ("x")) -> (0:w1696:bool)
            n573 = Not(x=w1679) -> (.not. x?=w1695:bool)
            n574 = Subtract(x=w1708, y=w1680) -> (x-y=w1705:i32)
            n575 = And(x=w1695, y=w1696) -> (x .and. y?=w1694:bool)
            n576 = Build Array (concatenate)(w1704, w1661) -> (w1690:dbl[])
            n577 = property class="DigNum (strict)"(reference=w1686) -> ("Value"=w1685:dbl)  [unwired: 1 in, 2 out]
            n578 = Build Array (concatenate)(w1709, w1705) -> (w1691:i32[])
            n579 = case shown="True" w1694 {
              tunnel: w1687 -> [_ w1715]
              tunnel: w1677 -> [_ w1713]
              tunnel: w1676 -> [_ w1710]
              frame False {
              }
              frame True {
                n580 = Add(x=60, y=w1715) -> (x+y=w1711:i32)
                n581 = property class="DigNum (strict)"(reference=w1710, "Value"=w1711) -> ()  [unwired: 1 in, 2 out]
                n582 = property class="Bool (strict)"(reference=w1713, "Value"=TRUE ("extend GS")) -> ()  [unwired: 1 in, 2 out]
              }
            }
            n583 = Bundle(w1691, w1690) -> (w1682:cluster{i32[], dbl[]})  [unwired: 1 out]
            n584 = call "gigasealing_v7.vi"("Pressure box control in"=w1701, "holding V (mV)"=w1685, "Cm"=w1663, "Ra"=w1662, "apply suction"=FALSE, "gigasealing array"=w1704, "Slide Refnum"=w1700, "gigasealing options"=w1666, "Rm"=w1661, "GS timeout"=w1687, "vhold applied?"=w1671, "which manipulator"=w1674) -> ("set pressure"=→"set pressure":dbl, "Vholding (mV)"=w1684:dbl, "vhold applied"=w1672:bool, "state out"=w1698:T3)  [unwired: 4 in]
            n585 = property class="DigNum (strict)"(reference=w1673, "Value"=w1684) -> ()  [unwired: 1 in, 2 out]
            n586 = property class="XYGraph (strict)"(reference=w1683, "Value"=w1682) -> ()  [unwired: 1 in, 2 out]
            n587 = Compound Arithmetic op=AND(w1672, invert w1671) -> (w1669:bool)
            n588 = And(x=w1670, y=w1669) -> (x .and. y?=w1668:bool)
            n589 = property class="Bool (strict)"(reference=w1692, "Value"=w1672) -> ()  [unwired: 1 in, 2 out]
            n590 = case shown="True" w1668 {
              tunnel: w1703 -> [_ _]
              tunnel: w1702 -> [_ w1721]
              tunnel: w1684 -> [_ w1725]
              tunnel: w1675 -> [_ w1723]
              tunnel: w1674 -> [_ w1719]
              frame False {
              }
              frame True {
                # "SELECT MCLAMP FIRST!"
                # "set offset"
                n591 = property class="Clust (strict)"(reference=w1723) -> (error out=w1716:errorcluster, "Value"=w1722:T29)  [unwired: 1 in, 1 out]
                n592 = call "select_mclamp_channel.vi"("which manipulator"=w1719, "error in (no error)"=w1716, "mclamp cluster"=w1722, "Multiclamp Handle In"=w1721) -> ("error out"=w1717:errorcluster, "error"=w1718:i32, "Multiclamp Handle out"=w1720:u32)  [unwired: 5 in]
                n593 = Divide(x=w1725, y=1000.0) -> (x/y=w1724:dbl)
                n594 = dll-call lib="C:/multiBot/patcherBot/AxMultiClampMsg.dll" fn="MCCMSG_SetHolding"(error in=w1717, "handle"=w1720, "ModeConstant"=w1724, "error"=w1718) -> ()  [unwired: 6 in, 2 out]
              }
            }
            n595 = Wait (ms)(milliseconds to wait=u32 500) -> ()  [unwired: 1 out]
            n596 = property class="Arr (strict)"(reference=w1688, "Value"=w1691) -> ()  [unwired: 1 in, 2 out]
            n597 = property class="Arr (strict)"(reference=w1689, "Value"=w1690) -> ()  [unwired: 1 in, 2 out]
          }
          frame True {
          }
        }
      }
      frame "Gigaseal Established..." {
        w1739 = T28 7 items=["Grayscale (U8)", "Grayscale (I16)", "Grayscale (SGL)", "Complex (CSG)", "RGB (U32)", "HSL (U32)", "RGB (U64)", "Grayscale (U16)"] ("Image Type")
        # "create image buffer"
        n598 = Unbundle By Name(w1753) -> ("misc common.mclamp cluster"=w1752:refnum<vi>)
        n599 = Unbundle By Name(w1761) -> ("misc indiv.other state ref"=w1750:refnum<vi>, "gigaseal indiv.holding V (mV)"=w1756:refnum<vi>, "state UI indiv.skip to unsuccessful breakin"=w1760:refnum<vi>, "state UI indiv.skip to successful breakin"=w1759:refnum<vi>, "positioning + hunting indiv.Memtest inputs"=w1755:refnum<vi>, "breakin indiv.MAX Break In Pressure (mbar)"=w1751:refnum<vi>)
        n600 = Unbundle By Name(w1730) -> ("slice image"=w1729:T9)
        n601 = call "IMAQ Create"("Border Size"=0, "Image Name"="temp", "Image Type"=w1739, "error in (no error)"=w1733) -> ("New Image"=w1734:T9, "error out"=w1732:errorcluster)  [unwired: 1 in]
        n602 = Wait (ms)(milliseconds to wait=u32 500) -> ()  [unwired: 1 out]
        n603 = while {
          tunnel: w1729 -> [w1798]
          tunnel: w1743 -> [w1812]
          tunnel: w1744 -> [w1791]
          tunnel: [w1789] -> w1738
          tunnel: w1732 -> [w1797]
          tunnel: "images/05-gigaSeal.png" ("name or relative path") -> [w1809]
          tunnel: w1742 -> [w1807]
          tunnel: [w1790] -> w1736
          tunnel: [w1788] -> w1735
          tunnel: [w1786] -> w1731
          stop <- w1808 stop-if-true
          n604 = property class="Bool (strict)"(reference=w1807) -> ("Value"=w1806:bool)  [unwired: 1 in, 2 out]
          n605 = call "IMAQ GetImageSize"("Image"=w1798, "error in (no error)"=w1797) -> ("Y Resolution"=w1802:i32, "X Resolution"=w1805:i32, "error out"=w1796:errorcluster)  [unwired: 2 in]
          n606 = call "IMAQ ImageToArray"("error in (no error)"=w1796, "Image"=w1798) -> ("Image Pixels (U16)"=w1788:u16[][], "error out"=w1789:errorcluster)  [unwired: 2 in, 3 out]
          n607 = Add Array Elements(numeric array=w1788) -> (sum=w1795:u16)
          n608 = Build Path(base path=w1812, name or relative path=w1809) -> (appended path=w1790:path)
          n609 = Index Array(array=w1791) -> (element #1=w1804:i32, element #2=w1803:i32)  [unwired: 2 in]
          n610 = Equal?(x=w1802, y=w1803) -> (x = y?=w1800:bool)
          n611 = Greater?(x=w1795, y=u16 0) -> (0:w1792:bool)
          n612 = Equal?(x=w1805, y=w1804) -> (x = y?=w1801:bool)
          n613 = And(x=w1801, y=w1800) -> (x .and. y?=w1793:bool)
          n614 = Wait (ms)(milliseconds to wait=u32 1000) -> ()  [unwired: 1 out]
          n615 = And(x=w1793, y=w1792) -> (x .and. y?=w1787:bool)
          n616 = Select(t="Ready", s=w1787, f="Before") -> (s? t:f=w1786:string)
          n617 = Or(x=w1787, y=w1806) -> (x .or. y?=w1808:bool)
        }
        n618 = property class="Bool (strict)"(reference=w1760) -> ("Value"=w1757:bool)  [unwired: 1 in, 2 out]
        n619 = property class="Bool (strict)"(reference=w1759) -> ("Value"=w1758:bool)  [unwired: 1 in, 2 out]
        n620 = case shown="\"Ready\"" w1731 {
          tunnel: w1736 -> [_ w1782 _]
          tunnel: [FALSE TRUE FALSE] -> _
          tunnel: w1738 -> [w1771 w1775 w1784]
          tunnel: [w1771 w1773 w1784] -> w1737
          tunnel: w1735 -> [_ w1779 _]
          tunnel: w1734 -> [_ w1778 _]
          frame "Before", Default {
          }
          frame "Ready" {
            n621 = call "IMAQ ArrayToImage"("Image Pixels (U16)"=w1779, "error in (no error)"=w1775, "Image"=w1778) -> ("error out"=w1780:errorcluster, "Image Out"=w1776:T9)  [unwired: 7 in]
            n622 = call-poly "IMAQ Write File 2"("error in (no error)"=w1780, "Image Quality"=u32 1000, "File Path"=w1782, "Image"=w1776) -> ("error out"=w1774:errorcluster)  [unwired: 6 in, 1 out]
            n623 = call "IMAQ Dispose"("All Images? (No)"=FALSE, "Image"=w1776, "error in (no error)"=w1774) -> ("error out"=w1773:errorcluster)  [unwired: 3 in]
          }
          frame "After" {
          }
        }
        n624 = call "Time Delay29"("error in (no error)"=w1737, "Delay Time (s)"=0.2) -> ("error out"=w1746:errorcluster)  [unwired: 9 in]
        n625 = Or(x=w1757, y=w1758) -> (x .or. y?=w1762:bool)
        n626 = case shown="False" w1762 {
          tunnel: [w1825 w1885] -> w1770
          tunnel: [w1816 w1889] -> _
          tunnel: w1769 -> [w1833 w1889]
          tunnel: [w1818 _] -> w1768
          tunnel: w1767 -> [w1839 _]
          tunnel: w1766 -> [w1836 _]
          tunnel: w1765 -> [w1835 _]
          tunnel: w1746 -> [w1831 _]
          tunnel: w1763 -> [w1815 _]
          tunnel: w1758 -> [_ w1888]
          tunnel: w1756 -> [w1830 _]
          tunnel: w1755 -> [w1829 _]
          tunnel: w1754 -> [w1814 _]
          tunnel: w1752 -> [w1828 _]
          tunnel: w1751 -> [w1813 _]
          tunnel: w1750 -> [w1826 _]
          tunnel: w1749 -> [w1823 _]
          frame False {
            # "setting valves to atm pressure"
            # "=== simultaneous break-in ======\nif other state = \"waiting\"\nstart break in and other state should start break-in\n\nelse\nwait to break in"
            # "fast/slow capacitance compensation"
            # "setting valves to atm pressure"
            # "set breakin pressure.\n8-24-16: removed. the pulse pressure VI should do this already"
            n627 = property class="DigNum (strict)"(reference=w1813) -> ("Value"=w1827:dbl)  [unwired: 1 in, 2 out]
            n628 = disable-structure shown="Enabled" {
              disable-tunnel: [w1858 w1859] -> w1842
              disable-tunnel: w1833 -> [w1857 w1860]
              disable-tunnel: [w1856 w1860] -> w1817
              disable-tunnel: w1831 -> [w1855 w1859]
              disable-tunnel: w1815 -> [w1854 _]
              disable-tunnel: w1814 -> [w1853 _]
              disable-tunnel: w1827 -> [w1852 _]
              frame Disabled {
                n629 = call "prepBreakIn_toplvl.vi"("which manipulator"=w1853, "Slide Refnum"=w1854, "error in (no error)"=w1855, "Break In Pressure (mbar)"=w1852, "Pressure box control in"=w1857) -> ("error out"=w1858:errorcluster, "Pressure box control out"=w1856:T22)  [unwired: 5 in]
              }
              frame Enabled {
              }
            }
            n630 = call "Time Delay14"("error in (no error)"=w1842, "Delay Time (s)"=1.0) -> ("error out"=w1837:errorcluster)  [unwired: 9 in]
            n631 = case shown="True" w1839 {
              tunnel: [w1868 w1882] -> w1838
              tunnel: w1837 -> [w1868 w1875]
              tunnel: w1836 -> [_ w1879]
              tunnel: w1835 -> [_ _]
              tunnel: w1830 -> [_ w1881]
              tunnel: w1814 -> [_ w1878]
              tunnel: w1828 -> [_ w1877]
              frame False {
              }
              frame True {
                # "SELECT MCLAMP FIRST!"
                n632 = property class="Clust (strict)"(reference=w1877) -> ("Value"=w1876:T29)  [unwired: 1 in, 2 out]
                n633 = call "select_mclamp_channel.vi"("which manipulator"=w1878, "error in (no error)"=w1875, "mclamp cluster"=w1876, "Multiclamp Handle In"=w1879) -> ("error out"=w1874:errorcluster, "error"=w1869:i32, "Multiclamp Handle out"=w1870:u32)  [unwired: 5 in]
                n634 = call "mclamp_zero_pipetteCap.vi"("error in (no error)"=w1874, "Error in"=w1869, "Multiclamp Handle Out"=w1870) -> ("error out"=w1871:errorcluster, "slow comp (pF)"=→"slow comp (pF)":dbl, "fast comp (pF)"=→"fast comp (pF)":dbl)  [unwired: 6 in]
                n635 = property class="DigNum (strict)"(reference=w1881) -> ("Value"=w1880:dbl)  [unwired: 1 in, 2 out]
                n636 = Divide(x=w1880, y=1000.0) -> (x/y=w1884:dbl)
                n637 = dll-call lib="C:/multiBot/patcherBot/AxMultiClampMsg.dll" fn="MCCMSG_SetHolding"(error in=w1871, "handle"=w1870, "ModeConstant"=w1884, "error"=w1869) -> (error out=w1882:errorcluster)  [unwired: 6 in, 1 out]
              }
            }
            n638 = call "Time Delay15"("error in (no error)"=w1838, "Delay Time (s)"=3.0) -> ("error out"=w1832:errorcluster)  [unwired: 9 in]
            n639 = property class="Bool (strict)"(reference=w1823) -> ("Value"=w1824:bool)  [unwired: 1 in, 2 out]
            n640 = property on="Property Node" class="Clust (strict)"(reference=w1829, error in=w1832, "Val(Sgnl)"="GS memtest inputs") -> (error out=w1819:errorcluster)  [unwired: 1 out]
            n641 = case shown="True" w1824 {
              tunnel: w1826 -> [_ w1867]
              tunnel: [user_message_v6."Breaking in..." ("state out") w1862] -> w1825
              frame False {
              }
              frame True {
                w1863 = user_message_v6."Waiting to break in..." ("Value")
                n642 = property on="Property Node" class="Enum (strict)"(reference=w1867) -> ("Value"=w1866:T3)  [unwired: 1 in, 2 out]
                n643 = Equal?(x=w1866, y=w1863) -> (x = y?=w1865:bool)
                n644 = Select(t=user_message_v6."Breaking in..." ("Value"), s=w1865, f=w1863) -> (s? t:f=w1862:T3)
              }
            }
            n645 = property class="DigNum (strict)"(reference=w1813) -> ("Value"=w1820:dbl)  [unwired: 1 in, 2 out]
            n646 = disable-structure shown="Enabled" {
              disable-tunnel: [w1849 w1850] -> w1822
              disable-tunnel: w1817 -> [w1848 w1851]
              disable-tunnel: [w1847 w1851] -> w1816
              disable-tunnel: w1819 -> [w1846 w1850]
              disable-tunnel: w1815 -> [w1845 _]
              disable-tunnel: w1814 -> [w1844 _]
              disable-tunnel: w1820 -> [w1843 _]
              frame Disabled {
                n647 = call "prepBreakIn_toplvl.vi"("which manipulator"=w1844, "Slide Refnum"=w1845, "error in (no error)"=w1846, "Break In Pressure (mbar)"=w1843, "Pressure box control in"=w1848) -> ("error out"=w1849:errorcluster, "Pressure box control out"=w1847:T22)  [unwired: 5 in]
              }
              frame Enabled {
              }
            }
            n648 = call "Time Delay27"("error in (no error)"=w1822, "Delay Time (s)"=1.0) -> ("error out"=w1818:errorcluster)  [unwired: 9 in]
          }
          frame True {
            n649 = Select(t=user_message_v6."Successful breakin!" ("state out"), s=w1888, f=user_message_v6."Unsuccessful breakin!" ("state out")) -> (s? t:f=w1885:T3)
          }
        }
      }
      frame "Breaking in..." {
        w1918 = 0.0 ("set pressure (mBar)")
        # "setting valves to atm pressure"
        # "save transients"
        n650 = Unbundle By Name(w1921) -> ("breakin indiv.MAX Break In Pressure (mbar)"=w1920:refnum<vi>, "misc indiv.Break-In Counter"=w1899:refnum<vi>)  [unwired: 5 out]
        n651 = disable-structure shown="Enabled" {
          disable-tunnel: w1891 -> [w1947 w1951]
          disable-tunnel: [w1946 w1951] -> w1890
          frame Disabled {
            n652 = call <vilib>:"Play Sound File.vi"("error in (no error)"=w1947, "path"=path "C:/multiBot/patcherBot/sounds/FF7-Cast Magic.m4a") -> ("error out"=w1949:errorcluster)  [unwired: 8 in, 1 out]
            n653 = call "Time Delay45"("error in (no error)"=w1949, "Delay Time (s)"=0.2) -> ("error out"=w1946:errorcluster)  [unwired: 9 in]
          }
          frame Enabled {
          }
        }
        n654 = Unbundle By Name(w1927) -> ("misc common.mclamp cluster"=w1902:refnum<vi>)
        n655 = property class="DigNum (strict)"(reference=w1920) -> ("Value"=w1922:dbl)  [unwired: 1 in, 2 out]
        n656 = Unbundle By Name(w1921) -> ("gigaseal indiv"=w1893:T36, "gigaseal indiv.pipette resistance"=w1929:refnum<vi>, "gigaseal indiv.Iholding"=w1928:refnum<vi>, "gigaseal indiv.Ra"=w1910:refnum<vi>, "gigaseal indiv.Cm"=w1911:refnum<vi>)  [unwired: 8 out]
        n657 = call "prepBreakIn_toplvl.vi"("which manipulator"=w1912, "Slide Refnum"=w1913, "error in (no error)"=w1890, "Break In Pressure (mbar)"=w1922, "Pressure box control in"=w1926) -> ("error out"=w1924:errorcluster, "Pressure box control out"=w1925:T22)  [unwired: 5 in]
        n658 = property class="DigNum (strict)"(reference=w1923) -> (reference out=w1933:refnum<vi>, "Value"=w1906:i32)  [unwired: 1 in, 1 out]
        n659 = call "Time Delay18"("error in (no error)"=w1924, "Delay Time (s)"=0.5) -> ("error out"=w1940:errorcluster)  [unwired: 9 in]
        n660 = Index Array(array="Breakin durations (ms)", index=w1906) -> (element=w1942:i32)
        n661 = Array Size(array="Breakin num pulses") -> (size(s)=w1941:i32)
        n662 = Index Array(array="Breakin num pulses", index=w1906) -> (element=w1943:i32)
        n663 = Index Array(array="give a zap?", index=w1906) -> (element=w1905:i32)
        n664 = Equal?(x=w1905, y=1) -> (x = y?=w1903:bool)
        n665 = property class="Clust (strict)"(reference=w1902) -> ("Value"=w1901:T29)  [unwired: 1 in, 2 out]
        n666 = for {
          N: w1943 -> [_]
          tunnel: w1925 -> [w1981]
          tunnel: w1940 -> [w1983]
          tunnel: [w1982] -> w1898
          tunnel: w1942 -> [w1980]
          tunnel: w1912 -> [w1979]
          tunnel: w1903 -> [w1978]
          tunnel: w1901 -> [w1977]
          tunnel: w1900 -> [w1976]
          n667 = call "breakIn_toplvl_zapOption-v01.vi"("Pressure box control in"=w1981, "Multiclamp Handle In"=w1976, "which manipulator"=w1979, "break in duration (ms)"=w1980, "mclamp cluster"=w1977, "give a zap?"=w1978, "error in (no error)"=w1983) -> ("error out"=w1982:errorcluster)  [unwired: 7 in, 1 out]
        }
        n668 = property class="DigNum (strict)"(reference=w1899, error in=w1898) -> (error out=w1897:errorcluster, "Value"=w1895:i32)  [unwired: 1 out]
        n669 = Increment(x=w1906) -> (x+1=w1932:i32)
        n670 = Increment(x=w1895) -> (x+1=w1894:i32)
        n671 = property class="DigNum (strict)"(reference=w1899, error in=w1897, "Value"=w1894) -> (error out=w1896:errorcluster)  [unwired: 1 out]
        n672 = call "Time Delay17"("error in (no error)"=w1896, "Delay Time (s)"=3.0) -> ("error out"=w1892:errorcluster)  [unwired: 9 in]
        n673 = property class="DigNum (strict)" props=["Value"](reference=w1929, error in=w1892) -> (error out=w1909:errorcluster)  [unwired: 2 out]
        n674 = property on="Property Node" class="DigNum (strict)" props=["Value"](reference=w1911, error in=w1892) -> ()  [unwired: 3 out]
        n675 = property on="Property Node" class="DigNum (strict)" props=["Value"](reference=w1910, error in=w1892) -> ()  [unwired: 3 out]
        n676 = property on="Property Node" class="DigNum (strict)" props=["Value"](reference=w1928, error in=w1892) -> ()  [unwired: 3 out]
        n677 = call "detectWC_v0.006.vi"("gigaseal indiv"=w1893, "breakin attempt #"=w1906, "max breakin attempts #"=w1941, "error in (no error)"=w1909) -> ("error out"=w1908:errorcluster, "state out 2"=w1938:T3)  [unwired: 14 in]
        n678 = Not Equal?(x=user_message_v6."Breaking in...", y=w1938) -> (x != y?=w1936:bool)
        n679 = case shown="True" w1936 {
          tunnel: w1925 -> [w1953 w1957]
          tunnel: [w1953 w1957] -> w1915
          tunnel: w1908 -> [w1952 w1963]
          tunnel: [w1952 w1958] -> w1917
          tunnel: w1935 -> [_ w1961]
          tunnel: w1900 -> [_ w1960]
          tunnel: w1934 -> [_ w1959]
          tunnel: w1902 -> [_ w1955]
          tunnel: w1912 -> [_ w1954]
          frame False {
          }
          frame True {
            # "SELECT MCLAMP!"
            n680 = call "Time Delay19"("error in (no error)"=w1963, "Delay Time (s)"=1.0) -> ("error out"=w1956:errorcluster)  [unwired: 9 in]
            n681 = case shown="True" w1961 {
              tunnel: w1960 -> [_ w1971]
              tunnel: w1959 -> [_ w1975]
              tunnel: w1956 -> [w1964 w1966]
              tunnel: [w1964 w1973] -> w1958
              tunnel: w1955 -> [_ w1969]
              tunnel: w1954 -> [_ w1967]
              frame False {
              }
              frame True {
                # "apply holding voltage"
                n682 = property class="Clust (strict)"(reference=w1969, error in=w1966) -> (error out=w1965:errorcluster, "Value"=w1968:T29)  [unwired: 1 out]
                n683 = call "select_mclamp_channel.vi"("which manipulator"=w1967, "error in (no error)"=w1965, "mclamp cluster"=w1968, "Multiclamp Handle In"=w1971) -> ("error out"=w1972:errorcluster, "Multiclamp Handle out"=w1970:u32)  [unwired: 5 in, 1 out]
                n684 = dll-call lib="C:/multiBot/patcherBot/AxMultiClampMsg.dll" fn="MCCMSG_SetHoldingEnable"(error in=w1972, "handle"=w1970, "ModeConstant"=1, "error"=w1975) -> (error out=w1973:errorcluster)  [unwired: 6 in, 1 out]
              }
            }
          }
        }
        n685 = property class="DigNum (strict)"(reference=w1933, "Value"=w1932) -> ()  [unwired: 1 in, 2 out]
        n686 = call "prepBreakIn_toplvl.vi"("which manipulator"=w1912, "Slide Refnum"=w1913, "error in (no error)"=w1917, "Break In Pressure (mbar)"=w1918, "Pressure box control in"=w1915) -> ("error out"=w1916:errorcluster, "Pressure box control out"=w1914:T22)  [unwired: 5 in]
        n687 = call "setPressure_topLvl.vi"("which manipulator"=w1912, "Slide Refnum"=w1913, "error in"=w1916, "set pressure (mBar)"=w1918, "Pressure box control in"=w1914) -> ("error out"=w1919:errorcluster)  [unwired: 5 in, 1 out]
      }
      frame "Successful breakin!" {
        # "if other manip is in \"waiting for WC\"\n        Go to WC\nelse\n        Go to \"waiting for WC\""
        n688 = Unbundle By Name(w1992) -> ("misc indiv.other state ref"=w1991:refnum<vi>, "state UI indiv.successful breakin"=w1985:refnum<vi>)
        n689 = property class="Bool (strict)"(reference=w1985, "Value"=TRUE) -> ()  [unwired: 1 in, 2 out]
        n690 = Wait (ms)(milliseconds to wait=u32 5000) -> ()  [unwired: 1 out]
        n691 = property on="Property Node" class="Bool (strict)"(reference=w1987) -> ("Value"=w1986:bool)  [unwired: 1 in, 2 out]
        n692 = case shown="True" w1986 {
          tunnel: w1991 -> [_ w2007]
          tunnel: [user_message_v6."Whole-cell recording" ("state out") w2004] -> w1990
          tunnel: w1989 -> [_ w2003]
          tunnel: w1988 -> [_ w2001]
          frame False {
          }
          frame True {
            w2005 = user_message_v6."Waiting for WC" ("Value")
            # "if other pipette is in successful breakin or WC --> Go to WC too!"
            # "other state"
            n693 = call "wcLED_topLvl.vi"("which manipulator"=w2001, "wc LED"=TRUE, "Pressure box control in"=w2003) -> ()  [unwired: 7 in, 2 out]
            n694 = property on="Property Node" class="Enum (strict)"(reference=w2007) -> ("Value"=w1998:T3)  [unwired: 1 in, 2 out]
            n695 = Equal?(x=w1998, y=user_message_v6."Successful breakin!" ("Value")) -> (x = y?=w1997:bool)
            n696 = Equal?(x=w1998, y=w2005) -> (x = y?=w1999:bool)
            n697 = Or(x=w1999, y=w1997) -> (x .or. y?=w2000:bool)
            n698 = Select(t=user_message_v6."Whole-cell recording" ("Value"), s=w2000, f=w2005) -> (s? t:f=w2004:T3)
          }
        }
      }
      frame "Unsuccessful breakin!" {
        (unwired) user_message_v6."Saving autopatching parameters..." ("f")
        # "DO THIS IN NON-DEBUG MODE"
        # "DEBUG MODE! 7-3-17"
        # "some time to wallow"
        n699 = Wait (ms)(milliseconds to wait=u32 2000) -> ()  [unwired: 1 out]
      }
      frame "Whole-cell recording" {
        w2037 = T28 7 items=["Grayscale (U8)", "Grayscale (I16)", "Grayscale (SGL)", "Complex (CSG)", "RGB (U32)", "HSL (U32)", "RGB (U64)", "Grayscale (U16)"] ("Image Type")
        (unwired) user_message_v6."Saving autopatching parameters..." ("f")
        # "create image buffer"
        # "DO THIS IN NON-DEBUG MODE"
        # "DEBUG MODE! 7-3-17"
        # "STOP MEMTEST -> FALSE HERE"
        n700 = Unbundle By Name(w2027) -> ("misc common.stop memtest"=w2060:refnum<vi>, "misc common.dual patch cluster"=w2058:refnum<vi>, "misc common.mclamp cluster"=w2054:refnum<vi>, "misc common.dual WC keep going"=w2052:refnum<vi>, "misc common.HEK/slice options"=w2051:refnum<vi>, "ExperimentDescriptors.ExperimentVIToRun"=w2029:refnum<vi>, "PreviousValidationResults.ValidationResults"=w2025:refnum<vi>, "PreviousValidationResults.ValidationPos1"=w2024:refnum<vi>, "PreviousValidationResults.ValidationPos2"=w2023:refnum<vi>, "PreviousValidationResults.ValidationOutputCluster"=w2022:refnum<vi>, "misc common.Validate"=w2011:refnum<vi>)
        n701 = Unbundle By Name(w2026) -> ("misc indiv.Sampling Freq (Hz)"=w2046:refnum<vi>)
        n702 = Unbundle By Name(w2013) -> ("slice image"=w2012:T9)
        n703 = call "IMAQ Create"("Border Size"=0, "Image Name"="temp", "Image Type"=w2037, "error in (no error)"=w2035) -> ("New Image"=w2031:T9, "error out"=w2034:errorcluster)  [unwired: 1 in]
        n704 = Wait (ms)(milliseconds to wait=u32 500) -> ()  [unwired: 1 out]
        n705 = while {
          tunnel: w2012 -> [w2115]
          tunnel: w2041 -> [w2129]
          tunnel: w2042 -> [w2108]
          tunnel: [w2107] -> w2036
          tunnel: w2034 -> [w2114]
          tunnel: "images/06-beforeWholeCell.png" ("name or relative path") -> [w2126]
          tunnel: w2040 -> [w2124]
          tunnel: [w2106] -> w2033
          tunnel: [w2105] -> w2032
          tunnel: [w2103] -> w2030
          stop <- w2125 stop-if-true
          n706 = property class="Bool (strict)"(reference=w2124) -> ("Value"=w2123:bool)  [unwired: 1 in, 2 out]
          n707 = call "IMAQ GetImageSize"("Image"=w2115, "error in (no error)"=w2114) -> ("Y Resolution"=w2119:i32, "X Resolution"=w2122:i32, "error out"=w2113:errorcluster)  [unwired: 2 in]
          n708 = call "IMAQ ImageToArray"("error in (no error)"=w2113, "Image"=w2115) -> ("Image Pixels (U16)"=w2106:u16[][], "error out"=w2107:errorcluster)  [unwired: 2 in, 3 out]
          n709 = Add Array Elements(numeric array=w2106) -> (sum=w2112:u16)
          n710 = Build Path(base path=w2129, name or relative path=w2126) -> (appended path=w2105:path)
          n711 = Index Array(array=w2108) -> (element #1=w2121:i32, element #2=w2120:i32)  [unwired: 2 in]
          n712 = Equal?(x=w2119, y=w2120) -> (x = y?=w2117:bool)
          n713 = Greater?(x=w2112, y=u16 0) -> (0:w2109:bool)
          n714 = Equal?(x=w2122, y=w2121) -> (x = y?=w2118:bool)
          n715 = And(x=w2118, y=w2117) -> (x .and. y?=w2110:bool)
          n716 = Wait (ms)(milliseconds to wait=u32 1000) -> ()  [unwired: 1 out]
          n717 = And(x=w2110, y=w2109) -> (x .and. y?=w2104:bool)
          n718 = Select(t="Ready", s=w2104, f="Before") -> (s? t:f=w2103:string)
          n719 = Or(x=w2104, y=w2123) -> (x .or. y?=w2125:bool)
        }
        n720 = property class="Clust (strict)"(reference=w2054) -> ("Value"=w2053:T29)  [unwired: 1 in, 2 out]
        n721 = property class="Enum (strict)"(reference=w2051) -> (reference out=w2050:refnum<vi>, "Value"=w2049:enum16{"slice", "HEK"})  [unwired: 1 in, 1 out]
        n722 = Unbundle By Name(w2026) -> ("misc indiv.daq_ao"=w2068:tag, "misc indiv.daq_ai"=w2067:tag)
        n723 = property class="CmbBox"(reference=w2029) -> ("Value"=w2028:string)  [unwired: 1 in, 2 out]
        n724 = property class="Bool (strict)"(reference=w2056) -> ("Value"=w2057:bool)  [unwired: 1 in, 2 out]
        n725 = case shown="\"Ready\"" w2030 {
          tunnel: w2032 -> [_ w2099 _]
          tunnel: [FALSE TRUE FALSE] -> _
          tunnel: w2036 -> [w2088 w2092 w2101]
          tunnel: [w2088 w2090 w2101] -> w2018
          tunnel: w2033 -> [_ w2096 _]
          tunnel: w2031 -> [_ w2095 _]
          frame "Before", Default {
          }
          frame "Ready" {
            n726 = call "IMAQ ArrayToImage"("Image Pixels (U16)"=w2096, "error in (no error)"=w2092, "Image"=w2095) -> ("error out"=w2097:errorcluster, "Image Out"=w2093:T9)  [unwired: 7 in]
            n727 = call-poly "IMAQ Write File 2"("error in (no error)"=w2097, "Image Quality"=u32 1000, "File Path"=w2099, "Image"=w2093) -> ("error out"=w2091:errorcluster)  [unwired: 6 in, 1 out]
            n728 = call "IMAQ Dispose"("All Images? (No)"=FALSE, "Image"=w2093, "error in (no error)"=w2091) -> ("error out"=w2090:errorcluster)  [unwired: 3 in]
          }
          frame "After" {
          }
        }
        n729 = call <vilib>:"Play Sound File.vi"("error in (no error)"=w2018, "path"=path "C:/multiBot/patcherBot/sounds/LOZ-LTTP_Chest_Appears.wav") -> ("error out"=w2019:errorcluster)  [unwired: 8 in, 1 out]
        n730 = call "Time Delay5"("error in (no error)"=w2019, "Delay Time (s)"=0.2) -> ("error out"=w2017:errorcluster)  [unwired: 9 in]
        n731 = call "Time Delay10"("error in (no error)"=w2017, "Delay Time (s)"=0.5) -> ("error out"=w2044:errorcluster)  [unwired: 9 in]
        n732 = call "wcLED_topLvl.vi"("which manipulator"=w2059, "error in (no error)"=w2044, "wc LED"=TRUE, "Pressure box control in"=w2066) -> ("error out"=w2061:errorcluster, "Pressure box control out"=w2063:T22)  [unwired: 6 in]
        n733 = case shown="False" w2057 {
          tunnel: w2041 -> [w2161 w2372]
          tunnel: w2070 -> [w2172 w2371]
          tunnel: w2069 -> [w2171 w2370]
          tunnel: w2061 -> [w2170 w2373]
          tunnel: w2068 -> [_ _]
          tunnel: w2067 -> [_ _]
          tunnel: [w2164 w2391] -> w2064
          tunnel: w2060 -> [w2169 w2368]
          tunnel: w2059 -> [w2168 _]
          tunnel: w2058 -> [_ w2385]
          tunnel: w2055 -> [_ w2381]
          tunnel: w2053 -> [_ w2364]
          tunnel: w2052 -> [_ w2376]
          tunnel: w2050 -> [_ _]
          tunnel: w2049 -> [w2167 w2363]
          tunnel: w2048 -> [_ w2362]
          tunnel: w2012 -> [w2163 _]
          tunnel: w2046 -> [w2166 _]
          tunnel: w2042 -> [w2162 _]
          tunnel: w2040 -> [w2159 _]
          tunnel: w2028 -> [w2147 _]
          tunnel: w2027 -> [w2146 _]
          tunnel: w2026 -> [w2145 _]
          tunnel: w2013 -> [w2144 _]
          tunnel: w2025 -> [w2143 _]
          tunnel: w2024 -> [w2142 _]
          tunnel: w2023 -> [w2141 _]
          tunnel: w2022 -> [w2140 _]
          tunnel: [w2131 _] -> w2014
          tunnel: w2011 -> [w2130 _]
          frame False {
            w2156 = T28 7 items=["Grayscale (U8)", "Grayscale (I16)", "Grayscale (SGL)", "Complex (CSG)", "RGB (U32)", "HSL (U32)", "RGB (U64)", "Grayscale (U16)"] ("Image Type")
            # "create image buffer"
            n734 = case shown="\"pharmaBotExp\"" w2147 {
              tunnel: w2172 -> [_ w2212 w2241 w2286]
              tunnel: w2171 -> [_ w2211 w2240 w2285]
              tunnel: w2170 -> [w2173 w2198 w2243 w2288]
              tunnel: w2169 -> [_ w2196 w2244 w2289]
              tunnel: w2168 -> [_ w2192 w2230 w2275]
              tunnel: w2167 -> [_ w2185 w2236 w2281]
              tunnel: w2166 -> [_ w2181 w2239 w2284]
              tunnel: w2161 -> [_ w2175 w2242 w2287]
              tunnel: [w2173 w2174 w2245 w2290] -> w2149
              tunnel: w2146 -> [_ _ w2233 w2278]
              tunnel: w2145 -> [_ _ w2232 w2277]
              tunnel: w2144 -> [_ _ w2231 w2276]
              tunnel: w2143 -> [_ _ w2229 _]
              tunnel: w2142 -> [_ _ w2228 _]
              tunnel: w2141 -> [_ _ w2227 _]
              tunnel: w2140 -> [_ _ w2226 _]
              tunnel: [_ _ w2225 _] -> w2139
              tunnel: [_ _ w2224 _] -> w2138
              tunnel: [_ _ w2223 _] -> w2137
              tunnel: [_ _ w2222 _] -> w2136
              tunnel: [_ _ w2221 _] -> w2135
              tunnel: [_ _ w2220 _] -> w2134
              tunnel: [_ _ w2219 _] -> w2132
              tunnel: w2130 -> [_ _ w2218 _]
              frame "False", Default {
              }
              frame "autoWC" {
                # "restart memtest"
                # "stop memtest"
                n735 = case shown="\"manipulator 1\", Default" w2192 {
                  tunnel: [tag "Dev1/ao0" ("daq_ai 2") tag "Dev1/ao1" ("daq_ai 2")] -> w2191
                  tunnel: [tag "Dev1/ai0" ("daq_ai 2") tag "Dev1/ai1" ("daq_ai 2")] -> w2190
                  frame "manipulator 1", Default {
                  }
                  frame "manipulator 2" {
                  }
                }
                n736 = property class="Bool (strict)"(reference=w2196, error in=w2198, "Value"=TRUE) -> (reference out=w2195:refnum<vi>, error out=w2178:errorcluster)
                n737 = Wait (ms)(milliseconds to wait=u32 500) -> ()  [unwired: 1 out]
                n738 = call "Time Delay25"("error in (no error)"=w2178, "Delay Time (s)"=1.0) -> ("error out"=w2177:errorcluster)  [unwired: 9 in]
                n739 = Current VI's Path() -> (path=w2210:path)
                n740 = property class="DigNum (strict)"(reference=w2181) -> ("Value"=w2180:i32)  [unwired: 1 in, 2 out]
                n741 = Strip Path(path=w2210) -> (stripped path=w2189:path)  [unwired: 1 out]
                n742 = Strip Path(path=w2189) -> (stripped path=w2188:path)  [unwired: 1 out]
                n743 = Build Path(base path=w2188, name or relative path="whole_cell_protocol\\autoWC\\run_autoWC_v0.007.vi") -> (appended path=w2208:path)
                n744 = Open VI Reference(vi path=w2208, error in (no error)=w2177) -> (vi reference=w2207:refnum<vi>, error out=w2206:errorcluster)  [unwired: 4 in]
                n745 = Bundle By Name(cluster=T16 {"daq_ao 1"="Dev1/ao0", "daq_ai 1"="Dev1/ai0", "experiment day folder"=path "D:/DATA/8-27-15 save func testing/test.lvm", "Multiclamp init error"=0, "Multiclamp Handle Out"=0, "sampling rate (Hz)"=0, "trial name"=""} ("data in"), "daq_ao 1"=w2191, "daq_ai 1"=w2190, "experiment day folder"=w2175, "Multiclamp Handle Out"=w2212, "Multiclamp init error"=w2211, "sampling rate (Hz)"=w2180, "trial name"="t1") -> (w2183:T16)
                n746 = invoke class="VI" method="FP.Open"(reference=w2207, error in=w2206, "Activate"=TRUE ("Activate?"), "State"=T17."Standard") -> (reference out=w2200:refnum<vi>, error out=w2186:errorcluster)  [unwired: 1 in, 3 out]
                n747 = call "run_autoWC_v0.007.vi"("long?"="long wc protocol?", "error in"=w2186, "HEK/slice options"=w2185, "auto run?"=TRUE ("DEBUG?"), "data in"=w2183) -> ("error out"=w2187:errorcluster)  [unwired: 6 in]
                n748 = invoke class="VI" method="FP.Close"(reference=w2200, error in=w2187) -> (reference out=w2202:refnum<vi>, error out=w2201:errorcluster)  [unwired: 1 in, 1 out]
                n749 = Close Reference(reference=w2202, error in (no error)=w2201) -> (error out=w2193:errorcluster)
                n750 = property class="Bool (strict)"(reference=w2195, error in=w2193, "Value"=FALSE) -> (error out=w2174:errorcluster)  [unwired: 1 out]
              }
              frame "pharmaBotExp" {
                # "restart memtest"
                # "stop memtest"
                n751 = case shown="\"manipulator 1\", Default" w2230 {
                  tunnel: [tag "Dev1/ao0" ("daq_ai 2") tag "Dev1/ao1" ("daq_ai 2")] -> w2262
                  tunnel: [tag "Dev1/ai0" ("daq_ai 2") tag "Dev1/ai1" ("daq_ai 2")] -> w2263
                  frame "manipulator 1", Default {
                  }
                  frame "manipulator 2" {
                  }
                }
                n752 = property class="Bool (strict)"(reference=w2244, error in=w2243, "Value"=TRUE) -> (reference out=w2259:refnum<vi>, error out=w2268:errorcluster)
                n753 = Wait (ms)(milliseconds to wait=u32 500) -> ()  [unwired: 1 out]
                n754 = call "Time Delay38"("error in (no error)"=w2268, "Delay Time (s)"=1.0) -> ("error out"=w2269:errorcluster)  [unwired: 9 in]
                n755 = Current VI's Path() -> (path=w2246:path)
                n756 = property class="DigNum (strict)"(reference=w2239) -> ("Value"=w2266:i32)  [unwired: 1 in, 2 out]
                n757 = Strip Path(path=w2246) -> (stripped path=w2264:path)  [unwired: 1 out]
                n758 = property class="Bool (strict)"(reference=w2218) -> ("Value"=w2217:bool)  [unwired: 1 in, 2 out]
                n759 = Strip Path(path=w2264) -> (stripped path=w2265:path)  [unwired: 1 out]
                n760 = Build Path(base path=w2265, name or relative path="whole_cell_protocol\\autoWC\\run_pharmaBotExp_v0.015.vi") -> (appended path=w2248:path)
                n761 = Open VI Reference(vi path=w2248, error in (no error)=w2269) -> (vi reference=w2249:refnum<vi>, error out=w2250:errorcluster)  [unwired: 4 in]
                n762 = Bundle By Name(cluster=T16 {"daq_ao 1"="Dev1/ao0", "daq_ai 1"="Dev1/ai0", "experiment day folder"=path "D:/DATA/8-27-15 save func testing/test.lvm", "Multiclamp init error"=0, "Multiclamp Handle Out"=0, "sampling rate (Hz)"=0, "trial name"=""} ("data in"), "daq_ao 1"=w2262, "daq_ai 1"=w2263, "experiment day folder"=w2242, "Multiclamp Handle Out"=w2241, "Multiclamp init error"=w2240, "sampling rate (Hz)"=w2266, "trial name"="t1") -> (w2238:T16)
                n763 = invoke class="VI" method="FP.Open"(reference=w2249, error in=w2250, "Activate"=TRUE ("Activate?"), "State"=T17."Standard") -> (reference out=w2256:refnum<vi>, error out=w2235:errorcluster)  [unwired: 1 in, 3 out]
                n764 = call "run_pharmaBotExp_v0.015.vi"("data in"=w2238, "auto run?"=TRUE ("DEBUG?"), "which manipulator"=w2230, "HEK/slice options"=w2236, "error in"=w2235, "Validate after Experiment"=w2217, "common cluster"=w2233, "individual controls in"=w2232, "images"=w2231) -> ("Cell Looks Good?"=w2219:bool, "ValidationOutputCluster"=w2225:T1, "ValidationResults"=w2223:waveform(dbl)[][], "ValidationPos1"=w2222:T2, "Exp. Terminated"=w2220:bool, "ValidationPos2"=w2221:T2, "ValidationWaveform"=w2224:waveform(dbl)[], "error out"=w2234:errorcluster)  [unwired: 3 in]
                n765 = invoke class="VI" method="FP.Close"(reference=w2256, error in=w2234) -> (reference out=w2254:refnum<vi>, error out=w2255:errorcluster)  [unwired: 1 in, 1 out]
                n766 = property class="Arr (strict)"(reference=w2226, "Value"=w2225) -> ()  [unwired: 1 in, 2 out]
                n767 = Close Reference(reference=w2254, error in (no error)=w2255) -> (error out=w2261:errorcluster)
                n768 = property class="Arr (strict)"(reference=w2227, "Value"=w2221) -> ()  [unwired: 1 in, 2 out]
                n769 = property class="Arr (strict)"(reference=w2228, "Value"=w2222) -> ()  [unwired: 1 in, 2 out]
                n770 = property class="Arr (strict)"(reference=w2229, "Value"=w2223) -> ()  [unwired: 1 in, 2 out]
                n771 = property class="Bool (strict)"(reference=w2259, error in=w2261, "Value"=FALSE) -> (error out=w2245:errorcluster)  [unwired: 1 out]
              }
              frame "pharmaBotExpReliability" {
                # "restart memtest"
                # "stop memtest"
                n772 = case shown="\"manipulator 1\", Default" w2275 {
                  tunnel: [tag "Dev1/ao0" ("daq_ai 2") tag "Dev1/ao1" ("daq_ai 2")] -> w2307
                  tunnel: [tag "Dev1/ai0" ("daq_ai 2") tag "Dev1/ai1" ("daq_ai 2")] -> w2308
                  frame "manipulator 1", Default {
                  }
                  frame "manipulator 2" {
                  }
                }
                n773 = property class="Bool (strict)"(reference=w2289, error in=w2288, "Value"=TRUE) -> (reference out=w2304:refnum<vi>, error out=w2313:errorcluster)
                n774 = Wait (ms)(milliseconds to wait=u32 500) -> ()  [unwired: 1 out]
                n775 = call "Time Delay16"("error in (no error)"=w2313, "Delay Time (s)"=1.0) -> ("error out"=w2314:errorcluster)  [unwired: 9 in]
                n776 = Current VI's Path() -> (path=w2291:path)
                n777 = property class="DigNum (strict)"(reference=w2284) -> ("Value"=w2311:i32)  [unwired: 1 in, 2 out]
                n778 = Strip Path(path=w2291) -> (stripped path=w2309:path)  [unwired: 1 out]
                n779 = Strip Path(path=w2309) -> (stripped path=w2310:path)  [unwired: 1 out]
                n780 = Build Path(base path=w2310, name or relative path="whole_cell_protocol\\autoWC\\run_pharmaBotExpReliability_v0.002.vi") -> (appended path=w2293:path)
                n781 = Open VI Reference(vi path=w2293, error in (no error)=w2314) -> (vi reference=w2294:refnum<vi>, error out=w2295:errorcluster)  [unwired: 4 in]
                n782 = Bundle By Name(cluster=T16 {"daq_ao 1"="Dev1/ao0", "daq_ai 1"="Dev1/ai0", "experiment day folder"=path "D:/DATA/8-27-15 save func testing/test.lvm", "Multiclamp init error"=0, "Multiclamp Handle Out"=0, "sampling rate (Hz)"=0, "trial name"=""} ("data in"), "daq_ao 1"=w2307, "daq_ai 1"=w2308, "experiment day folder"=w2287, "Multiclamp Handle Out"=w2286, "Multiclamp init error"=w2285, "sampling rate (Hz)"=w2311, "trial name"="t1") -> (w2283:T16)
                n783 = invoke class="VI" method="FP.Open"(reference=w2294, error in=w2295, "Activate"=TRUE ("Activate?"), "State"=T17."Standard") -> (reference out=w2301:refnum<vi>, error out=w2280:errorcluster)  [unwired: 1 in, 3 out]
                n784 = call "run_pharmaBotExpReliability_v0.002.vi"("data in"=w2283, "auto run?"=TRUE ("DEBUG?"), "which manipulator"=w2275, "HEK/slice options"=w2281, "error in"=w2280, "common cluster"=w2278, "individual controls in"=w2277, "images"=w2276) -> ("error out"=w2279:errorcluster)  [unwired: 7 in]
                n785 = invoke class="VI" method="FP.Close"(reference=w2301, error in=w2279) -> (reference out=w2299:refnum<vi>, error out=w2300:errorcluster)  [unwired: 1 in, 1 out]
                n786 = Close Reference(reference=w2299, error in (no error)=w2300) -> (error out=w2306:errorcluster)
                n787 = property class="Bool (strict)"(reference=w2304, error in=w2306, "Value"=FALSE) -> (error out=w2290:errorcluster)  [unwired: 1 out]
              }
            }
            "ValidationResults" <- w2137
            "ValidationPos1" <- w2136
            "ValidationPos2" <- w2135
            "ValidationWaveform" <- w2138
            "ValidationOutputCluster" <- w2139
            n788 = Not(x=w2134) -> (.not. x?=w2133:bool)
            n789 = And(x=w2133, y=w2132) -> (x .and. y?=w2131:bool)
            n790 = call "IMAQ Create"("Border Size"=0, "Image Name"="temp", "Image Type"=w2156, "error in (no error)"=w2149) -> ("New Image"=w2151:T9, "error out"=w2150:errorcluster)  [unwired: 1 in]
            n791 = while {
              tunnel: w2163 -> [w2347]
              tunnel: w2161 -> [w2361]
              tunnel: w2162 -> [w2340]
              tunnel: [w2339] -> w2155
              tunnel: w2150 -> [w2346]
              tunnel: "images/07-afterWholeCell.png" ("name or relative path") -> [w2358]
              tunnel: w2159 -> [w2356]
              tunnel: [w2337] -> w2153
              tunnel: [w2336] -> w2152
              tunnel: [w2335] -> w2148
              stop <- w2357 stop-if-true
              n792 = property class="Bool (strict)"(reference=w2356) -> ("Value"=w2355:bool)  [unwired: 1 in, 2 out]
              n793 = call "IMAQ GetImageSize"("Image"=w2347, "error in (no error)"=w2346) -> ("Y Resolution"=w2351:i32, "X Resolution"=w2354:i32, "error out"=w2345:errorcluster)  [unwired: 2 in]
              n794 = call "IMAQ ImageToArray"("error in (no error)"=w2345, "Image"=w2347) -> ("Image Pixels (U16)"=w2337:u16[][], "error out"=w2339:errorcluster)  [unwired: 2 in, 3 out]
              n795 = Add Array Elements(numeric array=w2337) -> (sum=w2344:u16)
              n796 = Build Path(base path=w2361, name or relative path=w2358) -> (appended path=w2336:path)
              n797 = Index Array(array=w2340) -> (element #1=w2353:i32, element #2=w2352:i32)  [unwired: 2 in]
              n798 = Equal?(x=w2351, y=w2352) -> (x = y?=w2349:bool)
              n799 = Greater?(x=w2344, y=u16 0) -> (0:w2341:bool)
              n800 = Equal?(x=w2354, y=w2353) -> (x = y?=w2350:bool)
              n801 = And(x=w2350, y=w2349) -> (x .and. y?=w2342:bool)
              n802 = Wait (ms)(milliseconds to wait=u32 1000) -> ()  [unwired: 1 out]
              n803 = And(x=w2342, y=w2341) -> (x .and. y?=w2338:bool)
              n804 = Select(t="Ready", s=w2338, f="Before") -> (s? t:f=w2335:string)
              n805 = Or(x=w2338, y=w2355) -> (x .or. y?=w2357:bool)
            }
            n806 = case shown="\"Ready\"" w2148 {
              tunnel: w2152 -> [_ w2331 _]
              tunnel: [FALSE TRUE FALSE] -> _
              tunnel: w2155 -> [w2320 w2324 w2333]
              tunnel: [w2320 w2322 w2333] -> w2154
              tunnel: w2153 -> [_ w2328 _]
              tunnel: w2151 -> [_ w2327 _]
              frame "Before", Default {
              }
              frame "Ready" {
                n807 = call "IMAQ ArrayToImage"("Image Pixels (U16)"=w2328, "error in (no error)"=w2324, "Image"=w2327) -> ("error out"=w2329:errorcluster, "Image Out"=w2325:T9)  [unwired: 7 in]
                n808 = call-poly "IMAQ Write File 2"("error in (no error)"=w2329, "Image Quality"=u32 1000, "File Path"=w2331, "Image"=w2325) -> ("error out"=w2323:errorcluster)  [unwired: 6 in, 1 out]
                n809 = call "IMAQ Dispose"("All Images? (No)"=FALSE, "Image"=w2325, "error in (no error)"=w2323) -> ("error out"=w2322:errorcluster)  [unwired: 3 in]
              }
              frame "After" {
              }
            }
            n810 = call "Time Delay9"("error in (no error)"=w2154, "Delay Time (s)"=0.5) -> ("error out"=w2164:errorcluster)  [unwired: 9 in]
          }
          frame True {
            w2369 = T37 [enum."manipulator 1", enum."manipulator 2"] items=["manipulator 1", "manipulator 2", "manipulator 3", "manipulator 4"]
            # "dual WC"
            # "stop memtest"
            # "both channels to vclamp"
            # "both channels to iclamp"
            # "restart memtest"
            # "stop memtest"
            n811 = property class="Bool (strict)"(reference=w2368, error in=w2373, "Value"=TRUE) -> (reference out=w2366:refnum<vi>, error out=w2374:errorcluster)
            n812 = for {
              tunnel: w2372 -> [w2410]
              tunnel: w2371 -> [w2417]
              tunnel: w2370 -> [w2419]
              shift-right: [w2423] -> w2367
              shift-left: w2374 -> [w2415]
              tunnel: w2369 -> [w2413] mode=indexing
              tunnel: w2364 -> [w2416]
              tunnel: w2363 -> [w2405]
              tunnel: w2362 -> [w2403]
              # "individual WC"
              n813 = case shown="\"manipulator 1\", Default" w2413 {
                tunnel: [tag "Dev1/ao0" ("daq_ai 2") tag "Dev1/ao1" ("daq_ai 2")] -> w2422
                tunnel: [tag "Dev1/ai0" ("daq_ai 2") tag "Dev1/ai1" ("daq_ai 2")] -> w2421
                tunnel: ["m1" "m2"] -> w2411
                frame "manipulator 1", Default {
                }
                frame "manipulator 2" {
                }
              }
              n814 = call "select_mclamp_channel.vi"("which manipulator"=w2413, "error in (no error)"=w2415, "mclamp cluster"=w2416, "Multiclamp Handle In"=w2417) -> ("error out"=w2414:errorcluster, "Multiclamp Handle out"=w2412:u32)  [unwired: 5 in, 1 out]
              n815 = Current VI's Path() -> (path=w2435:path)
              n816 = Strip Path(path=w2435) -> (stripped path=w2418:path)  [unwired: 1 out]
              n817 = Build Path(base path=w2410, name or relative path=w2411) -> (appended path=w2409:path)
              n818 = Strip Path(path=w2418) -> (stripped path=w2420:path)  [unwired: 1 out]
              n819 = property class="DigNum (strict)"(reference=w2403) -> ("Value"=w2402:i32)  [unwired: 1 in, 2 out]
              n820 = Build Path(base path=w2420, name or relative path="whole_cell_protocol\\autoWC\\run_autoWC_v0.006.vi") -> (appended path=w2433:path)
              n821 = Bundle By Name(cluster=T16 {"daq_ao 1"="Dev1/ao0", "daq_ai 1"="Dev1/ai0", "experiment day folder"=path "D:/DATA/8-27-15 save func testing/test.lvm", "Multiclamp init error"=0, "Multiclamp Handle Out"=0, "sampling rate (Hz)"=0, "trial name"=""} ("data in"), "daq_ao 1"=w2422, "daq_ai 1"=w2421, "experiment day folder"=w2409, "Multiclamp Handle Out"=w2412, "Multiclamp init error"=w2419, "sampling rate (Hz)"=w2402, "trial name"="t1") -> (w2407:T16)
              n822 = Open VI Reference(vi path=w2433, error in (no error)=w2414) -> (vi reference=w2432:refnum<vi>, error out=w2431:errorcluster)  [unwired: 4 in]
              n823 = invoke class="VI" method="FP.Open"(reference=w2432, error in=w2431, "Activate"=TRUE ("Activate?"), "State"=T17."Standard") -> (reference out=w2425:refnum<vi>, error out=w2404:errorcluster)  [unwired: 1 in, 3 out]
              n824 = call "run_autoWC_v0.007.vi"("error in"=w2404, "HEK/slice options"=w2405, "auto run?"=TRUE ("DEBUG?"), "data in"=w2407) -> ("error out"=w2408:errorcluster)  [unwired: 7 in]
              n825 = invoke class="VI" method="FP.Close"(reference=w2425, error in=w2408) -> (reference out=w2427:refnum<vi>, error out=w2426:errorcluster)  [unwired: 1 in, 1 out]
              n826 = Close Reference(reference=w2427, error in (no error)=w2426) -> (error out=w2423:errorcluster)
            }
            n827 = case shown="True" w2381 {
              tunnel: w2367 -> [w2467 w2480]
              tunnel: [w2467 w2468] -> w2365
              tunnel: w2371 -> [_ w2479]
              tunnel: w2364 -> [_ w2477]
              frame False {
              }
              frame True {
                w2473 = enum16{"VClamp", "IClamp"}."IClamp" ("which clamp")
                n828 = call "select_mclamp_channel.vi"("which manipulator"=T5."manipulator 1", "error in (no error)"=w2480, "mclamp cluster"=w2477, "Multiclamp Handle In"=w2479) -> ("error out"=w2471:errorcluster, "error"=w2478:i32, "Multiclamp Handle out"=w2476:u32)  [unwired: 5 in]
                n829 = call "multiclamp_switchClamps_v02.vi"("error in"=w2478, "error in (no error)"=w2471, "which clamp"=w2473, "Multiclamp Handle in"=w2476) -> ("error out"=w2470:errorcluster)  [unwired: 6 in, 1 out]
                n830 = call "select_mclamp_channel.vi"("which manipulator"=T5."manipulator 2", "error in (no error)"=w2470, "mclamp cluster"=w2477, "Multiclamp Handle In"=w2476) -> ("error out"=w2469:errorcluster, "error"=w2472:i32, "Multiclamp Handle out"=w2474:u32)  [unwired: 5 in]
                n831 = call "multiclamp_switchClamps_v02.vi"("error in"=w2472, "error in (no error)"=w2469, "which clamp"=w2473, "Multiclamp Handle in"=w2474) -> ("error out"=w2468:errorcluster)  [unwired: 6 in, 1 out]
              }
            }
            n832 = Current VI's Path() -> (path=w2395:path)
            n833 = call "Time Delay20"("error in (no error)"=w2365, "Delay Time (s)"=1.0) -> ("error out"=w2378:errorcluster)  [unwired: 9 in]
            n834 = Strip Path(path=w2395) -> (stripped path=w2383:path)  [unwired: 1 out]
            n835 = Strip Path(path=w2383) -> (stripped path=w2393:path)  [unwired: 1 out]
            n836 = Build Path(base path=w2393, name or relative path="memtest_VIs\\dual_patch\\test_dualPatch.vi") -> (appended path=w2399:path)
            n837 = property class="Clust (strict)"(reference=w2385) -> ("Value"=w2384:T38)  [unwired: 1 in, 2 out]
            n838 = Open VI Reference(vi path=w2399, error in (no error)=w2378) -> (vi reference=w2398:refnum<vi>, error out=w2397:errorcluster)  [unwired: 4 in]
            n839 = invoke class="VI" method="FP.Open"(reference=w2398, error in=w2397, "Activate"=TRUE ("Activate?"), "State"=T17."Standard") -> (reference out=w2386:refnum<vi>, error out=w2387:errorcluster)  [unwired: 1 in, 3 out]
            n840 = while {
              tunnel: "AO physical channels" -> [w2449]
              tunnel: "AI Physical Channel" -> [w2448]
              tunnel: w2387 -> [w2444]
              tunnel: [w2450] -> w2382
              tunnel: w2384 -> [w2445]
              tunnel: w2372 -> [w2447]
              tunnel: w2376 -> [w2443]
              stop <- w2442 continue-if-true
              n841 = property class="Bool (strict)"(reference=w2443, error in=w2444) -> ("Value"=w2442:bool)  [unwired: 2 out]
              n842 = call "test_dualPatch_v02.vi"("experiment day folder"=w2447, "dual patch cluster"=w2445, "AO error in"=w2444, "AI Physical Channel"=w2448, "AO physical channels"=w2449) -> ("error out"=w2446:errorcluster)  [unwired: 6 in]
              n843 = call "Time Delay"("error in (no error)"=w2446, "Delay Time (s)"=20.0) -> ("error out"=w2450:errorcluster)  [unwired: 9 in]
            }
            n844 = case shown="True" w2381 {
              tunnel: w2382 -> [w2452 w2465]
              tunnel: [w2452 w2453] -> w2380
              tunnel: w2364 -> [_ w2463]
              tunnel: w2371 -> [_ w2457]
              frame False {
              }
              frame True {
                w2459 = enum16{"VClamp", "IClamp"}."VClamp" ("which clamp")
                n845 = call "select_mclamp_channel.vi"("which manipulator"=T5."manipulator 1", "error in (no error)"=w2465, "mclamp cluster"=w2463, "Multiclamp Handle In"=w2457) -> ("error out"=w2456:errorcluster, "error"=w2464:i32, "Multiclamp Handle out"=w2462:u32)  [unwired: 5 in]
                n846 = call "multiclamp_switchClamps_v02.vi"("error in"=w2464, "error in (no error)"=w2456, "which clamp"=w2459, "Multiclamp Handle in"=w2462) -> ("error out"=w2455:errorcluster)  [unwired: 6 in, 1 out]
                n847 = call "select_mclamp_channel.vi"("which manipulator"=T5."manipulator 2", "error in (no error)"=w2455, "mclamp cluster"=w2463, "Multiclamp Handle In"=w2462) -> ("error out"=w2454:errorcluster, "error"=w2458:i32, "Multiclamp Handle out"=w2460:u32)  [unwired: 5 in]
                n848 = call "multiclamp_switchClamps_v02.vi"("error in"=w2458, "error in (no error)"=w2454, "which clamp"=w2459, "Multiclamp Handle in"=w2460) -> ("error out"=w2453:errorcluster)  [unwired: 6 in, 1 out]
              }
            }
            n849 = invoke class="VI" method="FP.Close"(reference=w2386, error in=w2380) -> (reference out=w2390:refnum<vi>, error out=w2389:errorcluster)  [unwired: 1 in, 1 out]
            n850 = Close Reference(reference=w2390, error in (no error)=w2389) -> (error out=w2388:errorcluster)
            n851 = property class="Bool (strict)"(reference=w2366, error in=w2388, "Value"=FALSE) -> (error out=w2391:errorcluster)  [unwired: 1 out]
          }
        }
        n852 = disable-structure shown="Enabled" {
          disable-tunnel: w2064 -> [w2085 w2087]
          disable-tunnel: w2063 -> [w2084 _]
          disable-tunnel: w2059 -> [w2083 _]
          disable-tunnel: [w2082 w2087] -> w2016
          frame Disabled {
            n853 = call "wcLED_topLvl.vi"("which manipulator"=w2083, "error in (no error)"=w2085, "wc LED"=FALSE, "Pressure box control in"=w2084) -> ("error out"=w2082:errorcluster)  [unwired: 6 in, 1 out]
          }
          frame Enabled {
          }
        }
        n854 = case shown="True" w2014 {
          tunnel: w2016 -> [w2073 w2078]
          tunnel: [w2072 w2077] -> w2015
          frame True {
            n855 = call <vilib>:"Play Sound File.vi"("error in (no error)"=w2073, "path"=path "C:/multiBot/patcherBot/sounds/LTTP_ItemFanfare.wav") -> ("error out"=w2074:errorcluster)  [unwired: 8 in, 1 out]
            n856 = call "Time Delay6"("error in (no error)"=w2074, "Delay Time (s)"=0.2) -> ("error out"=w2072:errorcluster)  [unwired: 9 in]
          }
          frame False {
            n857 = call <vilib>:"Play Sound File.vi"("error in (no error)"=w2078, "path"=path "C:/multiBot/patcherBot/sounds/wlk-oi.wav") -> ("error out"=w2079:errorcluster)  [unwired: 8 in, 1 out]
            n858 = call "Time Delay46"("error in (no error)"=w2079, "Delay Time (s)"=0.2) -> ("error out"=w2077:errorcluster)  [unwired: 9 in]
          }
        }
      }
      frame "Saving autopatching parameters..." {
        w2493 = T28 7 items=["Grayscale (U8)", "Grayscale (I16)", "Grayscale (SGL)", "Complex (CSG)", "RGB (U32)", "HSL (U32)", "RGB (U64)", "Grayscale (U16)"] ("Image Type")
        # "create image buffer"
        # "7/1/17 disabled this for debugging purposes"
        # "used to be connected to exit trigger"
        # "SELECT NEXT CELL HERE"
        # "if this is the last cell, stop program"
        # "add final time, that is time of the last operation whatever it was"
        n859 = Unbundle By Name(w2540) -> ("positioning+hunting common.cells (image px)"=w2539:refnum<vi>, "positioning+hunting common.current cell locations (px)"=w2521:refnum<vi>, "positioning+hunting common.unpatched cell indices"=w2519:refnum<vi>, "cell tracker common.cell centroid array"=w2518:refnum<vi>, "cell tracker common.pipette centroid array"=w2517:refnum<vi>, "misc common.Select cells based on proximity (multi patch)"=w2507:refnum<vi>)
        n860 = property class="Arr (strict)"(reference=w2546) -> ("Value"=w2545:dbl[])  [unwired: 1 in, 2 out]
        n861 = Unbundle By Name(w2483) -> ("slice image"=w2482:T9)
        n862 = property class="Arr (strict)"(reference=w2544) -> ("Value"=w2542:dbl[])  [unwired: 1 in, 2 out]
        n863 = property class="Arr (strict)"(reference=w2543) -> ("Value"=w2541:dbl[])  [unwired: 1 in, 2 out]
        n864 = property class="Arr (strict)"(reference=w2548) -> ("Value"=w2547:i32[])  [unwired: 1 in, 2 out]
        n865 = Unbundle By Name(w2531) -> ("positioning + hunting indiv.current cell"=w2524:refnum<vi>, "misc indiv.trial data saved"=w2530:refnum<vi>, "misc indiv.state list"=w2528:refnum<vi>, "misc indiv.state times"=w2526:refnum<vi>)
        n866 = Wait (ms)(milliseconds to wait=u32 500) -> ()  [unwired: 1 out]
        n867 = property class="Arr (strict)"(reference=w2539) -> ("Value"=w2538:dbl[][])  [unwired: 1 in, 2 out]
        n868 = property class="Arr (strict)"(reference=w2526) -> (reference out=w2525:refnum<vi>, "Value"=w2505:dbl[])  [unwired: 1 in, 1 out]
        n869 = property class="Bool (strict)"(reference=w2530, "Value"=TRUE ("data saved?")) -> ()  [unwired: 1 in, 2 out]
        n870 = property class="Arr (strict)"(reference=w2528) -> ("Value"=w2527:string[])  [unwired: 1 in, 2 out]
        n871 = property class="Arr (strict)"(reference=w2518) -> ("Value"=w2514:dbl[][])  [unwired: 1 in, 2 out]
        n872 = property class="Arr (strict)"(reference=w2517) -> ("Value"=w2510:dbl[][])  [unwired: 1 in, 2 out]
        n873 = Build Path(base path=w2484, name or relative path="cell_location_px.lvm") -> (appended path=w2551:path)
        n874 = call "Convert to Dynamic Data2"("Array"=w2545) -> ("Dynamic Data Type"=w2575:dynamicdata)  [unwired: 3 in]
        n875 = call "Convert to Dynamic Data"("Array"=w2542) -> ("Dynamic Data Type"=w2574:dynamicdata)  [unwired: 3 in]
        n876 = Build Path(base path=w2484, name or relative path="state_list.txt") -> (appended path=w2564:path)
        n877 = Build Path(base path=w2484, name or relative path="NH.lvm") -> (appended path=w2569:path)
        n878 = Build Path(base path=w2484, name or relative path="cell_centroid_array.lvm") -> (appended path=w2516:path)
        n879 = Merge Signals(w2575, w2574) -> (w2576:dynamicdata)
        n880 = Build Path(base path=w2484, name or relative path="pipette_centroid_array.lvm") -> (appended path=w2511:path)
        n881 = Open/Create/Replace File(file path (use dialog)=w2564, operation (0:open)=T18."replace or create", access (0:read/write)=enum16{"read/write", "read-only", "write-only"}."read/write") -> (refnum out=w2560:refnum<file>, error out=w2561:errorcluster)  [unwired: 3 in, 1 out]
        n882 = Build Path(base path=w2484, name or relative path="GS.lvm") -> (appended path=w2567:path)
        n883 = Build Path(base path=w2484, name or relative path="state_times.lvm") -> (appended path=w2553:path)
        n884 = Write to Text File(file (use dialog)=w2560, text=w2527, error in=w2561) -> (refnum out=w2558:refnum<file>, error out=w2559:errorcluster)  [unwired: 1 in, 1 out]
        n885 = call "Convert to Dynamic Data7"("2D Array"=w2514) -> ("Dynamic Data Type"=w2513:dynamicdata)  [unwired: 3 in]
        n886 = call "Convert to Dynamic Data8"("2D Array"=w2510) -> ("Dynamic Data Type"=w2509:dynamicdata)  [unwired: 3 in]
        n887 = call "Convert to Dynamic Data4"("Array"=w2547) -> ("Dynamic Data Type"=w2571:dynamicdata)  [unwired: 3 in]
        n888 = call "Convert to Dynamic Data3"("Array"=w2541) -> ("Dynamic Data Type"=w2572:dynamicdata)  [unwired: 3 in]
        n889 = Close File(refnum=w2558, error in=w2559) -> (error out=w2502:errorcluster)  [unwired: 1 out]
        n890 = call "save NH"("Signals"=w2576, "error in (no error)"=w2502, "Filename"=w2569) -> ("error out"=w2555:errorcluster)  [unwired: 14 in, 2 out]
        n891 = call "save cell centroid"("Signals"=w2513, "Filename"=w2516) -> ()  [unwired: 15 in, 3 out]
        n892 = call "save pipette centroid"("Signals"=w2509, "Filename"=w2511) -> ()  [unwired: 15 in, 3 out]
        n893 = Merge Signals(w2571, w2572) -> (w2573:dynamicdata)
        n894 = property class="Arr (strict)"(reference=w2525, "Value"=w2505) -> ()  [unwired: 1 in, 2 out]
        n895 = call "save GS"("Signals"=w2573, "error in (no error)"=w2555, "Filename"=w2567) -> ("error out"=w2554:errorcluster)  [unwired: 14 in, 2 out]
        n896 = call "Convert to Dynamic Data5"("Array"=w2505) -> ("Dynamic Data Type"=w2566:dynamicdata)  [unwired: 3 in]
        n897 = call "save state times"("Signals"=w2566, "error in (no error)"=w2554, "Filename"=w2553) -> ("error out"=w2537:errorcluster)  [unwired: 14 in, 2 out]
        n898 = property class="Bool (strict)"(reference=w2507) -> ("Value"=w2506:bool)  [unwired: 1 in, 2 out]
        n899 = property class="DigNum (strict)"(reference=w2524, error in=w2537) -> (reference out=w2534:refnum<vi>, error out=w2536:errorcluster, "Value"=w2535:i32)
        n900 = Index Array(array=w2538, index (col)=w2535) -> (element=w2550:dbl[])  [unwired: 1 in]
        n901 = case shown="True" w2506 {
          tunnel: w2538 -> [w2628 _]
          tunnel: w2535 -> [w2627 _]
          tunnel: [w2626 w2635] -> w2533
          tunnel: [w2625 w2632] -> w2532
          tunnel: w2523 -> [_ w2639]
          tunnel: w2522 -> [_ w2638]
          tunnel: w2521 -> [_ w2637]
          tunnel: w2520 -> [_ w2634]
          tunnel: w2519 -> [_ w2633]
          frame False {
            n902 = Array Size(array=w2628) -> (size(s)=w2631:i32[])
            n903 = Increment(x=w2627) -> (x+1=w2626:i32)
            n904 = Index Array(array=w2631, index=1) -> (element=w2630:i32)
            n905 = Equal?(x=w2626, y=w2630) -> (x = y?=w2625:bool)
          }
          frame True {
            n906 = property class="Arr (strict)"(reference=w2637) -> ("Value"=w2636:dbl[][])  [unwired: 1 in, 2 out]
            n907 = call "get_nextCellIndex.vi"("which manipulator"=w2634, "unpatched cell indices ref"=w2633, "transform cluster"=w2638, "positions cluster"=w2639, "current cell locations (px)"=w2636) -> ("out of cells to patch"=w2632:bool, "next manip cell"=w2635:i32)  [unwired: 4 in, 1 out]
          }
        }
        n908 = call "Convert to Dynamic Data6"("Array"=w2550) -> ("Dynamic Data Type"=w2549:dynamicdata)  [unwired: 3 in]
        n909 = call "save cell array"("Signals"=w2549, "error in (no error)"=w2536, "Filename"=w2551) -> ("error out"=w2501:errorcluster)  [unwired: 14 in, 2 out]
        n910 = call "Time Delay3"("error in (no error)"=w2501, "Delay Time (s)"=0.2) -> ("error out"=w2487:errorcluster)  [unwired: 9 in]
        n911 = call "IMAQ Create"("Border Size"=0, "Image Name"="temp", "Image Type"=w2493, "error in (no error)"=w2487) -> ("New Image"=w2488:T9, "error out"=w2486:errorcluster)  [unwired: 1 in]
        n912 = while {
          tunnel: w2482 -> [w2605]
          tunnel: w2484 -> [w2619]
          tunnel: w2498 -> [w2598]
          tunnel: [w2596] -> w2492
          tunnel: w2486 -> [w2604]
          tunnel: "images/09-final.png" ("name or relative path") -> [w2616]
          tunnel: w2496 -> [w2614]
          tunnel: [w2597] -> w2490
          tunnel: [w2594] -> w2489
          tunnel: [w2593] -> w2485
          stop <- w2615 stop-if-true
          n913 = property class="Bool (strict)"(reference=w2614) -> ("Value"=w2613:bool)  [unwired: 1 in, 2 out]
          n914 = call "IMAQ GetImageSize"("Image"=w2605, "error in (no error)"=w2604) -> ("Y Resolution"=w2609:i32, "X Resolution"=w2612:i32, "error out"=w2603:errorcluster)  [unwired: 2 in]
          n915 = call "IMAQ ImageToArray"("error in (no error)"=w2603, "Image"=w2605) -> ("Image Pixels (U16)"=w2594:u16[][], "error out"=w2596:errorcluster)  [unwired: 2 in, 3 out]
          n916 = Add Array Elements(numeric array=w2594) -> (sum=w2602:u16)
          n917 = Build Path(base path=w2619, name or relative path=w2616) -> (appended path=w2597:path)
          n918 = Index Array(array=w2598) -> (element #1=w2611:i32, element #2=w2610:i32)  [unwired: 2 in]
          n919 = Equal?(x=w2609, y=w2610) -> (x = y?=w2607:bool)
          n920 = Greater?(x=w2602, y=u16 0) -> (0:w2599:bool)
          n921 = Equal?(x=w2612, y=w2611) -> (x = y?=w2608:bool)
          n922 = And(x=w2608, y=w2607) -> (x .and. y?=w2600:bool)
          n923 = Wait (ms)(milliseconds to wait=u32 1000) -> ()  [unwired: 1 out]
          n924 = And(x=w2600, y=w2599) -> (x .and. y?=w2595:bool)
          n925 = Select(t="Ready", s=w2595, f="Before") -> (s? t:f=w2593:string)
          n926 = Or(x=w2595, y=w2613) -> (x .or. y?=w2615:bool)
        }
        n927 = property class="DigNum (strict)"(reference=w2534, "Value"=w2533) -> ()  [unwired: 1 in, 2 out]
        n928 = case shown="\"Ready\"" w2485 {
          tunnel: w2490 -> [_ w2589 _]
          tunnel: [FALSE TRUE FALSE] -> _
          tunnel: w2492 -> [w2578 w2582 w2591]
          tunnel: [w2578 w2580 w2591] -> w2491
          tunnel: w2489 -> [_ w2586 _]
          tunnel: w2488 -> [_ w2585 _]
          frame "Before", Default {
          }
          frame "Ready" {
            n929 = call "IMAQ ArrayToImage"("Image Pixels (U16)"=w2586, "error in (no error)"=w2582, "Image"=w2585) -> ("error out"=w2587:errorcluster, "Image Out"=w2583:T9)  [unwired: 7 in]
            n930 = call-poly "IMAQ Write File 2"("error in (no error)"=w2587, "Image Quality"=u32 1000, "File Path"=w2589, "Image"=w2583) -> ("error out"=w2581:errorcluster)  [unwired: 6 in, 1 out]
            n931 = call "IMAQ Dispose"("All Images? (No)"=FALSE, "Image"=w2583, "error in (no error)"=w2581) -> ("error out"=w2580:errorcluster)  [unwired: 3 in]
          }
          frame "After" {
          }
        }
        n932 = call "Time Delay30"("error in (no error)"=w2491, "Delay Time (s)"=0.2) -> ("error out"=w2499:errorcluster)  [unwired: 9 in]
        n933 = disable-structure shown="Enabled" {
          disable-tunnel: [w2621 user_message_v6."DEBUG STATE" ("t")] -> w2556
          disable-tunnel: w2532 -> [w2620 _]
          disable-tunnel: [w2620 _] -> w2508
          frame Enabled {
            n934 = Select(t=user_message_v6."Done with Current Set of Cells", s=w2620, f=user_message_v6."Cleaning..." ("t")) -> (s? t:f=w2621:T3)
          }
          frame Disabled {
          }
        }
      }
      frame "Quitting VI" {
        w2642 = FALSE ("approach? (T = on)")
        # "reset stage to fast movement"
        n935 = call "reset manipulator.vi"("error in"=w2643, "approach? (T = on)"=w2642, "motion"=scope_motion."slow_dualPatch", "manip in"=w2644) -> ()  [unwired: 6 in, 2 out]
        n936 = call "reset manipulator.vi"("error in"=w2653, "approach? (T = on)"=w2642, "motion"=scope_motion."fast", "manip in"=w2649) -> ()  [unwired: 6 in, 2 out]
        n937 = call "switchPressure_topLvl.vi"("which manipulator"=w2645, "Slide Refnum"=w2648, "error in"=w2651, "pressure setting"=arduino_pressure_setting."Low Positive Pressure" ("arduino pressure setting"), "Pressure box control in"=w2652) -> ("error out"=w2650:errorcluster)  [unwired: 5 in, 1 out]
        n938 = Wait (ms)(milliseconds to wait=u32 2000) -> ()  [unwired: 1 out]
      }
      frame "Waiting for idle stage..." {
        n939 = Unbundle By Name(w2662) -> ("misc common.stage idle?"=w2663:refnum<vi>)
        n940 = property on="Property Node" class="Bool (strict)"(reference=w2663) -> ("Value"=w2661:bool)  [unwired: 1 in, 2 out]
        n941 = Select(t=user_message_v6."Starting new attempt..." ("Message to user"), s=w2661, f=user_message_v6."Waiting for idle stage..." ("Message to user")) -> (s? t:f=w2660:T3)
        n942 = Wait (ms)(milliseconds to wait=u32 100) -> ()  [unwired: 1 out]
        n943 = Wait (ms)(milliseconds to wait=u32 100) -> ()  [unwired: 1 out]
      }
      frame "Cleaning..." {
        w2699 = TRUE ("blocking?")
        # "go back to safe location"
        # "if this is the last cell in the list, quit"
        n944 = Unbundle By Name(w2750) -> ("Actuator COM"=w2751:refnum<visa-resource-name>)
        n945 = Unbundle By Name(w2745) -> ("state UI indiv.demo clean"=w2769:refnum<vi>, "cleaning indiv.avg peak height"=w2768:refnum<vi>, "cleaning indiv.cleaning status"=w2767:refnum<vi>, "cleaning indiv.clean bath detected"=w2758:refnum<vi>, "cleaning indiv.wash bath detected"=w2757:refnum<vi>)
        n946 = Unbundle By Name(w2766) -> ("misc common.mclamp cluster"=w2765:refnum<vi>)
        n947 = call "sc_adjustMotion.vi"("error in (no error)"=w2753, "motion"=scope_motion."fast", "VISA handle"=w2751) -> ("error out"=w2752:errorcluster)  [unwired: 7 in, 1 out]
        n948 = flat-sequence {
          tunnel: [w2863] -> w2710
          tunnel: [w2864] -> w2709
          tunnel: [w2866] -> w2703
          tunnel: [w2865] -> w2700
          tunnel: w2750 -> [w2863]
          tunnel: w2752 -> [w2864]
          tunnel: w2773 -> [w2862]
          tunnel: [w2862] -> w2711
          tunnel: [w2861] -> w2687
          tunnel: w2771 -> [w2861]
          tunnel: [w2855] -> w2685
          tunnel: w2745 -> [w2860]
          tunnel: [w2854] -> w2674
          frame #0 {
            # "REPLACE ALL"
            # "calculate positions (x_wash, y_wash, z_above)"
            n949 = Unbundle By Name(w2860) -> ("cleaning indiv.loc above baths"=w2858:refnum<vi>, "cleaning indiv.wash bath loc"=w2857:refnum<vi>, "cleaning indiv.cleaning bath loc"=w2856:refnum<vi>)
            n950 = property class="Arr (strict)"(reference=w2856) -> ("Value"=w2854:i32[])  [unwired: 1 in, 2 out]
            n951 = property class="Arr (strict)"(reference=w2857) -> ("Value"=w2855:i32[])  [unwired: 1 in, 2 out]
            n952 = property class="Arr (strict)"(reference=w2858) -> ("Value"=w2859:i32[])  [unwired: 1 in, 2 out]
            n953 = Index Array(array=w2859, index=2) -> (element=w2867:i32)
            n954 = Index Array(array=w2854) -> (element #1=w2869:i32, element #2=w2868:i32)  [unwired: 2 in]
            n955 = Index Array(array=w2855) -> (element #1=w2871:i32, element #2=w2870:i32)  [unwired: 2 in]
            n956 = Build Array(w2871, w2870, w2867) -> (w2865:i32[])
            n957 = Build Array(w2869, w2868, w2867) -> (w2866:i32[])
          }
        }
        n958 = property class="Clust (strict)"(reference=w2765) -> ("Value"=w2764:T29)  [unwired: 1 in, 2 out]
        n959 = property on="Property Node" class="Str"(reference=w2767, error in=w2709, "Value"="initiating cleaning...") -> (reference out=w2684:refnum<vi>, error out=w2733:errorcluster)
        n960 = call "setPressure_topLvl.vi"("which manipulator"=w2762, "Slide Refnum"=w2772, "error in"=w2733, "set pressure (mBar)"=200.0 ("Val"), "Pressure box control in"=w2711) -> ("error out"=w2735:errorcluster, "Pressure box control out"=w2706:T22)  [unwired: 5 in]
        n961 = property on="Property Node" class="Str"(reference=w2684, error in=w2735, "Value"="moving above cleaning bath..." ("cleaning status")) -> (reference out=w2683:refnum<vi>, error out=w2696:errorcluster)
        n962 = call "moveTo_abs_XYZ.vi"("blocking?"=TRUE, "error in"=w2696, "XYZ location (steps)"=w2703, "Actuator cluster in"=w2710) -> ("error out"=w2707:errorcluster, "Actuator cluster out"=w2708:T25)  [unwired: 6 in]
        n963 = case shown="\"clean\", Default" "protocol" {
          selector: "protocol" -> [w2825 w2846]
          tunnel: [w2825 w2846] -> w2726
          tunnel: w2708 -> [w2824 w2844]
          tunnel: w2703 -> [w2823 _]
          tunnel: w2700 -> [_ w2845]
          tunnel: w2707 -> [w2822 w2843]
          tunnel: w2706 -> [w2821 w2840]
          tunnel: [w2817 w2842] -> w2670
          tunnel: [w2818 w2841] -> w2668
          tunnel: [w2821 w2840] -> w2705
          tunnel: w2768 -> [w2816 w2839]
          tunnel: w2687 -> [w2815 w2838]
          tunnel: w2764 -> [w2814 w2833]
          tunnel: w2685 -> [_ w2837]
          tunnel: w2683 -> [w2813 w2836]
          tunnel: [w2811 w2834] -> w2682
          tunnel: w2674 -> [w2810 _]
          tunnel: w2762 -> [w2808 w2832]
          tunnel: [w2809 w2831] -> w2669
          frame "clean", Default {
            n964 = property on="Property Node" class="Str"(reference=w2813, error in=w2822, "Value"="moving above cleaning bath..." ("cleaning status")) -> (reference out=w2812:refnum<vi>, error out=w2829:errorcluster)
            n965 = call "moveTo_abs_XYZ.vi"("blocking?"=TRUE, "error in"=w2829, "XYZ location (steps)"=w2823, "Actuator cluster in"=w2824) -> ("error out"=w2827:errorcluster, "Actuator cluster out"=w2820:T25)  [unwired: 6 in]
            n966 = property on="Property Node" class="Str"(reference=w2812, error in=w2827, "Value"="dipping into cleaning bath..." ("cleaning status")) -> (reference out=w2811:refnum<vi>, error out=w2819:errorcluster)
            n967 = call "detectFluidTouch.vi"("which manipulator"=w2808, "lowest position"=w2810, "avg peak height Refnum"=w2816, "error in"=w2819, "mclamp cluster"=w2814, "Multiclamp Handle in"=w2815, "manip in"=w2820) -> ("error out"=w2818:errorcluster, "detected"=w2809:bool, "manip out"=w2817:T25)  [unwired: 2 in]
          }
          frame "sham" {
            n968 = property on="Property Node" class="Str"(reference=w2836, error in=w2843, "Value"="moving above wash (sham) bath..." ("cleaning status")) -> (reference out=w2835:refnum<vi>, error out=w2848:errorcluster)
            n969 = call "moveTo_abs_XYZ.vi"("blocking?"=TRUE, "error in"=w2848, "XYZ location (steps)"=w2845, "Actuator cluster in"=w2844) -> ("error out"=w2850:errorcluster, "Actuator cluster out"=w2853:T25)  [unwired: 6 in]
            n970 = property on="Property Node" class="Str"(reference=w2835, error in=w2850, "Value"="dipping into wash (sham) bath..." ("cleaning status")) -> (reference out=w2834:refnum<vi>, error out=w2849:errorcluster)
            n971 = call "detectFluidTouch.vi"("which manipulator"=w2832, "lowest position"=w2837, "avg peak height Refnum"=w2839, "error in"=w2849, "mclamp cluster"=w2833, "Multiclamp Handle in"=w2838, "manip in"=w2853) -> ("error out"=w2841:errorcluster, "detected"=w2831:bool, "manip out"=w2842:T25)  [unwired: 2 in]
          }
        }
        n972 = case shown="\"manipulator 4\"" w2762 {
          tunnel: w2763 -> [w2891 w2893 w2895 w2897]
          tunnel: [w2890 w2892 w2894 w2896] -> w2761
          frame "manipulator 1", Default {
            n973 = Unbundle By Name(w2891) -> ("manip 1"=w2890:refnum<vi>)
          }
          frame "manipulator 2" {
            n974 = Unbundle By Name(w2893) -> ("manip 2"=w2892:refnum<vi>)
          }
          frame "manipulator 3" {
            n975 = Unbundle By Name(w2895) -> ("manip 3"=w2894:refnum<vi>)
          }
          frame "manipulator 4" {
            n976 = Unbundle By Name(w2897) -> ("manip 4"=w2896:refnum<vi>)
          }
        }
        n977 = property class="Bool (strict)"(reference=w2769) -> ("Value"=w2686:bool)  [unwired: 1 in, 2 out]
        n978 = property on="Property Node" class="Bool (strict)"(reference=w2758, error in=w2668, "Value"=w2669) -> (error out=w2667:errorcluster)  [unwired: 1 out]
        n979 = Not(x=w2669) -> (.not. x?=w2756:bool)
        n980 = property on="Property Node" class="Clust (strict)"(reference=w2761) -> ("Value"=w2760:T24)  [unwired: 1 in, 2 out]
        n981 = property on="Property Node" class="Str"(reference=w2682, error in=w2667, "Value"="cleaning protocol..." ("cleaning status")) -> (reference out=w2681:refnum<vi>, error out=w2728:errorcluster)
        n982 = case shown="False" w2686 {
          tunnel: "Cleaning step (time [s], value [mBar]) actual" -> [w2790 _]
          tunnel: w2728 -> [w2789 w2793]
          tunnel: [w2788 w2793] -> w2727
          tunnel: w2705 -> [w2787 w2792]
          tunnel: [w2786 w2792] -> w2698
          tunnel: w2772 -> [w2785 _]
          tunnel: w2762 -> [w2784 _]
          frame False {
            n983 = call "execute_protocol_topLvl.vi"("which manipulator"=w2784, "Slide Refnum"=w2785, "error in"=w2789, "protocol array"=w2790, "Pressure box control in"=w2787) -> ("error out"=w2788:errorcluster, "Pressure box control out"=w2786:T22)  [unwired: 5 in]
          }
          frame True {
            n984 = Wait (ms)(milliseconds to wait=u32 1000) -> ()  [unwired: 1 out]
          }
        }
        n985 = property on="Property Node" class="Str"(reference=w2681, error in=w2727, "Value"="raising..." ("cleaning status")) -> (reference out=w2680:refnum<vi>, error out=w2704:errorcluster)
        n986 = Unbundle By Name(w2760) -> ("safe space (steps)"=w2759:i32[])
        n987 = case shown="\"clean\", Default" w2726 {
          tunnel: w2704 -> [w2800 w2806]
          tunnel: w2670 -> [w2799 w2807]
          tunnel: w2700 -> [_ w2804]
          tunnel: w2703 -> [w2798 _]
          tunnel: [w2797 w2803] -> w2701
          tunnel: [w2796 w2802] -> w2702
          tunnel: [w2794 w2801] -> w2697
          tunnel: w2698 -> [w2794 w2801]
          frame "clean", Default {
            n988 = call "moveTo_abs_XYZ.vi"("blocking?"=TRUE, "error in"=w2800, "XYZ location (steps)"=w2798, "Actuator cluster in"=w2799) -> ("error out"=w2796:errorcluster, "Actuator cluster out"=w2797:T25)  [unwired: 6 in]
          }
          frame "sham" {
            n989 = call "moveTo_abs_XYZ.vi"("blocking?"=TRUE, "error in"=w2806, "XYZ location (steps)"=w2804, "Actuator cluster in"=w2807) -> ("error out"=w2802:errorcluster, "Actuator cluster out"=w2803:T25)  [unwired: 6 in]
          }
        }
        n990 = property on="Property Node" class="Str"(reference=w2680, error in=w2702, "Value"="moving to wash bath..." ("cleaning status")) -> (reference out=w2679:refnum<vi>, error out=w2723:errorcluster)
        n991 = call "moveTo_abs_XYZ.vi"("blocking?"=w2699, "error in"=w2723, "XYZ location (steps)"=w2700, "Actuator cluster in"=w2701) -> ("error out"=w2721:errorcluster, "Actuator cluster out"=w2722:T25)  [unwired: 6 in]
        n992 = property on="Property Node" class="Str"(reference=w2679, error in=w2721, "Value"="dipping to wash bath..." ("cleaning status")) -> (reference out=w2678:refnum<vi>, error out=w2720:errorcluster)
        n993 = call "detectFluidTouch.vi"("which manipulator"=w2762, "lowest position"=w2685, "avg peak height Refnum"=w2768, "error in"=w2720, "mclamp cluster"=w2764, "Multiclamp Handle in"=w2687, "manip in"=w2722) -> ("error out"=w2671:errorcluster, "detected"=w2673:bool, "manip out"=w2672:T25)  [unwired: 2 in]
        n994 = property on="Property Node" class="Str"(reference=w2678, error in=w2671, "Value"="post-washing..." ("cleaning status")) -> (reference out=w2677:refnum<vi>, error out=w2718:errorcluster)
        n995 = case shown="False" w2686 {
          tunnel: w2718 -> [w2780 w2783]
          tunnel: [w2779 w2783] -> w2717
          tunnel: "Wash step (time [s], value [mBar]) actual" -> [w2778 _]
          tunnel: w2697 -> [w2777 w2782]
          tunnel: w2772 -> [w2776 _]
          tunnel: [w2775 w2782] -> w2689
          tunnel: w2762 -> [w2774 _]
          frame False {
            n996 = call "execute_protocol_topLvl.vi"("which manipulator"=w2774, "Slide Refnum"=w2776, "error in"=w2780, "protocol array"=w2778, "Pressure box control in"=w2777) -> ("error out"=w2779:errorcluster, "Pressure box control out"=w2775:T22)  [unwired: 5 in]
          }
          frame True {
            n997 = Wait (ms)(milliseconds to wait=u32 1000) -> ()  [unwired: 1 out]
          }
        }
        n998 = property on="Property Node" class="Bool (strict)"(reference=w2757, "Value"=w2673) -> ()  [unwired: 1 in, 2 out]
        n999 = property on="Property Node" class="Str"(reference=w2677, error in=w2717, "Value"="raising above wash bath..." ("cleaning status")) -> (reference out=w2676:refnum<vi>, error out=w2715:errorcluster)
        n1000 = Unbundle By Name(w2689) -> ("Low pos pressure (mBar)"=w2688:dbl)
        n1001 = call "moveTo_abs_XYZ.vi"("blocking?"=w2699, "error in"=w2715, "XYZ location (steps)"=w2700, "Actuator cluster in"=w2672) -> ("error out"=w2714:errorcluster, "Actuator cluster out"=w2695:T25)  [unwired: 6 in]
        n1002 = property on="Property Node" class="Str"(reference=w2676, error in=w2714, "Value"="moving to exp bath location..." ("cleaning status")) -> (reference out=w2675:refnum<vi>, error out=w2690:errorcluster)
        n1003 = call "setPressure_topLvl.vi"("which manipulator"=w2762, "Slide Refnum"=w2772, "error in"=w2690, "set pressure (mBar)"=w2688, "Pressure box control in"=w2689) -> ("error out"=w2694:errorcluster)  [unwired: 5 in, 1 out]
        n1004 = call "moveTo_abs_XYZ.vi"("blocking?"=TRUE, "error in"=w2694, "XYZ location (steps)"=w2759, "Actuator cluster in"=w2695) -> ("error out"=w2692:errorcluster, "Actuator cluster out"=w2748:T25)  [unwired: 6 in]
        n1005 = property on="Property Node" class="Str"(reference=w2675, error in=w2692, "Value"="protocol complete" ("cleaning status")) -> (error out=w2666:errorcluster)  [unwired: 1 out]
        n1006 = case shown="True" w2756 {
          tunnel: w2755 -> [_ w2889]
          tunnel: w2666 -> [w2875 w2879]
          tunnel: [w2875 w2877] -> w2665
          frame False {
          }
          frame True {
            n1007 = call <vilib>:"Play Sound File.vi"("error in (no error)"=w2879, "path"=path "C:/multiBot/patcherBot/sounds/The QI Klaxon.wav") -> ("error out"=w2878:errorcluster)  [unwired: 8 in, 1 out]
            n1008 = property class="DigNum (strict)"(reference=w2889, error in=w2878) -> (error out=w2882:errorcluster, "Value"=w2888:i32)  [unwired: 1 out]
            "cell number when cleaning fail" <- w2888
            n1009 = Number To Decimal String(number=w2888) -> (decimal integer string=w2885:string)  [unwired: 1 in]
            n1010 = Concatenate Strings("HELP! No fluid in my bath! \\n" ("string"), "Failed on cell #" ("string"), w2885) -> (w2881:string)
            n1011 = One Button Dialog(message=w2881, button name ("OK")="click to advance") -> ()  [unwired: 1 out]
            n1012 = call "jsontest.vi"("error in (no error)"=w2882, "string"=w2881) -> ("error out"=w2884:errorcluster)  [unwired: 9 in]
            n1013 = call "Bath Refill Delay"("error in (no error)"=w2884, "Delay Time (s)"=1.0) -> ("error out"=w2877:errorcluster)  [unwired: 9 in]
          }
        }
        n1014 = Unbundle By Name(w2745) -> ("misc indiv.In Process Calibration?"=w2744:refnum<vi>)
        n1015 = property class="Bool (strict)"(reference=w2744) -> ("Value"=w2743:bool)  [unwired: 1 in, 2 out]
        n1016 = call <vilib>:"Play Sound File.vi"("error in (no error)"=w2665, "path"=path "C:/multiBot/patcherBot/sounds/ness04.dsp.wav") -> ("error out"=w2741:errorcluster)  [unwired: 8 in, 1 out]
        n1017 = case shown="False" w2743 {
          tunnel: [user_message_v6."Starting new attempt..." ("Message to user") user_message_v6."In Process Calibration" ("Message to user")] -> w2770
          frame False {
          }
          frame True {
          }
        }
        n1018 = call "Time Delay32"("error in (no error)"=w2741, "Delay Time (s)"=0.2) -> ("error out"=w2739:errorcluster)  [unwired: 9 in]
        n1019 = Unbundle By Name(w2748) -> ("Actuator COM"=w2747:refnum<visa-resource-name>)
        n1020 = call "sc_adjustMotion.vi"("error in (no error)"=w2739, "motion"=scope_motion."slow_dualPatch", "VISA handle"=w2747) -> ("error out"=w2749:errorcluster)  [unwired: 7 in, 1 out]
      }
      frame "reclean" {
        w2944 = TRUE ("blocking?")
        # "go back to safe location"
        # "if this is the last cell in the list, quit"
        n1021 = Unbundle By Name(w2904) -> ("Actuator COM"=w2994:refnum<visa-resource-name>)
        n1022 = Unbundle By Name(w2902) -> ("state UI indiv.demo clean"=w3009:refnum<vi>, "cleaning indiv.avg peak height"=w3008:refnum<vi>, "cleaning indiv.cleaning status"=w3007:refnum<vi>, "cleaning indiv.clean bath detected"=w2999:refnum<vi>, "cleaning indiv.wash bath detected"=w2998:refnum<vi>)
        n1023 = Unbundle By Name(w3006) -> ("misc common.mclamp cluster"=w3005:refnum<vi>)
        n1024 = call "sc_adjustMotion.vi"("error in (no error)"=w2995, "motion"=scope_motion."fast", "VISA handle"=w2994) -> ("error out"=w2906:errorcluster)  [unwired: 7 in, 1 out]
        n1025 = case shown="\"manipulator 1\", Default" w2903 {
          tunnel: w2901 -> [w3023 w3025 w3027 w3029]
          tunnel: [w3022 w3024 w3026 w3028] -> w2909
          frame "manipulator 1", Default {
            n1026 = Unbundle By Name(w3023) -> ("manip 1"=w3022:refnum<vi>)
          }
          frame "manipulator 2" {
            n1027 = Unbundle By Name(w3025) -> ("manip 2"=w3024:refnum<vi>)
          }
          frame "manipulator 3" {
            n1028 = Unbundle By Name(w3027) -> ("manip 3"=w3026:refnum<vi>)
          }
          frame "manipulator 4" {
            n1029 = Unbundle By Name(w3029) -> ("manip 4"=w3028:refnum<vi>)
          }
        }
        n1030 = property on="Property Node" class="Clust (strict)"(reference=w2909) -> ("Value"=w2908:T24)  [unwired: 1 in, 2 out]
        n1031 = Unbundle By Name(w2908) -> ("safe space (steps)"=w2905:i32[])
        n1032 = call "moveTo_abs_XYZ.vi"("blocking?"=TRUE, "error in"=w2906, "XYZ location (steps)"=w2905, "Actuator cluster in"=w2904) -> ("error out"=w2900:errorcluster)  [unwired: 6 in, 1 out]
        n1033 = disable-structure shown="Disabled" {
          disable-tunnel: w2900 -> [w3020 w3021]
          disable-tunnel: [w3019 w3021] -> w2899
          disable-tunnel: w2898 -> [w3018 _]
          frame Disabled {
            n1034 = property class="DigNum (strict)"(reference=w3018, error in=w3020) -> (reference out=w3017:refnum<vi>, error out=w3014:errorcluster, "Value"=w3016:i32)
            n1035 = Decrement(x=w3016) -> (x-1=w3015:i32)
            n1036 = property class="DigNum (strict)"(reference=w3017, error in=w3014, "Value"=w3015) -> (error out=w3019:errorcluster)  [unwired: 1 out]
          }
          frame Enabled {
          }
        }
        n1037 = property class="Clust (strict)"(reference=w3005) -> ("Value"=w3004:T29)  [unwired: 1 in, 2 out]
        n1038 = flat-sequence {
          tunnel: [w3119] -> w2955
          tunnel: [w3120] -> w2954
          tunnel: [w3122] -> w2948
          tunnel: [w3121] -> w2945
          tunnel: w2904 -> [w3119]
          tunnel: w2899 -> [w3120]
          tunnel: w3013 -> [w3118]
          tunnel: [w3118] -> w2956
          tunnel: [w3117] -> w2932
          tunnel: w3011 -> [w3117]
          tunnel: [w3111] -> w2930
          tunnel: w2902 -> [w3116]
          tunnel: [w3110] -> w2919
          frame #0 {
            # "REPLACE ALL"
            # "calculate positions (x_wash, y_wash, z_above)"
            n1039 = Unbundle By Name(w3116) -> ("cleaning indiv.loc above baths"=w3114:refnum<vi>, "cleaning indiv.wash bath loc"=w3113:refnum<vi>, "cleaning indiv.cleaning bath loc"=w3112:refnum<vi>)
            n1040 = property class="Arr (strict)"(reference=w3112) -> ("Value"=w3110:i32[])  [unwired: 1 in, 2 out]
            n1041 = property class="Arr (strict)"(reference=w3113) -> ("Value"=w3111:i32[])  [unwired: 1 in, 2 out]
            n1042 = property class="Arr (strict)"(reference=w3114) -> ("Value"=w3115:i32[])  [unwired: 1 in, 2 out]
            n1043 = Index Array(array=w3115, index=2) -> (element=w3123:i32)
            n1044 = Index Array(array=w3110) -> (element #1=w3125:i32, element #2=w3124:i32)  [unwired: 2 in]
            n1045 = Index Array(array=w3111) -> (element #1=w3127:i32, element #2=w3126:i32)  [unwired: 2 in]
            n1046 = Build Array(w3127, w3126, w3123) -> (w3121:i32[])
            n1047 = Build Array(w3125, w3124, w3123) -> (w3122:i32[])
          }
        }
        n1048 = property on="Property Node" class="Str"(reference=w3007, error in=w2954, "Value"="initiating cleaning...") -> (reference out=w2929:refnum<vi>, error out=w2978:errorcluster)
        n1049 = case shown="\"manipulator 4\"" w3003 {
          tunnel: w2901 -> [w3147 w3149 w3151 w3153]
          tunnel: [w3146 w3148 w3150 w3152] -> w3002
          frame "manipulator 1", Default {
            n1050 = Unbundle By Name(w3147) -> ("manip 1"=w3146:refnum<vi>)
          }
          frame "manipulator 2" {
            n1051 = Unbundle By Name(w3149) -> ("manip 2"=w3148:refnum<vi>)
          }
          frame "manipulator 3" {
            n1052 = Unbundle By Name(w3151) -> ("manip 3"=w3150:refnum<vi>)
          }
          frame "manipulator 4" {
            n1053 = Unbundle By Name(w3153) -> ("manip 4"=w3152:refnum<vi>)
          }
        }
        n1054 = call "setPressure_topLvl.vi"("which manipulator"=w3003, "Slide Refnum"=w3012, "error in"=w2978, "set pressure (mBar)"=200.0 ("Val"), "Pressure box control in"=w2956) -> ("error out"=w2980:errorcluster, "Pressure box control out"=w2951:T22)  [unwired: 5 in]
        n1055 = property on="Property Node" class="Str"(reference=w2929, error in=w2980, "Value"="moving above cleaning bath..." ("cleaning status")) -> (reference out=w2928:refnum<vi>, error out=w2941:errorcluster)
        n1056 = call "moveTo_abs_XYZ.vi"("blocking?"=TRUE, "error in"=w2941, "XYZ location (steps)"=w2948, "Actuator cluster in"=w2955) -> ("error out"=w2952:errorcluster, "Actuator cluster out"=w2953:T25)  [unwired: 6 in]
        n1057 = property class="Bool (strict)"(reference=w3009) -> ("Value"=w2931:bool)  [unwired: 1 in, 2 out]
        n1058 = case shown="\"clean\", Default" "protocol 2" {
          selector: "protocol 2" -> [w3081 w3102]
          tunnel: [w3081 w3102] -> w2971
          tunnel: w2953 -> [w3080 w3100]
          tunnel: w2948 -> [w3079 _]
          tunnel: w2945 -> [_ w3101]
          tunnel: w2952 -> [w3078 w3099]
          tunnel: w2951 -> [w3077 w3096]
          tunnel: [w3073 w3098] -> w2915
          tunnel: [w3074 w3097] -> w2913
          tunnel: [w3077 w3096] -> w2950
          tunnel: w3008 -> [w3072 w3095]
          tunnel: w2932 -> [w3071 w3094]
          tunnel: w3004 -> [w3070 w3089]
          tunnel: w2930 -> [_ w3093]
          tunnel: w2928 -> [w3069 w3092]
          tunnel: [w3067 w3090] -> w2927
          tunnel: w2919 -> [w3066 _]
          tunnel: w3003 -> [w3064 w3088]
          tunnel: [w3065 w3087] -> w2914
          frame "clean", Default {
            n1059 = property on="Property Node" class="Str"(reference=w3069, error in=w3078, "Value"="moving above cleaning bath..." ("cleaning status")) -> (reference out=w3068:refnum<vi>, error out=w3085:errorcluster)
            n1060 = call "moveTo_abs_XYZ.vi"("blocking?"=TRUE, "error in"=w3085, "XYZ location (steps)"=w3079, "Actuator cluster in"=w3080) -> ("error out"=w3083:errorcluster, "Actuator cluster out"=w3076:T25)  [unwired: 6 in]
            n1061 = property on="Property Node" class="Str"(reference=w3068, error in=w3083, "Value"="dipping into cleaning bath..." ("cleaning status")) -> (reference out=w3067:refnum<vi>, error out=w3075:errorcluster)
            n1062 = call "detectFluidTouch.vi"("which manipulator"=w3064, "lowest position"=w3066, "avg peak height Refnum"=w3072, "error in"=w3075, "mclamp cluster"=w3070, "Multiclamp Handle in"=w3071, "manip in"=w3076) -> ("error out"=w3074:errorcluster, "detected"=w3065:bool, "manip out"=w3073:T25)  [unwired: 2 in]
          }
          frame "sham" {
            n1063 = property on="Property Node" class="Str"(reference=w3092, error in=w3099, "Value"="moving above wash (sham) bath..." ("cleaning status")) -> (reference out=w3091:refnum<vi>, error out=w3104:errorcluster)
            n1064 = call "moveTo_abs_XYZ.vi"("blocking?"=TRUE, "error in"=w3104, "XYZ location (steps)"=w3101, "Actuator cluster in"=w3100) -> ("error out"=w3106:errorcluster, "Actuator cluster out"=w3109:T25)  [unwired: 6 in]
            n1065 = property on="Property Node" class="Str"(reference=w3091, error in=w3106, "Value"="dipping into wash (sham) bath..." ("cleaning status")) -> (reference out=w3090:refnum<vi>, error out=w3105:errorcluster)
            n1066 = call "detectFluidTouch.vi"("which manipulator"=w3088, "lowest position"=w3093, "avg peak height Refnum"=w3095, "error in"=w3105, "mclamp cluster"=w3089, "Multiclamp Handle in"=w3094, "manip in"=w3109) -> ("error out"=w3097:errorcluster, "detected"=w3087:bool, "manip out"=w3098:T25)  [unwired: 2 in]
          }
        }
        n1067 = Not(x=w2914) -> (.not. x?=w2997:bool)
        n1068 = property on="Property Node" class="Clust (strict)"(reference=w3002) -> ("Value"=w3001:T24)  [unwired: 1 in, 2 out]
        n1069 = property on="Property Node" class="Bool (strict)"(reference=w2999, error in=w2913, "Value"=w2914) -> (error out=w2912:errorcluster)  [unwired: 1 out]
        n1070 = property on="Property Node" class="Str"(reference=w2927, error in=w2912, "Value"="cleaning protocol..." ("cleaning status")) -> (reference out=w2926:refnum<vi>, error out=w2973:errorcluster)
        n1071 = case shown="False" w2931 {
          tunnel: "Cleaning step (time [s], value [mBar]) actual 2" -> [w3046 _]
          tunnel: w2973 -> [w3045 w3049]
          tunnel: [w3044 w3049] -> w2972
          tunnel: w2950 -> [w3043 w3048]
          tunnel: [w3042 w3048] -> w2943
          tunnel: w3012 -> [w3041 _]
          tunnel: w3003 -> [w3040 _]
          frame False {
            n1072 = call "execute_protocol_topLvl.vi"("which manipulator"=w3040, "Slide Refnum"=w3041, "error in"=w3045, "protocol array"=w3046, "Pressure box control in"=w3043) -> ("error out"=w3044:errorcluster, "Pressure box control out"=w3042:T22)  [unwired: 5 in]
          }
          frame True {
            n1073 = Wait (ms)(milliseconds to wait=u32 1000) -> ()  [unwired: 1 out]
          }
        }
        n1074 = property on="Property Node" class="Str"(reference=w2926, error in=w2972, "Value"="raising..." ("cleaning status")) -> (reference out=w2925:refnum<vi>, error out=w2949:errorcluster)
        n1075 = Unbundle By Name(w3001) -> ("safe space (steps)"=w3000:i32[])
        n1076 = case shown="\"clean\", Default" w2971 {
          tunnel: w2949 -> [w3056 w3062]
          tunnel: w2915 -> [w3055 w3063]
          tunnel: w2945 -> [_ w3060]
          tunnel: w2948 -> [w3054 _]
          tunnel: [w3053 w3059] -> w2946
          tunnel: [w3052 w3058] -> w2947
          tunnel: [w3050 w3057] -> w2942
          tunnel: w2943 -> [w3050 w3057]
          frame "clean", Default {
            n1077 = call "moveTo_abs_XYZ.vi"("blocking?"=TRUE, "error in"=w3056, "XYZ location (steps)"=w3054, "Actuator cluster in"=w3055) -> ("error out"=w3052:errorcluster, "Actuator cluster out"=w3053:T25)  [unwired: 6 in]
          }
          frame "sham" {
            n1078 = call "moveTo_abs_XYZ.vi"("blocking?"=TRUE, "error in"=w3062, "XYZ location (steps)"=w3060, "Actuator cluster in"=w3063) -> ("error out"=w3058:errorcluster, "Actuator cluster out"=w3059:T25)  [unwired: 6 in]
          }
        }
        n1079 = property on="Property Node" class="Str"(reference=w2925, error in=w2947, "Value"="moving to wash bath..." ("cleaning status")) -> (reference out=w2924:refnum<vi>, error out=w2968:errorcluster)
        n1080 = call "moveTo_abs_XYZ.vi"("blocking?"=w2944, "error in"=w2968, "XYZ location (steps)"=w2945, "Actuator cluster in"=w2946) -> ("error out"=w2966:errorcluster, "Actuator cluster out"=w2967:T25)  [unwired: 6 in]
        n1081 = property on="Property Node" class="Str"(reference=w2924, error in=w2966, "Value"="dipping to wash bath..." ("cleaning status")) -> (reference out=w2923:refnum<vi>, error out=w2965:errorcluster)
        n1082 = call "detectFluidTouch.vi"("which manipulator"=w3003, "lowest position"=w2930, "avg peak height Refnum"=w3008, "error in"=w2965, "mclamp cluster"=w3004, "Multiclamp Handle in"=w2932, "manip in"=w2967) -> ("error out"=w2916:errorcluster, "detected"=w2918:bool, "manip out"=w2917:T25)  [unwired: 2 in]
        n1083 = property on="Property Node" class="Str"(reference=w2923, error in=w2916, "Value"="post-washing..." ("cleaning status")) -> (reference out=w2922:refnum<vi>, error out=w2963:errorcluster)
        n1084 = case shown="False" w2931 {
          tunnel: w2963 -> [w3036 w3039]
          tunnel: [w3035 w3039] -> w2962
          tunnel: "Wash step (time [s], value [mBar]) actual 2" -> [w3034 _]
          tunnel: w2942 -> [w3033 w3038]
          tunnel: w3012 -> [w3032 _]
          tunnel: [w3031 w3038] -> w2934
          tunnel: w3003 -> [w3030 _]
          frame False {
            n1085 = call "execute_protocol_topLvl.vi"("which manipulator"=w3030, "Slide Refnum"=w3032, "error in"=w3036, "protocol array"=w3034, "Pressure box control in"=w3033) -> ("error out"=w3035:errorcluster, "Pressure box control out"=w3031:T22)  [unwired: 5 in]
          }
          frame True {
            n1086 = Wait (ms)(milliseconds to wait=u32 1000) -> ()  [unwired: 1 out]
          }
        }
        n1087 = property on="Property Node" class="Bool (strict)"(reference=w2998, "Value"=w2918) -> ()  [unwired: 1 in, 2 out]
        n1088 = property on="Property Node" class="Str"(reference=w2922, error in=w2962, "Value"="raising above wash bath..." ("cleaning status")) -> (reference out=w2921:refnum<vi>, error out=w2960:errorcluster)
        n1089 = Unbundle By Name(w2934) -> ("Low pos pressure (mBar)"=w2933:dbl)
        n1090 = call "moveTo_abs_XYZ.vi"("blocking?"=w2944, "error in"=w2960, "XYZ location (steps)"=w2945, "Actuator cluster in"=w2917) -> ("error out"=w2959:errorcluster, "Actuator cluster out"=w2940:T25)  [unwired: 6 in]
        n1091 = property on="Property Node" class="Str"(reference=w2921, error in=w2959, "Value"="moving to exp bath location..." ("cleaning status")) -> (reference out=w2920:refnum<vi>, error out=w2935:errorcluster)
        n1092 = call "setPressure_topLvl.vi"("which manipulator"=w3003, "Slide Refnum"=w3012, "error in"=w2935, "set pressure (mBar)"=w2933, "Pressure box control in"=w2934) -> ("error out"=w2939:errorcluster)  [unwired: 5 in, 1 out]
        n1093 = call "moveTo_abs_XYZ.vi"("blocking?"=TRUE, "error in"=w2939, "XYZ location (steps)"=w3000, "Actuator cluster in"=w2940) -> ("error out"=w2937:errorcluster, "Actuator cluster out"=w2992:T25)  [unwired: 6 in]
        n1094 = property on="Property Node" class="Str"(reference=w2920, error in=w2937, "Value"="protocol complete" ("cleaning status")) -> (error out=w2911:errorcluster)  [unwired: 1 out]
        n1095 = case shown="True" w2997 {
          tunnel: w2898 -> [_ w3145]
          tunnel: w2911 -> [w3131 w3135]
          tunnel: [w3131 w3133] -> w2910
          frame False {
          }
          frame True {
            n1096 = call <vilib>:"Play Sound File.vi"("error in (no error)"=w3135, "path"=path "C:/multiBot/patcherBot/sounds/The QI Klaxon.wav") -> ("error out"=w3134:errorcluster)  [unwired: 8 in, 1 out]
            n1097 = property class="DigNum (strict)"(reference=w3145, error in=w3134) -> (error out=w3138:errorcluster, "Value"=w3144:i32)  [unwired: 1 out]
            "cell number when cleaning fail 2" <- w3144
            n1098 = Number To Decimal String(number=w3144) -> (decimal integer string=w3141:string)  [unwired: 1 in]
            n1099 = Concatenate Strings("HELP! No fluid in my bath! \\n" ("string"), "Failed on cell #" ("string"), w3141) -> (w3137:string)
            n1100 = One Button Dialog(message=w3137, button name ("OK")="click to advance") -> ()  [unwired: 1 out]
            n1101 = call "jsontest.vi"("error in (no error)"=w3138, "string"=w3137) -> ("error out"=w3140:errorcluster)  [unwired: 9 in]
            n1102 = call "Bath Refill Delay2"("error in (no error)"=w3140, "Delay Time (s)"=1.0) -> ("error out"=w3133:errorcluster)  [unwired: 9 in]
          }
        }
        n1103 = Unbundle By Name(w2902) -> ("misc indiv.In Process Calibration?"=w2989:refnum<vi>)
        n1104 = property class="Bool (strict)"(reference=w2989) -> ("Value"=w2988:bool)  [unwired: 1 in, 2 out]
        n1105 = call <vilib>:"Play Sound File.vi"("error in (no error)"=w2910, "path"=path "C:/multiBot/patcherBot/sounds/ness04.dsp.wav") -> ("error out"=w2986:errorcluster)  [unwired: 8 in, 1 out]
        n1106 = case shown="False" w2988 {
          tunnel: [user_message_v6."Starting new attempt..." ("Message to user") user_message_v6."In Process Calibration" ("Message to user")] -> w3010
          frame False {
          }
          frame True {
          }
        }
        n1107 = call "Time Delay24"("error in (no error)"=w2986, "Delay Time (s)"=0.2) -> ("error out"=w2984:errorcluster)  [unwired: 9 in]
        n1108 = Unbundle By Name(w2992) -> ("Actuator COM"=w2991:refnum<visa-resource-name>)
        n1109 = call "sc_adjustMotion.vi"("error in (no error)"=w2984, "motion"=scope_motion."slow_dualPatch", "VISA handle"=w2991) -> ("error out"=w2993:errorcluster)  [unwired: 7 in, 1 out]
      }
      frame "Retracting pipette..." {
        w3159 = T28 7 items=["Grayscale (U8)", "Grayscale (I16)", "Grayscale (SGL)", "Complex (CSG)", "RGB (U32)", "HSL (U32)", "RGB (U64)", "Grayscale (U16)"] ("Image Type")
        # "create image buffer"
        # "when true, this used to use step retract for sucking up nucleus... Colby undid this for now..."
        # "set holding to 0 mV"
        # "blowout"
        # "move pipette to safe location"
        n1110 = Unbundle By Name(w3205) -> ("misc common.mclamp cluster"=w3204:refnum<vi>)
        n1111 = Unbundle By Name(w3211) -> ("misc indiv.retract distance (um)"=w3203:refnum<vi>, "state UI indiv.successful breakin"=w3197:refnum<vi>)
        n1112 = Unbundle By Name(w3155) -> ("slice image"=w3154:T9)
        n1113 = call "switchSolenoid_topLvl.vi"("which manipulator"=w3182, "error in (no error)"=w3185, "solenoidSwitch (T:atm; F: Reg)"=FALSE, "Pressure box control in"=w3186) -> ("error out"=w3183:errorcluster, "Pressure box control out"=w3187:T22)  [unwired: 6 in]
        n1114 = property class="DigNum (strict)"(reference=w3203) -> ("Value"=w3193:dbl)  [unwired: 1 in, 2 out]
        n1115 = property class="Bool (strict)"(reference=w3197) -> ("Value"=w3195:bool)  [unwired: 1 in, 2 out]
        n1116 = call "setPressure_topLvl.vi"("which manipulator"=w3182, "Slide Refnum"=w3181, "error in"=w3183, "set pressure (mBar)"=15.0, "Pressure box control in"=w3187) -> ("error out"=w3190:errorcluster, "Pressure box control out"=w3177:T22)  [unwired: 5 in]
        n1117 = call "Time Delay22"("error in (no error)"=w3190, "Delay Time (s)"=1.0) -> ("error out"=w3191:errorcluster)  [unwired: 9 in]
        n1118 = case shown="True" w3195 {
          tunnel: w3194 -> [w3294 w3300]
          tunnel: [w3293 w3297] -> w3176
          tunnel: [w3292 w3298] -> w3192
          tunnel: w3193 -> [w3291 w3299]
          tunnel: w3191 -> [w3290 w3296]
          tunnel: w3196 -> [w3289 w3295]
          frame False {
            n1119 = call "slow retract.vi"("reset motion"=w3289, "error in"=w3290, "retract distance (um)"=w3291, "manp in"=w3294) -> ("error out"=w3292:errorcluster, "manip out"=w3293:T25)  [unwired: 6 in]
          }
          frame True {
            n1120 = disable-structure shown="Disabled" {
              frame Disabled {
                n1121 = call "stepwise retract.vi"() -> ()  [unwired: 10 in, 2 out]
              }
              frame Enabled {
              }
            }
            n1122 = call "slow retract.vi"("reset motion"=w3295, "error in"=w3296, "retract distance (um)"=w3299, "manp in"=w3300) -> ("error out"=w3298:errorcluster, "manip out"=w3297:T25)  [unwired: 6 in]
          }
        }
        n1123 = case shown="True" w3210 {
          tunnel: w3220 -> [_ w3315]
          tunnel: w3219 -> [_ _]
          tunnel: w3192 -> [w3309 w3317]
          tunnel: [w3309 w3316] -> w3212
          tunnel: w3182 -> [_ w3312]
          tunnel: w3204 -> [_ w3311]
          frame False {
          }
          frame True {
            n1124 = property class="Clust (strict)"(reference=w3311) -> ("Value"=w3310:T29)  [unwired: 1 in, 2 out]
            n1125 = call "select_mclamp_channel.vi"("which manipulator"=w3312, "mclamp cluster"=w3310, "Multiclamp Handle In"=w3315) -> ("error"=w3313:i32, "Multiclamp Handle out"=w3314:u32)  [unwired: 6 in, 1 out]
            n1126 = call "mclamp_auto_offset.vi"("error in (no error)"=w3317, "Error in"=w3313, "Multiclamp Handle Out"=w3314) -> ("error out"=w3316:errorcluster)  [unwired: 7 in, 1 out]
          }
        }
        n1127 = call "Time Delay26"("error in (no error)"=w3212, "Delay Time (s)"=1.0) -> ("error out"=w3208:errorcluster)  [unwired: 9 in]
        n1128 = case shown="\"manipulator 4\"" w3182 {
          tunnel: w3202 -> [w3302 w3304 w3306 w3308]
          tunnel: [w3301 w3303 w3305 w3307] -> w3201
          frame "manipulator 1", Default {
            n1129 = Unbundle By Name(w3302) -> ("manip 1"=w3301:refnum<vi>)
          }
          frame "manipulator 2" {
            n1130 = Unbundle By Name(w3304) -> ("manip 2"=w3303:refnum<vi>)
          }
          frame "manipulator 3" {
            n1131 = Unbundle By Name(w3306) -> ("manip 3"=w3305:refnum<vi>)
          }
          frame "manipulator 4" {
            n1132 = Unbundle By Name(w3308) -> ("manip 4"=w3307:refnum<vi>)
          }
        }
        n1133 = property on="Property Node" class="Clust (strict)"(reference=w3201) -> ("Value"=w3200:T24)  [unwired: 1 in, 2 out]
        n1134 = call "switchSolenoid_topLvl.vi"("which manipulator"=w3182, "error in (no error)"=w3208, "solenoidSwitch (T:atm; F: Reg)"=FALSE ("solenoidSwitch"), "Pressure box control in"=w3177) -> ("error out"=w3207:errorcluster, "Pressure box control out"=w3209:T22)  [unwired: 6 in]
        n1135 = Unbundle By Name(w3200) -> ("safe space (steps)"=w3199:i32[])
        n1136 = call "setPressure_topLvl.vi"("which manipulator"=w3182, "Slide Refnum"=w3181, "error in"=w3207, "set pressure (mBar)"=1000.0, "Pressure box control in"=w3209) -> ("error out"=w3180:errorcluster, "Pressure box control out"=w3217:T22)  [unwired: 5 in]
        n1137 = call "Time Delay21"("error in (no error)"=w3180, "Delay Time (s)"=1.0) -> ("error out"=w3179:errorcluster)  [unwired: 9 in]
        n1138 = disable-structure shown="Enabled" {
          disable-tunnel: w3217 -> [w3271 w3288]
          disable-tunnel: [w3270 w3288] -> w3216
          disable-tunnel: [w3269 w3287] -> w3215
          disable-tunnel: w3198 -> [w3268 _]
          disable-tunnel: w3179 -> [w3267 w3287]
          frame Disabled {
            n1139 = while {
              tunnel: [w3282] -> w3270
              tunnel: [w3278] -> w3269
              tunnel: w3271 -> [w3282]
              tunnel: w3267 -> [w3279]
              tunnel: w3268 -> [w3281]
              i -> [w3276]
              stop <- w3272 stop-if-true
              n1140 = call "Time Delay23"("error in (no error)"=w3279, "Delay Time (s)"=0.2) -> ("error out"=w3278:errorcluster)  [unwired: 9 in]
              n1141 = property class="DigNum (strict)"(reference=w3281) -> ("Value"=w3280:dbl)  [unwired: 1 in, 2 out]
              n1142 = Less?(x=w3280, y=11.0) -> (x < y?=w3283:bool)
              n1143 = Greater?(x=w3276, y=50.0) -> (0:w3285:bool)
              n1144 = Or(x=w3283, y=w3285) -> (x .or. y?=w3273:bool)
              n1145 = Greater?(x=w3276, y=1) -> (0:w3274:bool)
              n1146 = And(x=w3274, y=w3273) -> (x .and. y?=w3272:bool)
            }
          }
          frame Enabled {
          }
        }
        n1147 = call "setPressure_topLvl.vi"("which manipulator"=w3182, "Slide Refnum"=w3181, "error in"=w3215, "set pressure (mBar)"=20.0, "Pressure box control in"=w3216) -> ("error out"=w3175:errorcluster)  [unwired: 5 in, 1 out]
        n1148 = call "reset manipulator.vi"("error in"=w3175, "motion"=scope_motion."fast", "manip in"=w3176) -> ("error out"=w3157:errorcluster, "manip out"=w3174:T25)  [unwired: 7 in]
        n1149 = call "IMAQ Create"("Border Size"=0, "Image Name"="temp", "Image Type"=w3159, "error in (no error)"=w3157) -> ("New Image"=w3158:T9, "error out"=w3156:errorcluster)  [unwired: 1 in]
        n1150 = while {
          tunnel: w3154 -> [w3252]
          tunnel: w3168 -> [w3266]
          tunnel: w3170 -> [w3245]
          tunnel: [w3244] -> w3166
          tunnel: w3156 -> [w3251]
          tunnel: "images/08-retracted.png" ("name or relative path") -> [w3263]
          tunnel: w3167 -> [w3261]
          tunnel: [w3243] -> w3164
          tunnel: [w3242] -> w3163
          tunnel: [w3241] -> w3162
          stop <- w3262 stop-if-true
          n1151 = property class="Bool (strict)"(reference=w3261) -> ("Value"=w3260:bool)  [unwired: 1 in, 2 out]
          n1152 = call "IMAQ GetImageSize"("Image"=w3252, "error in (no error)"=w3251) -> ("Y Resolution"=w3256:i32, "X Resolution"=w3259:i32, "error out"=w3250:errorcluster)  [unwired: 2 in]
          n1153 = call "IMAQ ImageToArray"("error in (no error)"=w3250, "Image"=w3252) -> ("Image Pixels (U16)"=w3241:u16[][], "error out"=w3244:errorcluster)  [unwired: 2 in, 3 out]
          n1154 = Add Array Elements(numeric array=w3241) -> (sum=w3249:u16)
          n1155 = Build Path(base path=w3266, name or relative path=w3263) -> (appended path=w3243:path)
          n1156 = Index Array(array=w3245) -> (element #1=w3258:i32, element #2=w3257:i32)  [unwired: 2 in]
          n1157 = Equal?(x=w3256, y=w3257) -> (x = y?=w3254:bool)
          n1158 = Greater?(x=w3249, y=u16 0) -> (0:w3246:bool)
          n1159 = Equal?(x=w3259, y=w3258) -> (x = y?=w3255:bool)
          n1160 = And(x=w3255, y=w3254) -> (x .and. y?=w3247:bool)
          n1161 = Wait (ms)(milliseconds to wait=u32 1000) -> ()  [unwired: 1 out]
          n1162 = And(x=w3247, y=w3246) -> (x .and. y?=w3240:bool)
          n1163 = Select(t="Ready", s=w3240, f="Before") -> (s? t:f=w3242:string)
          n1164 = Or(x=w3240, y=w3260) -> (x .or. y?=w3262:bool)
        }
        n1165 = case shown="\"Ready\"" w3163 {
          tunnel: w3164 -> [_ w3236 _]
          tunnel: [FALSE TRUE FALSE] -> _
          tunnel: w3166 -> [w3225 w3229 w3238]
          tunnel: [w3225 w3227 w3238] -> w3165
          tunnel: w3162 -> [_ w3233 _]
          tunnel: w3158 -> [_ w3232 _]
          frame "Before", Default {
          }
          frame "Ready" {
            n1166 = call "IMAQ ArrayToImage"("Image Pixels (U16)"=w3233, "error in (no error)"=w3229, "Image"=w3232) -> ("error out"=w3234:errorcluster, "Image Out"=w3230:T9)  [unwired: 7 in]
            n1167 = call-poly "IMAQ Write File 2"("error in (no error)"=w3234, "Image Quality"=u32 1000, "File Path"=w3236, "Image"=w3230) -> ("error out"=w3228:errorcluster)  [unwired: 6 in, 1 out]
            n1168 = call "IMAQ Dispose"("All Images? (No)"=FALSE, "Image"=w3230, "error in (no error)"=w3228) -> ("error out"=w3227:errorcluster)  [unwired: 3 in]
          }
          frame "After" {
          }
        }
        n1169 = call "Time Delay2"("error in (no error)"=w3165, "Delay Time (s)"=0.2) -> ("error out"=w3171:errorcluster)  [unwired: 9 in]
        n1170 = call "moveTo_abs_XYZ.vi"("blocking?"=TRUE, "error in"=w3171, "XYZ location (steps)"=w3199, "Actuator cluster in"=w3174) -> ("error out"=w3221:errorcluster)  [unwired: 6 in, 1 out]
      }
      frame "DEBUG STATE" {
        n1171 = case shown="True" w3320 {
          tunnel: w3319 -> [_ w3325]
          tunnel: [user_message_v6."DEBUG STATE" ("Message to user") "debug state"] -> w3318
          frame False {
          }
          frame True {
            n1172 = property class="Bool (strict)"(reference=w3325, "Value"=FALSE) -> ()  [unwired: 1 in, 2 out]
          }
        }
        n1173 = Wait (ms)(milliseconds to wait=u32 100) -> ()  [unwired: 1 out]
      }
      frame "Waiting to break in..." {
        w3353 = user_message_v6."Breaking in..." ("Value")
        # "if gigaseal\n        still have the cell -> wait for break in\notherwise\n       no cell. Go to unsuccessful breakin"
        # "CONTINUE MEASURING GS RESISTANCE HERE"
        # "if other manip is in break-in state, go to break-in state\notherwise, stay in waiting state"
        n1174 = Unbundle By Name(w3358) -> ("misc indiv.other state ref"=w3357:refnum<vi>, "gigaseal indiv.GIGASEALING MONITOR"=w3346:refnum<vi>, "gigaseal indiv.start GS time"=w3339:refnum<vi>)
        n1175 = property class="DigNum (strict)"(reference=w3345) -> ("Value"=w3344:dbl)  [unwired: 1 in, 2 out]
        n1176 = property class="Arr (strict)"(reference=w3348) -> (reference out=w3327:refnum<vi>, "Value"=w3347:i32[])  [unwired: 1 in, 1 out]
        n1177 = property class="DigNum (strict)"(reference=w3339) -> ("Value"=w3351:i32)  [unwired: 1 in, 2 out]
        n1178 = property class="Arr (strict)"(reference=w3343) -> (reference out=w3340:refnum<vi>, "Value"=w3342:dbl[])  [unwired: 1 in, 1 out]
        n1179 = Subtract(x=w3350, y=w3351) -> (x-y=w3349:i32)
        n1180 = Build Array (concatenate)(w3342, w3344) -> (w3331:dbl[])
        n1181 = Build Array (concatenate)(w3347, w3349) -> (w3326:i32[])
        n1182 = Bundle(w3326, w3331) -> (w3341:cluster{i32[], dbl[]})  [unwired: 1 out]
        n1183 = property class="XYGraph (strict)"(reference=w3346, "Value"=w3341) -> ()  [unwired: 1 in, 2 out]
        n1184 = property on="Property Node" class="Enum (strict)"(reference=w3357) -> ("Value"=w3356:T3)  [unwired: 1 in, 2 out]
        n1185 = Wait (ms)(milliseconds to wait=u32 1000) -> ()  [unwired: 1 out]
        n1186 = Equal?(x=w3356, y=w3353) -> (x = y?=w3355:bool)
        n1187 = Select(t=w3353, s=w3355, f=user_message_v6."Waiting to break in..." ("Value")) -> (s? t:f=w3336:T3)
        n1188 = property class="Arr (strict)"(reference=w3340, "Value"=w3331) -> ()  [unwired: 1 in, 2 out]
        n1189 = property class="Arr (strict)"(reference=w3327, "Value"=w3326) -> ()  [unwired: 1 in, 2 out]
        n1190 = call "gigaseal_checker.vi"("default val in beginning"=TRUE, "num elements to look at"=5, "gigasealing array"=w3331) -> ("Gigaseal?"=w3329:bool)  [unwired: 8 in]
        n1191 = call "gigaseal_checker.vi"("default val in beginning"=TRUE, "num elements to look at"=20, "gigasealing array"=w3331) -> ("Gigaseal?"=w3330:bool)  [unwired: 8 in]
        n1192 = Or(x=w3329, y=w3330) -> (x .or. y?=w3328:bool)
        n1193 = Select(t=w3336, s=w3328, f=user_message_v6."Unsuccessful breakin!" ("Value")) -> (s? t:f=w3335:T3)
      }
      frame "Waiting for WC" {
        w3363 = user_message_v6."Retracting pipette..." ("Value")
        # "if other pipette is retracting,\nclear WC LED after WC"
        # "the pipette spends time here during whole cell"
        n1194 = Unbundle By Name(w3367) -> ("misc indiv.other state ref"=w3366:refnum<vi>)
        n1195 = Wait (ms)(milliseconds to wait=u32 100) -> ()  [unwired: 1 out]
        n1196 = property on="Property Node" class="Enum (strict)"(reference=w3366) -> ("Value"=w3368:T3)  [unwired: 1 in, 2 out]
        n1197 = Equal?(x=w3368, y=w3363) -> (x = y?=w3361:bool)
        n1198 = Select(t=w3363, s=w3361, f=user_message_v6."Waiting for WC" ("Value")) -> (s? t:f=w3364:T3)
        n1199 = case shown="True" w3361 {
          tunnel: w3360 -> [_ w3370]
          tunnel: w3359 -> [_ w3369]
          frame False {
          }
          frame True {
            n1200 = call "wcLED_topLvl.vi"("which manipulator"=w3370, "wc LED"=FALSE, "Pressure box control in"=w3369) -> ()  [unwired: 7 in, 2 out]
          }
        }
      }
      frame "Done with Current Set of Cells" {
      }
    }
    "state out" <- w33
    "error out" <- w64
    "exit trigger" <- w43
    n1201 = call "saveStateTiming_HEK-v02.vi"("current state"=w33, "previous state"=w34, "state times"=w60, "state list"=w61, "previous time in"=w63) -> ("previous time out"=w62:timestamp)  [unwired: 6 in]
    n1202 = property class="Enum (strict)"(reference=w58, "Value"=w33) -> ()  [unwired: 1 in, 2 out]
  }
